vi "fly dominator.vi"() -> ()   [LabVIEW 2021]
uses:
  states.ctl
  <vilib>/Analysis/NI_AALBase.lvlib
  <vilib>/Analysis/baseanly.llb/Mean (DBL).vi
  <extravilib>/ChannelInstances/Tag-bool.lvlib
  <vilib>/DAQmx/write.llb/DAQmx Write (Digital Bool 1Line 1Point).vi
  <vilib>/DAQmx/create/channels.llb/DAQmx Create Channel (DO-Digital Output).vi
  <resource>/objmgr/daqmx.rc
  <vilib>/Waveform/WDTFileIO.llb/ Write Waveform to File.vi
  C:/FINDS_VIs/Thorlabs.MotionControl.Controls.dll
  FINDS_VIs/Thorlabs.MotionControl.Controls.dll
  C:/FINDS_VIs/Thorlabs.MotionControl.Benchtop.StepperMotorCLI.dll
  FINDS_VIs/Thorlabs.MotionControl.Benchtop.StepperMotorCLI.dll
  <vilib>/Analysis/NI_AALPro.lvlib
  0273469b-1630-426e-8888-91f9d245564e.vi
  8ea25fb4-7a89-4be8-837a-9bc05b844755.vi
  <vilib>/smtpClient/LabVIEWSMTPClient.lvlib
  a9b58a78-20d6-47fd-9184-b30837673e93.vi
  <vilib>/vision/NI_Vision_Development_Module.lvlib
  <vilib>/DAQmx/write.llb/DAQmx Write (Analog DBL 1Chan 1Samp).vi
  <vilib>/platform/TimedLoop/XDataNode/XDataNode.xnode
  <vilib>/Platform/TimedLoop/XDataNode/nitl_modes.ctl
  <vilib>/Platform/TimedLoop/XDataNode/XDNodeRunTimeDep.lvlib
  <vilib>/Platform/TimedLoop/XDataNode/wakeup.ctl
  <vilib>/Platform/TimedLoop/XDataNode/timing_clust.ctl
  <vilib>/DAQmx/read.llb/DAQmx Read (Digital Bool 1Line 1Point).vi
  <vilib>/DAQmx/create/channels.llb/DAQmx Create Channel (DI-Digital Input).vi
  <vilib>/DAQmx/create/channels.llb/DAQmx Create Channel (AO-Voltage-Basic).vi
  <vilib>/DAQmx/configure/timing.llb/DAQmx Timing (Sample Clock).vi
  <vilib>/DAQmx/create/channels.llb/DAQmx Create Channel (AI-Voltage-Basic).vi
  <vilib>/DAQmx/read.llb/DAQmx Read (Analog 1D DBL 1Chan NSamp).vi
  <vilib>/smtpClient/Set Message Text.vi
panel:
  out "Focal position":dbl
  in  "y 3":dbl
  in  "y 2":dbl
  in  "x":dbl
  in  "element 3":dbl=200.0
  in  "Focus changing \nperiod (ms)":dbl=3000.0
  out "relative seconds start":dbl format="%_19f"
  in  "4c":bool
  in  "Exposure time":dbl=0.0195
  in  "sample name":string="cance4r"
  out "Current state":string
  in  "Range 3":bool
  out "Last saved file 2":path
  out "Last saved # 2":i32
  in  "# to measure 2":i32=200
  out "Timed loop#":i32
  out "lateral position\n indexs":dbl[](array[numeric])
  out "647 2":bool
  out "647 i":bool
  in  "647?":bool
  in  "647 filter":dbl=0.2499999999999 format="%#_13g"
  in  "galvano":bool
  in  "647":bool
  in  "Slide":dbl(slide)=2.5059665871121717 scale=0.0..5.0
  out "405 2":bool
  out "488 2":bool
  out "594  2":bool
  out "532  2":bool
  in  "594 filter":dbl=0.3333333333333 format="%#_13g"
  in  "532 filter":dbl=0.4166667 format="%#_13g"
  in  "405 filter":dbl=0.16 format="%#_13g"
  in  "488 filter":dbl=0.08333333333333333 format="%#_13g"
  out "center":dbl format="%0.2f"
  in  "morphology\nthreshold":i32=40
  out "Numeric 8":i32
  in  "Setting 2":dbl=110.0
  in  "tube to stop":i32=6
  in  "maximum":i32=15
  out "larva size":bool
  out "r285":bool
  out "r216":bool
  out "Homing distance":u32
  in  "594?":bool
  in  "488?":bool
  in  "532?":bool
  in  "405?":bool
  in  "shower time":u32=20000
  in  "waiting time for\n robotic arm":u32=12000
  in  "washing time":u32=11000
  out "Boolean":bool
  out "Numeric 7":i32
  out "Numeric 6":i32
  out "Numeric 5":dbl
  out "waiting number":i32
  out "larvae in chamber?":bool
  in  "Range 2":bool
  out "4c label #":i32
  in  "batch#":string
  in  "High speed?":bool
  out "max value":i32
  out "real R2":i32
  in  "clearing date":string
  in  "laser channel":string
  in  "wait for\nclearing":bool
  in  "wait for clearing? 2":bool
  out "clear finished?":bool
  out "relative seconds 2":dbl format="%_19f"
  in  "real laser power":string
  in  "Operator":T1(ring)=enum."hanqing WANG"
  in  "max intensity threshold":i32=3500
  out "screening":bool
  in  "4000?":bool
  in  "calibration?":bool
  out "experiment time(mins)":dbl
  out "experiment stop time (relative)":dbl format="%_19f"
  in  "screening method":T2(ring)=enum."Pix count"
  in  "Count threshold":dbl
  in  "2000?":bool=TRUE
  out "Numeric 4":i32
  out "index":i32
  out "size(s)":i32
  out "Frame 2":i32
  out "mean 5":dbl format="%0.2f"
  out "mean 4":dbl format="%0.2f"
  out "Numeric 2":i32
  in  "manual loading":bool
  in  "shower time(ms)":u32=5000
  in  "BUBBLE SIZE":i32=3
  out "gp":dbl
  in  "um to move short":u32=6500
  in  "um to move long":u32=7000
  out "OK Done 4":bool
  out "homing speed":bool
  out "homing":bool
  in  "4c direction":bool=TRUE
  in  "manual 4c":bool
  out "tube changing #":i32
  in  "# BEFORE GO DOWN":i32=1
  in  "TIME THRESHOLD":dbl=40.0
  in  "force anticlogging":bool
  in  "Flow Rate (5.00)":dbl=100.0 format="%#.4f"
  in  "milliseconds to wait":u32=4000
  in  "position":dbl=0.083333
  out "#of edgehunting":u32
  in  "wavelength":string
  out "Auto-imaging time":dbl[](graph)
  in  "4c Base file name":string="brp_each"
  out "594 i":bool
  out "532 i":bool
  out "488 i":bool
  out "405 i":bool
  out "Last saved file 4c":path
  in  "BenchtopStepperControl":refnum<k24>(container)
  in  "SerialNumber":string="40227394"
  in  "Frames in memory 2":i32=800
  in  "High Speed 2":u32=10000
  out "Larva length (# frames)":i32
  in  "correction":i32=600
  out "backwards pulses":i32
  in  "scanning Speed":u32=20000 min=1 max=500000
  out "larvae size in scan":dbl[](graph)
  out "OK Done":bool
  in  "Edge-hunting Direction":bool
  in  "scanning distance (um)":u32=43000 min=1 max=500000
  in  "Main/Sub":bool
  in  "manual edgehunting":bool
  in  "Number of samples":i32=150
  out "Waveform Graph":dbl[](graph)
  out "loading tube#":i32
  in  "manual load":bool
  in  "Force move":bool
  in  "Larva # to move":i32=1000
  out "Larvae until move":i32
  in  "tb Pulses to move":u32=750 min=1 max=500000
  in  "tube Direction":bool
  in  "Save start #":i32
  out "Last saved file number 4":i32
  in  "Enable screening\n(during flow zoometry)":bool
  in  "Save base file name 2000":path=path "\\\\FINDSCTRL\\findsdata/finds2/20240321/2000test"
  in  "Acquire speed 3 (um/s)":u32=2000
  out "Last saved file 2000":path
  out "Last saved file number 2000":i32
  in  "Samples to measure 2000":i32=100
  in  "EH speed 3":bool
  out "Mean intensity\nof frame":dbl=212.9530098438263 format="%0.2f"
  in  "reverse":bool
  in  "wave trigger":dbl
  in  "Save base file name 4000":path=path "\\\\157.82.9.50\\d/20240220/gp mor/tm6b/4000/uasmcherry.tm6b.2.50w.4000"
  in  "Acquire speed 2 (um/s)":u32=4000
  out "Last saved file 4000":path
  in  "Samples to measure 4000":i32=100
  in  "EH speed 2":bool
  in  "reverse flow \nthreshold (sec)":dbl=40.0
  out "Elapsed (sec)":dbl
  in  "next loop":bool=TRUE
  out "False triggers":i32
  in  "manual imaging":bool
  in  "SampClk.Rate 2":dbl=100000.0
  in  "Physical Channel 2":tag="Dev1/ai0"
  in  "Stop Trigger stream":bool
  out "Mean":dbl format="%0.2f"
  out "Triggered":bool
  in  "Trigger":dbl=0.10000000000000009
  out "Trigger PD running mean":dbl(graph)
  out "#triggers":i32
  in  "um to move":u32=6000
  in  "488":bool
  in  "532":bool
  in  "594":bool
  in  "405":bool
  in  "START AUTO IMAGING":bool caption="Start\nauto imaging"
  in  "Continuous\nacquisition":bool
  in  "# to measure":i32=200
  out "Last saved #":i32
  out "Last saved file":path
  in  "Acquire speed (um/s)":u32=200
  in  "Movement direction":bool=TRUE
  out "Saving image":bool
  out "Moving":bool
  in  "Save directory":path=path "\\\\157.82.9.50\\d/HW/b11 cance4r"
  in  "Mean trigger":i32=170
  out "Sub img mean":dbl
  out "Sub image":u16[][](graph) caption="Image"
  in  "XS x length":i32=1000
  in  "XS x px start":i32=500
  out "READY":bool
  in  "Shut down":bool
  in  "START":bool
  out "Streaming":bool
  in  "XS y length":i32=1000
  in  "XS y px start":i32=1000
  out "Camera error out":errorcluster {"code" format="%.0x"}
  in  "Quit":bool
  out "Obtained image":u16[][](graph) caption="Image"
  out "Frame count":i32
  # "error trigger exclusion setting"
  # "NOTICE:\nplease check the state frequently\nyou have to go back to chilling state before you do any other operation"
  # "File & save settings"
  # "motion tracker"
  # "Status"
  # "Laser output\n(Chilling state updates)"
  # "Flow zoometry"
  # "Trigger"
  # "No-flow imaging"
  # "Camera streaming"
  # "Genetic screening"
  # "Acquisition settings"
  # "Auto\nfocus settings"
  # "Sucking tube settings"
  # "Manual image acquisition\n(initiate from chilling state)"
  # "down"
  # "up"
  # "Edgehunting settings"
  # "Anti-clogging settings"
  # "ROBOTIC ARM LOADING"
  # "B"
  # "F"
  # "channel selection"
types:
  T1 = enum16{"kobayashi", "Tsutsumi", "hanqing WANG", "chenglang"}
  T2 = enum16{"morphology", "Pix count", "MAX INTENSITY", "Average int"}
  T3 = enum32{"Invalid", "Standard", "Closed", "Hidden", "Minimized", "Maximized"}
  T4 = typedef "states.ctl" = enum16{"acquire without AF", "647", "Initialize", "Chilling", "4climbo", "light reverse", "wait for clearing", "manual loading", "4cini", "reverse", "2000", "4000", "screening", "tube position", "Edgehunting", "Edgehunting2", "homing", "Position_check", "antic\n", "Stream w/o flow2", "Stream w/o flow", "stopflow triggertest", "Find boundaries", "Acquire", "save", "auto imaging", "robotic arm", "Close", "594", "532", "488", "405", "4c acquirement", "Stop", "405_r"}
  T5 = enum32{"Map Pixel Pointer", "Unmap Pixel Pointer", "Get Pixels Infos"}
  T6 = typedef "XDNodeRunTimeDep.lvlib/timing_clust.ctl" = cluster{"Expected End [f-1]":u64, "Actual End [f-1]":u64, "Finished Late? [f-1]":bool, "Expected End [i-1]":u64, "Actual End [i-1]":u64, "Finished Late? [i-1]":bool, "Expected Start [i]":u64, "Actual Start [i]":u64, "Expected Start [f]":u64, "Actual Start [f]":u64, "Source Name":string, "Structure Name":string, "Period":i64, "Deadline":i64, "Offset":i64, "Start":i64, "Priority":i32, "Timeout":i32, "Mode":T7, "Wakeup Reason":T8, "Error":errorcluster, "Source Type":string, "Secondary Source Type":string, "Global End Time":u64, "Global Start Time":u64, "Frame Duration":u64, "Iteration Duration":u64, "Assigned CPU":i32, "I/O Scan Engine Mode":u32}
  T7 = typedef "XDNodeRunTimeDep.lvlib/nitl_modes.ctl" = enum32{"No Change", "Process missed periods, maintain original phase", "Discard missed periods, maintain original phase", "Process missed periods, ignore original phase", "Discard missed periods, ignore original phase"}
  T8 = typedef "XDNodeRunTimeDep.lvlib/wakeup.ctl" = enum32{"Normal", "Aborted", "Asynchronous wakeup", "Timing source error", "Timed loop error", "Timeout"}
  T9 = cluster{"Output Trigger Mode":u32, "Output Trigger Polarity":u32}
  T10 = cluster{"Output Trigger Period":dbl, "Delay":dbl, "Source":u32}
  T11 = typedef "Image Type" = u32
  T12 = typedef "IMAQ Image.ctl" = refnum<image>
  T13 = typedef "Tag-bool.lvlib/))Channel.ctl" = refnum<queue>
  T14 = typedef "LabVIEWSMTPClient.lvlib/SmtpClientHandle.ctl" = refnum<k1>
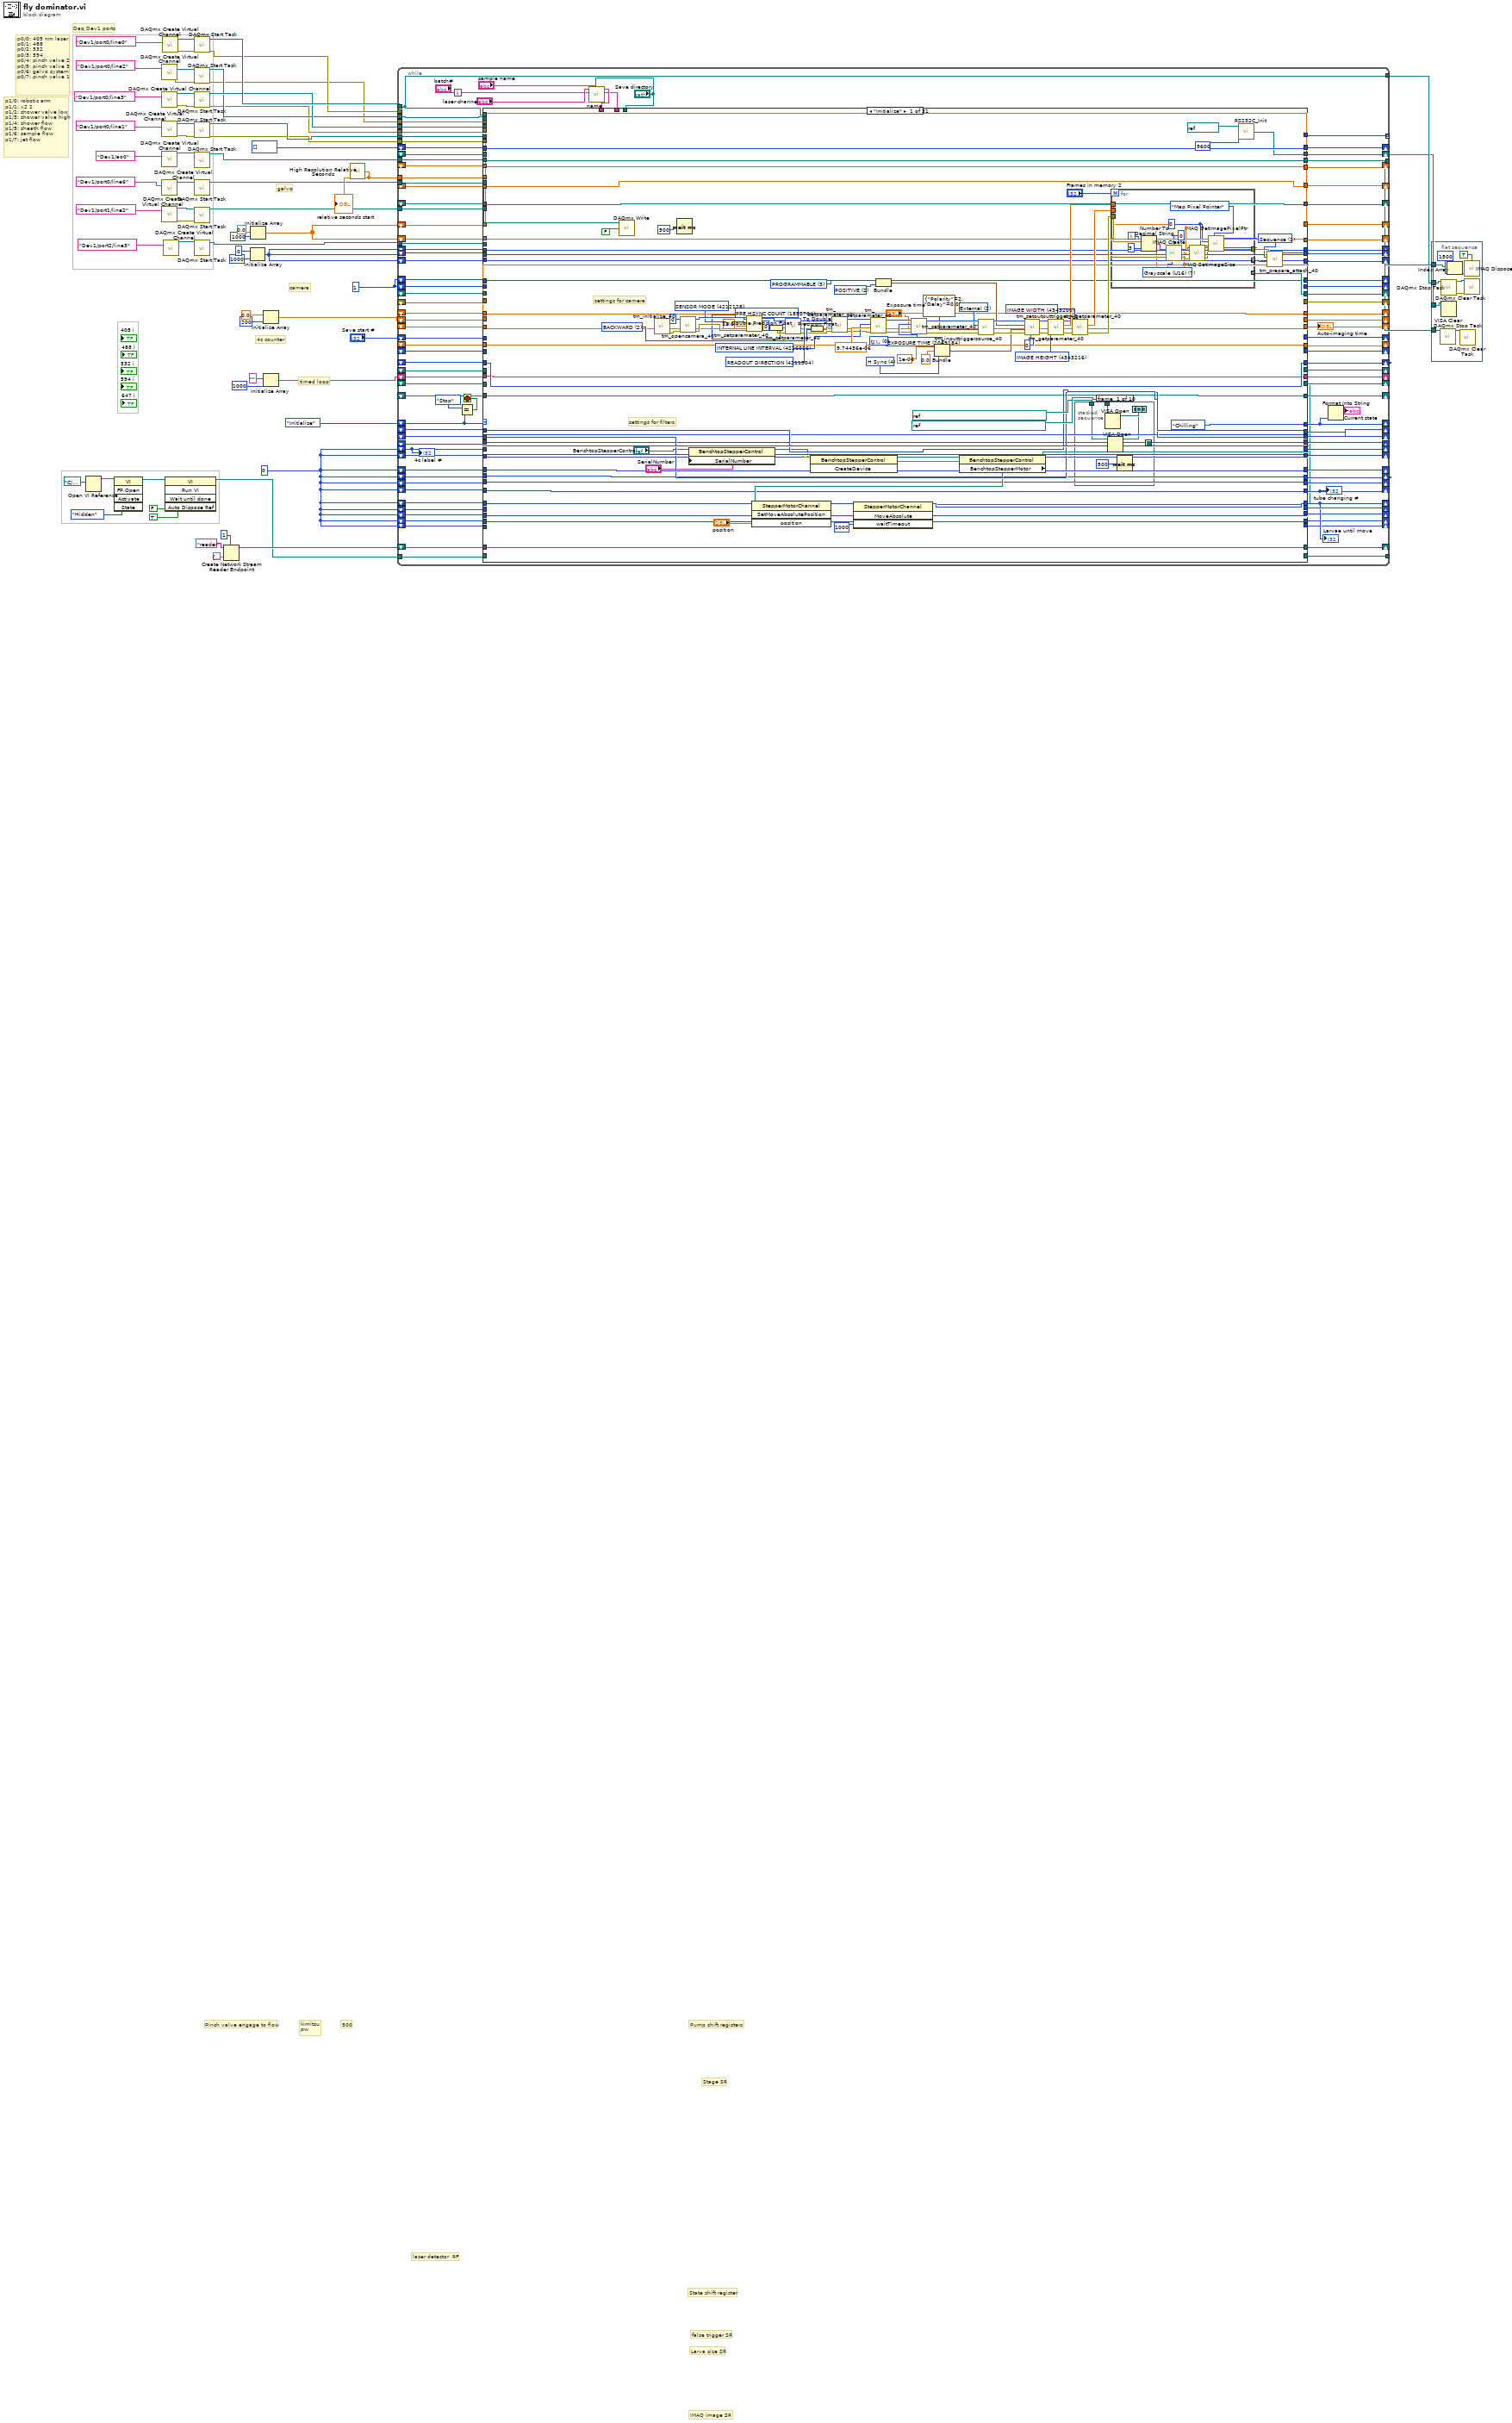
[diagram p0: block diagram]
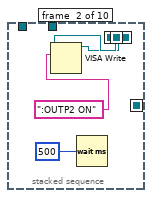
[diagram p2: hidden frame]
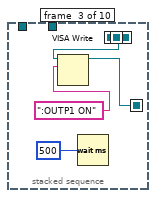
[diagram p3: hidden frame]
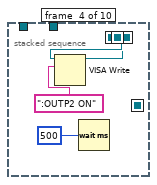
[diagram p4: hidden frame]
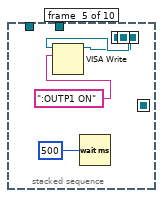
[diagram p5: hidden frame]
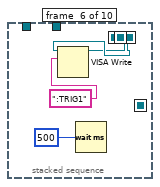
[diagram p6: hidden frame]
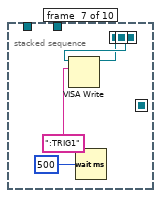
[diagram p7: hidden frame]
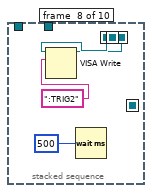
[diagram p8: hidden frame]
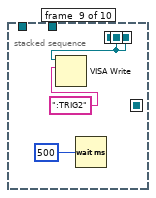
[diagram p9: hidden frame]
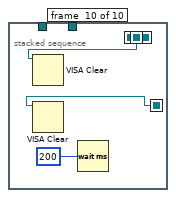
[diagram p10: hidden frame]
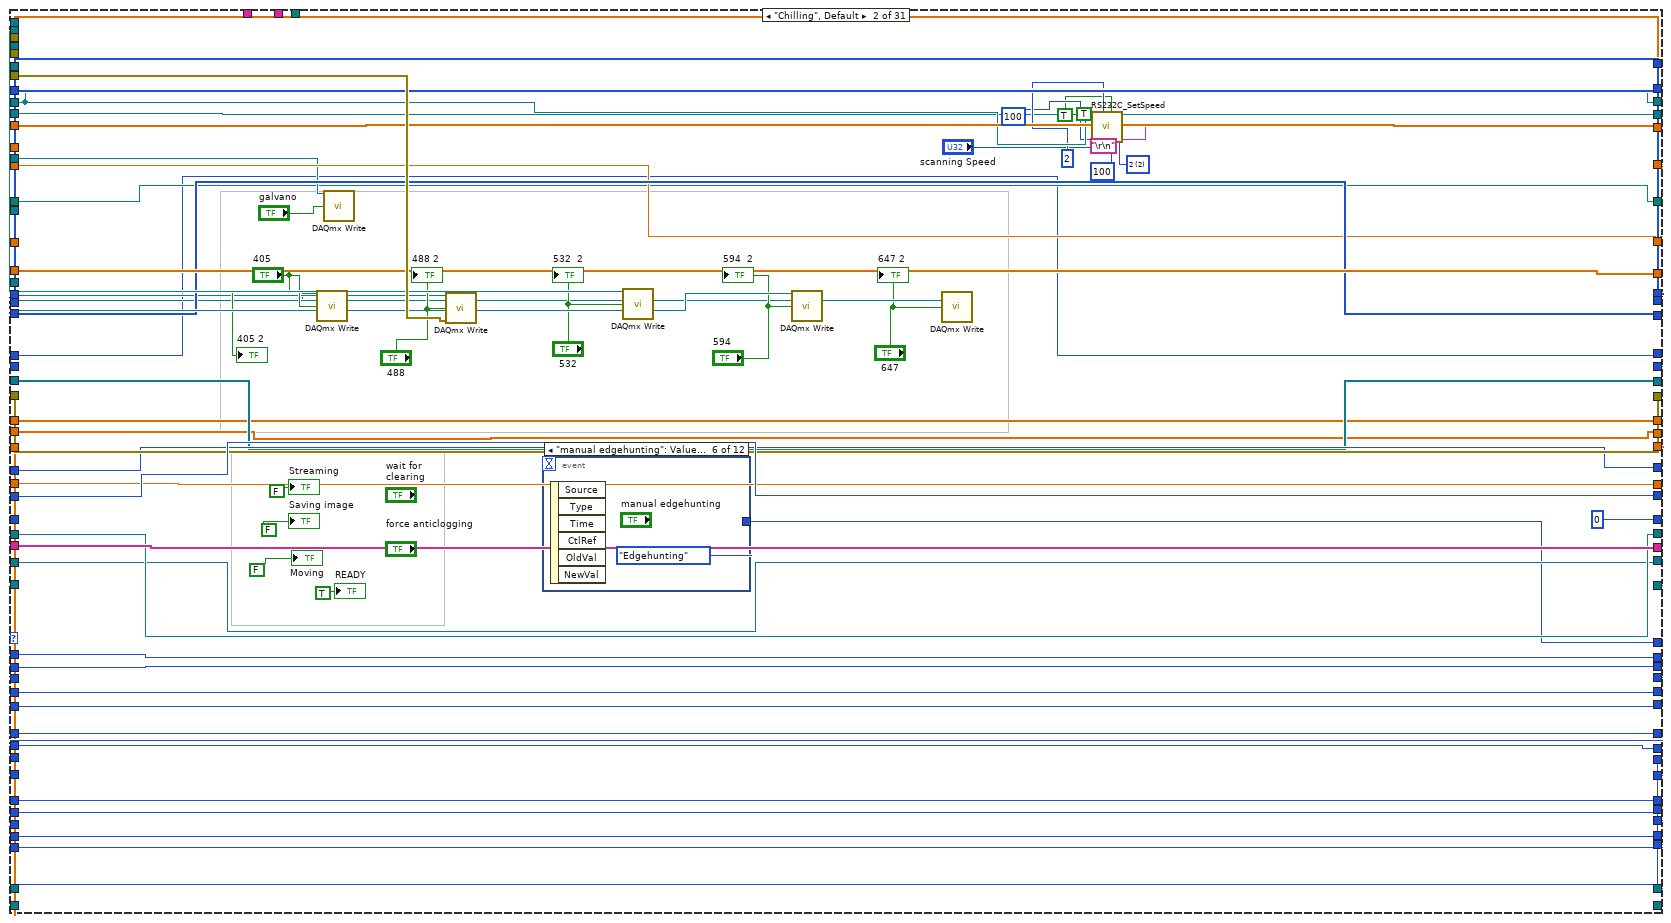
[diagram p11: hidden frame]
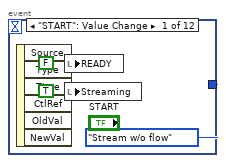
[diagram p12: hidden frame]
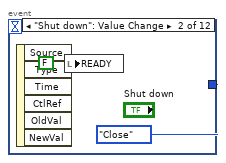
[diagram p13: hidden frame]
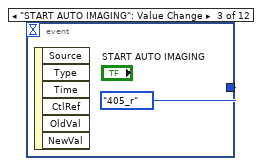
[diagram p14: hidden frame]
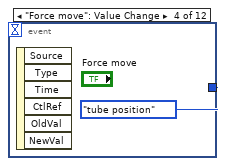
[diagram p15: hidden frame]
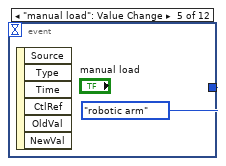
[diagram p16: hidden frame]
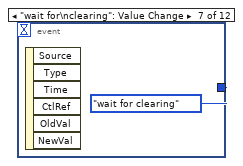
[diagram p17: hidden frame]
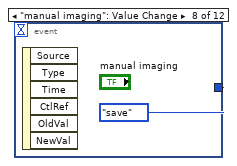
[diagram p18: hidden frame]
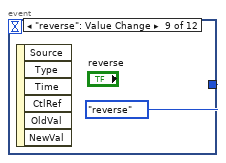
[diagram p19: hidden frame]
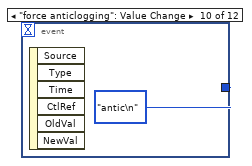
[diagram p20: hidden frame]
diagram:
  w4 = 1
  w5 = 0
  # "p0/0: 405 nm laser \np0/1: 488\np0/2: 532\np0/3: 594\np0/4: pinch valve 2\np0/5: pinch valve 3\np0/6: galvo system \np0/7: pinch valve 1"
  # "p1/0: robotic arm\np1/1: v2 2\np1/2: shower valve low\np1/3: shower valve high\np1/4: shower flow\np1/5: sheath flow\np1/6: sample flow\np1/7: jet flow"
  # "timed loop"
  # "Daq Dev1 ports"
  # "galvo"
  # "4c counter"
  # "500"
  # "false trigger SR"
  # "camera"
  # "kimitsu\npw"
  # "laser detector  RF"
  # "IMAQ image SR"
  # "Larva size SR"
  # "Stage SR"
  # "Pinch valve engage to flow"
  # "State shift register"
  # "Pump shift registers"
  n1 = Open VI Reference(vi path=path "C:/FINDS_VIs/Abyss-watcher_love-edition.vi") -> (vi reference=w27:refnum<vi>)  [unwired: 5 in, 1 out]
  n2 = invoke class="VI" method="FP.Open"(reference=w27, "State"=T3."Hidden") -> (reference out=w25:refnum<vi>)  [unwired: 3 in, 4 out]
  n3 = call-poly <vilib>:"DAQmx Create Virtual Channel.vi"("lines"=tag "Dev1/port0/line2") -> ("task out"=w49:refnum<k21>, "error out"=w58:errorcluster)  [unwired: 13 in]
  n4 = call-poly <vilib>:"DAQmx Create Virtual Channel.vi"("lines"=tag "Dev1/port0/line3") -> ("task out"=w52:refnum<k21>, "error out"=w56:errorcluster)  [unwired: 13 in]
  n5 = call-poly <vilib>:"DAQmx Create Virtual Channel.vi"("lines"=tag "Dev1/port0/line1") -> ("task out"=w61:refnum<k21>, "error out"=w54:errorcluster)  [unwired: 13 in]
  n6 = call-poly <vilib>:"DAQmx Create Virtual Channel.vi"("physical channels"=tag "Dev1/ao0") -> ("task out"=w12:refnum<k21>)  [unwired: 13 in, 1 out]
  n7 = call-poly <vilib>:"DAQmx Create Virtual Channel.vi"("lines"=tag "Dev1/port0/line6") -> ("task out"=w9:refnum<k21>)  [unwired: 13 in, 1 out]
  n8 = call-poly <vilib>:"DAQmx Create Virtual Channel.vi"("lines"=tag "Dev1/port1/line2") -> ("task out"=w33:refnum<k21>, "error out"=w31:errorcluster)  [unwired: 13 in]
  n9 = call-poly <vilib>:"DAQmx Create Virtual Channel.vi"("lines"=tag "Dev1/port0/line0") -> ("task out"=w65:refnum<k21>, "error out"=w64:errorcluster)  [unwired: 13 in]
  n10 = call-poly <vilib>:"DAQmx Create Virtual Channel.vi"("lines"=tag "Dev1/port2/line3") -> ("task out"=w17:refnum<k21>)  [unwired: 13 in, 1 out]
  n11 = invoke class="VI" method="Run VI"(reference=w25, "Wait until done"=FALSE ("Wait Until Done"), "Auto Dispose Ref"=TRUE ("Auto Dispose Reference")) -> (reference out=w3:refnum<vi>)  [unwired: 2 in, 4 out]
  n12 = call <vilib>:"DAQmx Start Task.vi"("task/channels in"=w49, "error in"=w58) -> ("task out"=w50:refnum<k21>, "error out"=w43:errorcluster)  [unwired: 12 in]
  n13 = call <vilib>:"DAQmx Start Task.vi"("task/channels in"=w52, "error in"=w56) -> ("task out"=w51:refnum<k21>, "error out"=w42:errorcluster)  [unwired: 12 in]
  n14 = call <vilib>:"DAQmx Start Task.vi"("task/channels in"=w61, "error in"=w54) -> ("task out"=w59:refnum<k21>, "error out"=w53:errorcluster)  [unwired: 12 in]
  n15 = call <vilib>:"DAQmx Start Task.vi"("task/channels in"=w12) -> ("task out"=w11:refnum<k21>)  [unwired: 13 in, 1 out]
  n16 = call <vilib>:"DAQmx Start Task.vi"("task/channels in"=w9) -> ("task out"=w8:refnum<k21>)  [unwired: 13 in, 1 out]
  n17 = call <vilib>:"DAQmx Start Task.vi"("task/channels in"=w65, "error in"=w64) -> ("task out"=w62:refnum<k21>, "error out"=w48:errorcluster)  [unwired: 12 in]
  n18 = call <vilib>:"DAQmx Start Task.vi"("task/channels in"=w33, "error in"=w31) -> ("task out"=w30:refnum<k21>)  [unwired: 12 in, 1 out]
  n19 = call <vilib>:"DAQmx Start Task.vi"("task/channels in"=w17) -> ("task out"=w16:refnum<k21>)  [unwired: 13 in, 1 out]
  n20 = Create Network Stream Reader Endpoint(7:1 ("reader buffer size"), 9:cluster{dbl, bool} {0.0, TRUE}, 11:"reader" ("reader name")) -> (3:w20:refnum<k21>)  [unwired: 4 in, 1 out]
  n21 = Initialize Array(i16 0 ("element"), 1000 ("dimension size")) -> (w1:i16[])
  n22 = Initialize Array(0.0 ("element"), 1000 ("dimension size")) -> (w7:dbl[])
  n23 = Initialize Array("", 1000 ("dimension size")) -> (w44:string[])
  n24 = Initialize Array(0.0 ("element"), 200 ("dimension size")) -> (w6:dbl[])
  n25 = call <vilib>:"High Resolution Relative Seconds.vi"() -> ("relative seconds"=w36:dbl)
  "relative seconds start" <- w36
  n26 = while {
    shift-right: [w73] -> _
    shift-left: states."Initialize" -> [w173]
    shift-right: [w170] -> _
    shift-left: _ -> [w168]
    shift-right: [w169] -> _
    shift-left: _ -> [w167]
    shift-right: [w165] -> _
    shift-left: "Save start #" -> [w166]
    shift-right: [w164] -> _
    shift-left: _ -> [w163]
    shift-right: [w98] -> w29
    shift-left: _ -> [w162]
    shift-right: [w161] -> _
    shift-left: _ -> [w160]
    shift-right: [w159] -> w47
    shift-left: _ -> [w158]
    tunnel: w62 -> [w107]
    tunnel: w59 -> [w157]
    tunnel: w53 -> [w156]
    tunnel: w51 -> [w154]
    tunnel: w50 -> [w155]
    tunnel: [w107] -> w37
    tunnel: w48 -> [_]
    shift-right: [w152] -> _
    shift-left: w5 -> [w153]
    shift-right: [w132] -> _
    shift-left: w7 -> [w151]
    shift-right: [w111] -> _
    shift-left: w6 -> [w150]
    shift-right: [w148] -> _
    shift-left: w44 -> [w149]
    shift-right: [w146] -> _
    shift-left: w5 -> [w147]
    shift-right: [w144] -> _
    shift-left: i32[] [] -> [w145]
    shift-right: [w142] -> _
    shift-left: w1 -> [w143]
    shift-right: [w131] -> _
    shift-left: _ -> [w141]
    shift-right: [w139] -> _
    shift-left: w4 -> [w140]
    shift-right: [w137] -> _
    shift-left: w1 -> [w138]
    tunnel: w43 -> [w136]
    tunnel: w42 -> [w135]
    shift-right: [w133] -> _
    shift-left: w1 -> [w134]
    shift-right: [w129] -> _
    shift-left: w4 -> [w130]
    shift-right: [w127] -> _
    shift-left: w5 -> [w128]
    shift-right: [w126] -> _
    shift-left: w5 -> [w125]
    tunnel: [w124] -> _ mode=indexing
    shift-right: [w122] -> _
    shift-left: w5 -> [w123]
    shift-right: [w87] -> _
    shift-left: _ -> [w119]
    shift-right: [w121] -> _
    shift-left: _ -> [w117]
    shift-right: [w120] -> _
    shift-left: _ -> [w118]
    shift-right: [w116] -> _
    shift-left: _ -> [w114]
    shift-right: [w115] -> _
    shift-left: _ -> [w75]
    tunnel: w36 -> [w113]
    shift-right: [w110] -> _
    shift-left: w6 -> [w112]
    shift-right: [w108] -> _
    shift-left: w5 -> [w109]
    tunnel: w30 -> [w106]
    tunnel: [w105] -> _
    shift-right: [w103] -> _
    shift-left: w5 -> [w104]
    shift-right: [w101] -> _
    shift-left: w5 -> [w102]
    shift-right: [w99] -> _
    shift-left: w6 -> [w100]
    shift-right: [w96] -> _
    shift-left: w5 -> [w97]
    shift-right: [w95] -> _
    shift-left: w20 -> [w94]
    tunnel: w3 -> [w93]
    shift-right: [w91] -> _
    shift-left: w5 -> [w92]
    shift-right: [w90] -> _
    shift-left: _ -> [w89]
    tunnel: w16 -> [w88]
    shift-right: [w85] -> _
    shift-left: w7 -> [w86]
    shift-right: [w83] -> _
    shift-left: w5 -> [w84]
    tunnel: w11 -> [w82]
    tunnel: [w81] -> w13
    tunnel: w8 -> [w80]
    shift-right: [w79] -> _
    shift-left: _ -> [w78]
    shift-right: [w77] -> _
    shift-left: _ -> [w76]
    stop <- w172 stop-if-true
    n27 = Equal?(x=w173, y=states."Stop") -> (x = y?=w172:bool)
    n28 = call "name.vi"("sample name"="sample name", "Save directory"="Save directory", "batch#"="batch#", "laser channel"="laser channel") -> ("time stamp"=w72:string, "file naming"=w71:string)  [unwired: 5 in, 1 out]
    n29 = case shown="\"Initialize\"" w173 {
      tunnel: [w232 w413 w482 w535 w630 w969 w1057 w1355 w1471 w1591 w1885 w1969 w2219 w2397 w2602 w2848 w3081 w3281 w3349 w3417 w3486 w3548 w3616 w3684 w3734 w3827 w4035 w4186 w4447 u32 0 ("Handle out") u32 0 ("Handle out")] -> w170
      tunnel: [w235 w412 w481 w536 w632 w968 w1056 w1354 w1470 w1590 w1884 w1967 w2218 w2396 w2600 w2846 w3079 w3280 w3348 w3416 w3485 w3547 w3615 w3683 w3733 w3826 w4034 w4185 w4446 errorcluster {"status"=FALSE, "code"=0, "source"=""} ("error out") errorcluster {"status"=FALSE, "code"=0, "source"=""} ("error out")] -> w169
      tunnel: [states."Chilling" w367 w451 states."Chilling" w633 w952 w1045 w1328 w1444 w1546 w1814 w2032 w2193 w2398 states."acquire without AF" w2880 w3110 w3247 w3315 w3383 w3453 w3514 w3582 w3650 w3701 w3859 w4042 w4151 w4454 states."Stop" states."Stop"] -> w73
      tunnel: w168 -> [_ w413 w482 w497 w630 w969 w1057 w1355 w1471 w1591 w1885 w1974 w2219 w2397 w2643 w2890 w3120 w3281 w3349 w3417 w3486 w3548 w3616 w3684 w3734 w3870 w4055 w4186 w4466 w4628 _]
      tunnel: w167 -> [_ w412 w481 w533 w632 w968 w1056 w1354 w1470 w1590 w1884 w1973 w2218 w2396 w2644 w2891 w3121 w3280 w3348 w3416 w3485 w3547 w3615 w3683 w3733 w3871 w4056 w4185 w4467 w4627 _]
      tunnel: w166 -> [w245 w411 w480 w540 w634 w967 w1055 w1353 w1469 w1589 w1883 w1938 w2217 w2395 w2556 w2788 w3032 w3279 w3347 w3415 w3484 w3546 w3614 w3682 w3732 w3815 w3995 w4184 w4405 w4623 w4729]
      tunnel: [w245 w411 w480 w540 w634 w967 w1055 w1353 w1469 w1589 w1883 w1938 w2217 w2395 w2612 w2788 w3031 w3279 w3347 w3415 w3484 w3546 w3614 w3682 w3732 w3814 w3995 w4184 w4405 w4623 w4729] -> w165
      tunnel: [w179 w410 w432 w539 w576 w925 w984 w1291 w1407 w1517 w1807 w1958 w2170 w2353 w2642 w2889 w3119 w3227 w3296 w3364 w3431 w3494 w3563 w3631 w3692 w3869 w4054 w4141 w4465 refnum<visa-resource-name> refnum ("VISA resource name out") refnum<visa-resource-name> refnum ("VISA resource name out")] -> w164
      tunnel: w163 -> [w179 w410 w432 w539 w576 w925 w984 w1291 w1407 w1517 w1807 w1958 w2170 w2353 w2642 w2889 w3119 w3227 w3296 w3364 w3431 w3494 w3563 w3631 w3692 w3869 w4054 w4141 w4465 _ _]
      tunnel: [w206 w388 w479 w538 w631 w966 w1044 w1352 w1468 w1588 w1882 w2017 w2199 w2371 w2631 w2876 w3107 w3278 w3346 w3414 w3483 w3545 w3613 w3681 w3731 w3856 w4037 w4183 w4449 w4621 w4727] -> w98
      tunnel: w162 -> [_ w388 w479 w538 w631 w966 w1044 w1352 w1468 w1588 w1882 w2031 w2201 w2371 w2641 w2888 w3118 w3278 w3346 w3414 w3483 w3545 w3613 w3681 w3731 w3868 w4053 w4183 w4464 w4621 w4727]
      tunnel: [w224 u32 0 w478 w528 w625 w965 w1036 w1351 w1467 w1587 w1881 w2044 w2216 w2400 w2618 w2863 w3095 w3277 w3345 w3413 w3482 w3544 w3612 w3680 w3730 w3845 w4021 w4182 w4386 w4616 w4723] -> w161
      tunnel: w160 -> [w224 _ w478 w528 w625 w965 w1036 w1351 w1467 w1587 w1881 w2044 w2216 w2400 w2618 w2863 w3095 w3277 w3345 w3413 w3482 w3544 w3612 w3680 w3730 w3845 w4021 w4182 w4386 w4616 w4723]
      tunnel: "Save directory" -> [_ _ _ _ _ _ _ _ _ _ _ w1935 _ _ w2529 w2882 w3111 _ _ _ _ _ _ _ _ w3861 _ _ _ _ _]
      tunnel: [w229 w408 w477 w532 w629 w964 w1054 w1350 w1466 w1586 w1880 w2021 w2215 w2344 w2629 w2874 w3105 w3276 w3344 w3412 w3481 w3543 w3611 w3679 w3729 w3853 w4032 w4181 w4444 w4620 w4664] -> w159
      tunnel: w158 -> [_ w408 w477 w534 w629 w964 w1054 w1350 w1466 w1586 w1880 w2026 w2215 w2344 w2629 w2874 w3105 w3276 w3344 w3412 w3481 w3543 w3611 w3679 w3729 w3853 w4032 w4181 w4444 w4620 w4664]
      tunnel: w157 -> [_ w349 _ _ _ _ _ _ _ _ _ _ _ _ _ _ _ w3253 w3321 w3389 w3459 w3520 w3588 w3656 w3697 _ _ _ _ w4606 w4715]
      tunnel: w156 -> [_ w407 _ _ _ _ _ _ _ _ _ _ _ _ _ _ _ _ _ _ _ _ _ _ _ _ _ _ _ _ w4714]
      tunnel: w155 -> [_ w406 _ _ _ _ _ _ _ _ _ _ _ _ _ _ _ w3252 w3320 w3388 w3458 w3519 w3587 w3655 w3696 _ _ _ _ w4607 w4713]
      tunnel: w154 -> [_ w405 _ _ _ _ _ _ _ _ _ _ _ _ _ _ _ w3251 w3319 w3387 w3457 w3518 w3586 w3654 w3695 _ _ _ _ w4605 w4712]
      tunnel: w153 -> [w227 w401 w476 w531 w628 w963 w1053 w1349 w1465 w1585 w1879 w2043 w2214 w2394 w2616 w2861 w3093 w3275 w3343 w3411 w3480 w3542 w3610 w3678 w3728 w3843 w4019 w4180 w4431 w4619 w4726]
      tunnel: [w227 w401 w476 w531 w628 w963 w1053 w1349 w1465 w1585 w1879 w2043 w2214 w2393 w2616 w2861 w3093 w3275 w3343 w3411 w3480 w3542 w3610 w3678 w3728 w3843 w4019 w4180 w4431 w4619 w4726] -> w152
      tunnel: [w226 w400 w475 w530 w627 w962 w1052 w1348 w1464 w1584 w1878 w2042 w2213 w2392 w2597 w2843 w3072 w3274 w3342 w3410 w3479 w3541 w3609 w3677 w3727 w3832 w3977 w4179 w4403 w4618 w4725] -> w132
      tunnel: w151 -> [w226 w400 w475 w530 w627 w962 w1052 w1348 w1464 w1584 w1878 w2042 w2213 w2392 w2597 w2843 w3072 w3274 w3342 w3410 w3479 w3541 w3609 w3677 w3727 w3832 w3979 w4179 w4403 w4618 w4725]
      tunnel: w150 -> [w225 w399 w474 w529 w626 w961 w1051 w1347 w1463 w1583 w1877 w2009 w2212 w2391 w2596 w2842 w3071 w3273 w3341 w3409 w3478 w3540 w3608 w3676 w3726 w3831 w3984 w4178 w4429 w4617 w4724]
      tunnel: [w225 w399 w474 w529 w626 w961 w1051 w1347 w1463 w1583 w1877 w2008 w2212 w2391 w2596 w2842 w3071 w3273 w3341 w3409 w3478 w3540 w3608 w3676 w3726 w3831 w3984 w4178 w4428 w4617 w4724] -> w111
      tunnel: w149 -> [w223 w398 w473 w527 w623 w960 w1038 w1346 w1462 w1582 w1876 w2041 w2211 w2390 w2615 w2860 w3092 w3272 w3340 w3408 w3477 w3539 w3607 w3675 w3725 w3842 w4013 w4177 w4420 w4615 w4722]
      tunnel: w72 -> [_ _ _ _ _ _ _ _ _ _ _ _ _ _ w2614 w2859 w3091 _ _ _ _ _ _ _ _ w3841 w4017 _ w4426 _ _]
      tunnel: [w223 w398 w473 w527 w623 w960 w1038 w1346 w1462 w1582 w1876 w2041 w2211 w2390 w2613 w2858 w3090 w3272 w3340 w3408 w3477 w3539 w3607 w3675 w3725 w3840 w4013 w4177 w4420 w4615 w4722] -> w148
      tunnel: w147 -> [w222 w397 w472 w526 w622 w959 w1037 w1345 w1461 w1581 w1875 w2040 w2210 w2389 _ _ _ w3271 w3339 w3407 w3476 w3538 w3606 w3674 w3724 w3820 _ w4176 _ w4614 w4721]
      tunnel: [w222 w397 w472 w526 w622 w959 w979 w1345 w1461 w1581 w1875 w2040 w2210 w2389 0 0 0 w3271 w3339 w3407 w3476 w3538 w3606 w3674 w3724 w3820 0 w4176 0 w4614 w4721] -> w146
      tunnel: w145 -> [w221 w396 w471 w525 w621 w958 w1033 w1344 w1460 w1580 w1874 w2039 w2209 w2388 w2611 w2857 w3089 w3270 w3338 w3406 w3475 w3537 w3605 w3673 w3723 w3839 w4016 w4175 w4425 w4613 w4720]
      tunnel: [w221 w396 w471 w525 w621 w958 w1033 w1344 w1460 w1580 w1874 w2039 w2209 w2388 w2611 w2857 w3089 w3270 w3338 w3406 w3475 w3537 w3605 w3673 w3723 w3839 w4016 w4175 w4425 w4613 w4720] -> w144
      tunnel: w143 -> [w220 w395 w470 w524 w620 w957 w1032 w1343 w1459 w1579 w1873 w1993 w2208 w2387 _ _ _ w3269 w3337 w3405 w3474 w3536 w3604 w3672 w3722 _ w4014 w4174 w4421 w4612 w4719]
      tunnel: [w220 w395 w470 w524 w620 w957 w1032 w1343 w1459 w1579 w1873 w1993 w2208 w2387 i16[] [] i16[] [] i16[] [] w3269 w3337 w3405 w3474 w3536 w3604 w3672 w3722 w3821 w4014 w4174 w4421 w4612 w4719] -> w142
      tunnel: [w219 w394 w469 w523 w619 w956 w1031 w1342 w1458 w1578 w1872 w2038 w2207 w2386 w2610 w2856 w3088 w3268 w3336 w3404 w3473 w3535 w3603 w3671 w3721 w3838 w3986 w4173 w4422 w4611 w4718] -> w131
      tunnel: w141 -> [w219 w394 w469 w523 w619 w956 w1031 w1342 w1458 w1578 w1872 w2038 w2207 w2386 w2610 w2856 w3088 w3268 w3336 w3404 w3473 w3535 w3603 w3671 w3721 w3838 w3986 w4173 _ w4611 w4718]
      tunnel: w140 -> [w218 w393 w468 w522 w618 w937 w1030 w1341 w1457 w1577 w1871 w2037 w2206 w2385 w2609 w2855 w3087 w3267 w3335 w3403 w3472 w3534 w3602 w3670 w3720 w3837 w3996 w4172 w4393 w4604 w4717]
      tunnel: [w218 w393 w468 w522 w618 w937 w1030 w1341 w1457 w1577 w1871 w2037 w2206 w2385 w2609 w2855 w3087 w3267 w3335 w3403 w3472 w3534 w3602 w3670 w3720 w3837 w3980 w4172 w4393 w4604 w4717] -> w139
      tunnel: w138 -> [w217 w392 w467 w521 w617 w955 w1029 w1340 w1456 w1576 w1870 w2036 w2198 w2384 w2608 w2854 w3086 w3266 w3334 w3402 w3471 w3533 w3601 w3669 w3719 w3821 w3994 w4171 w4399 w4603 w4716]
      tunnel: [w217 w392 w467 w521 w617 w955 w1029 w1340 w1456 w1576 w1870 w2036 w2198 w2384 w2608 w2854 w3086 w3266 w3334 w3402 w3471 w3533 w3601 w3669 w3719 w3821 w3993 w4171 w4399 w4603 w4716] -> w137
      tunnel: w136 -> [_ _ _ _ _ _ _ _ _ _ _ _ _ _ _ _ _ _ _ _ _ _ _ _ _ _ _ _ _ _ w4701]
      tunnel: w135 -> [_ _ _ _ _ _ _ _ _ _ _ _ _ _ _ _ _ _ _ _ _ _ _ _ _ _ _ _ _ _ w4698]
      tunnel: [w216 w391 w466 w520 w616 w954 w1028 w1339 w1455 w1575 w1869 w2035 w2205 w2383 w2607 w2853 w3085 w3265 w3333 w3401 w3470 w3532 w3600 w3668 w3718 w3836 w3987 w4170 w4401 w4602 w4696] -> w133
      tunnel: w134 -> [w216 w391 w466 w520 w616 w954 w1028 w1339 w1455 w1575 w1869 w2035 w2205 w2383 w2607 w2853 w3085 w3265 w3333 w3401 w3470 w3532 w3600 w3668 w3718 w3836 w3987 w4170 w4400 w4602 w4696]
      tunnel: w130 -> [w215 w348 w465 w519 w615 w953 w1027 w1338 w1454 w1574 w1868 w2034 w2204 w2362 w2606 w2852 w3084 w3264 w3332 w3400 w3469 w3531 w3599 w3667 w3717 w3835 w3985 w4169 w4369 w4601 w4695]
      tunnel: [w215 w348 w465 w519 w615 w953 w1027 w1338 w1454 w1574 w1868 w2034 w2204 w2362 w2606 w2852 w3084 w3264 w3332 w3400 w3469 w3531 w3599 w3667 w3717 w3835 w3985 w4169 w4370 w4601 w4695] -> w129
      tunnel: w71 -> [_ _ _ _ _ _ _ _ _ _ _ _ _ _ w2604 w2850 _ _ _ _ _ _ _ _ _ w3823 _ _ _ _ w4674]
      tunnel: w128 -> [w211 w390 w464 w518 w614 w933 w1003 w1337 w1453 _ w1867 w2033 w2203 w2382 w2594 w2789 w3068 w3263 w3331 w3399 w3468 w3530 w3598 w3666 w3716 w3817 w3976 w4168 w4388 w4586 w4694]
      tunnel: [w211 w390 w464 w518 w614 w933 w1003 w1337 w1453 0 ("Larva # to move") w1867 w2033 w2203 w2382 w2593 w2789 w3067 w3263 w3331 w3399 w3468 w3530 w3598 w3666 w3716 w3817 w3976 w4168 w4388 w4586 w4694] -> w127
      tunnel: [w210 w389 w463 w517 w613 w950 w1002 w1336 w1452 w1573 w1866 w2001 w2202 w2381 w2591 w2840 w3066 w3262 w3330 w3398 w3467 w3529 w3597 w3665 w3715 w3816 w3975 w4167 w4387 w4585 w4693] -> w126
      tunnel: w125 -> [w210 w389 w463 w517 w612 w950 w1002 w1336 w1452 w1573 w1866 w2001 w2202 w2381 w2591 w2840 w3066 w3262 w3330 w3398 w3467 w3529 w3597 w3665 w3715 w3816 w3975 w4167 w4387 w4585 w4693]
      tunnel: [_ _ _ _ w611 _ _ _ _ _ _ _ _ _ _ _ _ _ _ _ _ _ _ _ _ _ _ _ _ _ _] -> w124
      tunnel: w123 -> [w187 w369 w462 w507 w583 w934 w992 w1301 w1418 w1545 w1865 w1995 w2188 w2369 w2566 w2814 w3043 w3236 w3305 w3372 w3446 w3502 w3571 w3639 w3714 w3804 w3965 w4166 w4376 w4575 w4683]
      tunnel: [w187 w369 w462 w507 w583 w934 w992 w1301 w1418 w1524 w1865 w1995 w2188 w2369 w2566 w2814 w3043 w3236 w3305 w3372 w3446 w3502 w3571 w3639 w3714 w3804 w3965 w4166 w4376 w4575 w4683] -> w122
      tunnel: [w208 w380 w461 w515 w608 w948 w1000 w1335 w1451 w1543 w1864 w2019 w2200 w2361 w2585 w2834 w3038 w3261 w3329 w3397 w3466 w3528 w3596 w3664 w3713 w3812 w3973 w4165 w4384 w4583 w4691] -> w87
      tunnel: [w207 w379 w460 w514 w607 w947 w999 w1334 w1450 w1542 w1863 w2018 w2197 w2379 w2584 w2833 w3061 w3260 w3328 w3396 w3465 w3527 w3595 w3663 w3712 w3811 w3972 w4164 w4383 w4582 w4690] -> w121
      tunnel: [w209 w381 w459 w516 w609 w949 w1001 w1333 w1449 w1544 w1862 w2013 w2196 w2380 w2586 w2835 w3041 w3259 w3327 w3395 w3464 w3526 w3594 w3662 w3711 w3813 w3974 w4163 w4385 w4584 w4692] -> w120
      tunnel: w119 -> [w209 w381 w459 w516 w609 w949 w1001 w1333 w1449 w1544 w1862 _ w2196 w2380 w2586 w2835 w3041 w3259 w3327 w3395 w3464 w3526 w3594 w3662 w3711 w3813 w3974 w4163 w4385 w4584 w4692]
      tunnel: w118 -> [w208 w380 w461 w515 w608 w948 w1000 w1335 w1451 w1543 w1864 _ w2200 w2361 w2585 w2834 w3038 w3261 w3329 w3397 w3466 w3528 w3596 w3664 w3713 w3812 w3973 w4165 w4384 w4583 w4691]
      tunnel: w117 -> [w207 w379 w460 w514 w607 w947 w999 w1334 w1450 w1542 w1863 _ w2197 w2379 w2584 w2833 w3061 w3260 w3328 w3396 w3465 w3527 w3595 w3663 w3712 w3811 w3972 w4164 w4383 w4582 w4690]
      tunnel: [w197 w376 w458 w513 w606 w946 w998 w1332 w1448 w1541 w1861 w2011 w2195 w2378 w2582 w2831 w3056 w3258 w3326 w3394 w3463 w3525 w3593 w3661 w3710 w3810 w3971 w4162 w4382 w4581 w4689] -> w116
      tunnel: [w192 w375 w457 w512 w605 w945 w997 w1331 w1447 w1540 w1860 w2010 w2194 w2377 w2581 w2830 w3050 w3249 w3317 w3385 w3455 w3516 w3584 w3652 w3709 w3809 w3970 w4161 w4381 w4580 w4688] -> w115
      tunnel: w114 -> [_ w376 w458 w513 w606 w946 w998 w1332 w1448 w1541 w1861 w2011 w2195 w2378 w2582 w2831 w3056 w3258 w3326 w3394 w3463 w3525 w3593 w3661 w3710 w3810 w3971 w4162 w4382 w4581 w4689]
      tunnel: w75 -> [_ w375 w457 w512 w605 w945 w997 w1331 w1447 w1540 w1860 w2010 w2194 w2377 w2581 w2830 w3050 w3250 w3318 w3386 w3456 w3517 w3585 w3653 w3709 w3809 w3970 w4161 w4381 w4580 w4688]
      tunnel: w107 -> [_ w347 _ _ _ _ _ _ _ _ _ _ _ _ _ _ _ w3254 w3322 w3390 w3460 w3521 w3589 w3657 w3698 _ _ _ _ _ _]
      tunnel: w113 -> [_ _ _ _ _ _ _ _ _ _ _ _ _ _ _ _ _ _ _ _ _ _ _ _ _ _ _ _ _ _ _]
      tunnel: w112 -> [w196 w374 w456 w511 w604 w944 w996 w1330 w1446 w1539 w1859 w2005 w2192 w2376 w2580 w2829 w3049 w3242 w3310 w3378 w3451 w3508 w3577 w3645 w3708 w3808 w3969 w4160 w4380 w4579 w4687]
      tunnel: [w196 w374 w456 w511 w602 w944 w996 w1330 w1446 w1539 w1859 w2005 w2192 w2376 w2580 w2829 w3049 w3242 w3310 w3378 w3451 w3508 w3577 w3645 w3708 w3808 w3969 w4160 w4380 w4579 w4687] -> w110
      tunnel: w109 -> [w190 w373 w455 w510 w600 w943 w995 w1329 w1445 w1538 w1858 w2003 w2191 w2375 w2579 w2828 w3047 w3240 w3309 w3376 w3449 w3506 w3575 w3643 w3707 w3807 w3968 w4159 w4379 w4578 w4686]
      tunnel: [w190 w373 w455 w510 w600 w943 w995 w1329 w1445 w1538 w1858 w2002 w2191 w2375 w2579 w2828 w3047 w3240 w3309 w3376 w3449 w3506 w3575 w3643 w3707 w3807 w3968 w4159 w4379 w4578 w4686] -> w108
      tunnel: w106 -> [_ _ _ _ _ _ _ w1325 w1443 w1537 _ _ _ _ _ _ _ _ _ _ _ _ _ _ _ _ _ _ _ _ _]
      tunnel: [_ _ _ _ _ _ _ w1287 w1440 w1536 _ _ _ _ _ _ _ _ _ _ _ _ _ _ _ _ _ _ _ _ _] -> w105
      tunnel: w104 -> [w189 w371 w454 w509 w598 _ w994 w1313 w1430 w1535 w1857 w2000 w2190 w2374 w2575 w2824 w3046 w3239 w3308 w3375 w3448 w3505 w3574 w3642 w3706 w3806 w3967 w4158 w4378 w4577 w4685]
      tunnel: [w189 w371 w454 w509 w596 0 w994 w1313 w1430 w1535 w1857 w2000 w2190 w2374 w2575 w2824 w3046 w3239 w3308 w3375 w3448 w3505 w3574 w3642 w3706 w3806 w3967 w4158 w4378 w4577 w4685] -> w103
      tunnel: w102 -> [w188 w370 w453 w508 w594 w936 w993 w1312 w1429 w1534 w1856 w1999 w2189 w2373 w2574 w2823 w3045 w3238 w3307 w3374 w3447 w3504 w3573 w3641 w3705 w3805 w3966 w4157 w4377 w4576 w4684]
      tunnel: [w188 w370 w453 w508 w594 w935 w993 w1312 w1429 w1534 w1856 w1999 w2189 w2373 w2574 w2823 w3045 w3238 w3307 w3374 w3447 w3504 w3573 w3641 w3705 w3805 w3966 w4157 w4377 w4576 w4684] -> w101
      tunnel: w100 -> [w186 w368 w452 w506 w588 w932 w991 w1300 w1417 w1528 w1855 w1994 w2187 w2368 w2565 w2813 w3042 w3235 w3304 w3371 w3445 w3501 w3570 w3638 w3704 w3803 w3964 w4156 w4375 w4574 w4682]
      tunnel: [w186 w368 w452 w506 w588 w932 w991 w1300 w1417 w1528 w1855 w1994 w2182 w2368 w2565 w2813 w3042 w3235 w3304 w3371 w3445 w3501 w3570 w3638 w3704 w3803 w3964 w4156 w4375 w4574 w4682] -> w99
      tunnel: w97 -> [w185 w366 w438 w505 w587 w931 w990 w1297 w1413 w1527 w1813 w1984 w2179 w2363 w2561 w2809 w3037 w3234 w3303 w3370 w3444 w3500 w3569 w3637 w3703 w3802 w3961 w4148 w4374 w4572 w4673]
      tunnel: [w185 w366 w438 w505 w587 w931 w990 w1297 w1413 w1527 w1813 w1984 w2179 w2363 w2561 w2809 w3037 w3234 w3303 w3370 w3443 w3500 w3569 w3637 w3703 w3802 w3961 w4148 w4374 w4572 w4673] -> w96
      tunnel: w94 -> [w184 w365 w437 w504 w586 w930 w989 w1296 w1412 w1526 w1812 w1983 w2178 w2360 w2560 w2808 w3036 w3233 w3302 w3369 w3442 w3499 w3568 w3636 w3702 w3801 w3960 w4147 w4373 w4571 w4672]
      tunnel: [w184 w365 w437 w504 w585 w930 w989 w1296 w1412 w1526 w1812 w1983 w2178 w2360 w2560 w2808 w3036 w3233 w3302 w3369 w3442 w3499 w3568 w3636 w3702 w3801 w3960 w4147 w4373 w4571 w4672] -> w95
      tunnel: w93 -> [_ _ _ _ _ _ _ _ _ _ _ _ _ _ _ _ _ _ _ _ _ _ _ _ _ _ _ _ _ _ w4671]
      tunnel: w92 -> [w183 w364 w436 w503 w580 w929 w988 w1295 w1411 w1521 w1811 w1976 w2177 w2357 w2559 w2807 w3034 w3232 w3301 w3368 w3436 w3498 w3567 w3635 w3700 w3800 w3959 w4146 w4372 w4570 w4663]
      tunnel: [w183 w364 w436 w503 w580 w929 w988 w1295 w1411 w1521 w1811 w1976 w2177 w2357 w2559 w2807 w3034 w3232 w3301 w3368 w3436 w3498 w3567 w3635 w3700 w3800 w3959 w4146 w4372 w4570 w4663] -> w91
      tunnel: [w182 w363 w435 w502 w579 w928 w987 w1294 w1410 w1520 w1810 w1975 w2176 w2356 w2558 w2806 w3033 w3231 w3300 w3367 w3435 w3497 w3566 w3634 w3699 w3799 w3958 w4145 w4371 w4569 w4670] -> w90
      tunnel: w89 -> [w182 w363 w435 w502 w579 w928 w987 w1294 w1410 w1520 w1810 w1975 w2176 w2356 w2558 w2806 w3033 w3231 w3300 w3367 w3435 w3497 w3566 w3634 w3699 w3799 _ w4145 _ w4569 w4670]
      tunnel: w88 -> [_ w359 _ _ _ _ _ _ _ _ _ _ _ _ _ _ _ w3230 w3299 w3362 w3434 w3492 w3561 w3629 _ _ _ _ _ _ _]
      tunnel: [w181 w362 w434 w498 w578 w927 w986 w1293 w1409 w1519 w1809 w1961 w2175 w2355 w2557 w2804 w3030 w3229 w3298 w3366 w3433 w3496 w3565 w3633 w3694 w3798 w3957 w4143 w4367 w4568 w4669] -> w85
      tunnel: w86 -> [w181 w362 w434 w498 w578 w927 w986 w1293 w1409 w1519 w1809 w1960 w2175 w2355 w2557 w2804 w3030 w3229 w3298 w3366 w3433 w3496 w3565 w3633 w3694 w3798 w3957 w4143 w4367 w4568 w4669]
      tunnel: w84 -> [w180 w361 w433 w501 w577 w926 w985 w1292 w1408 w1518 w1808 w1959 w2174 w2354 w2551 w2799 w3029 w3228 w3297 w3365 w3432 w3495 w3564 w3632 w3693 w3797 w3956 w4142 w4366 w4567 w4668]
      tunnel: [w180 w361 w433 w501 w577 w926 w985 w1292 w1408 w1518 w1808 w1959 w2174 w2354 w2555 w2803 w3029 w3228 w3297 w3365 w3432 w3495 w3564 w3632 w3693 w3797 w3956 w4142 w4366 w4567 w4668] -> w83
      tunnel: w82 -> [w178 w360 w431 w500 w575 w924 w983 w1290 w1406 w1516 w1806 w1957 w2171 w2352 w2546 _ w3028 w3226 w3295 w3363 w3430 w3493 w3562 w3630 w3691 w3796 w3955 w4140 w4365 w4566 w4667]
      tunnel: [w178 w360 w431 w499 w575 w924 w983 w1290 w1406 w1516 w1806 w1957 w2172 w2352 w2545 _ w3028 w3226 w3295 w3363 w3430 w3493 w3562 w3630 w3691 w3796 w3955 w4140 w4365 w4566 w4667] -> w81
      tunnel: w80 -> [w177 w357 _ _ _ _ _ _ _ _ _ w1948 _ _ w2538 w2793 _ _ _ _ _ _ _ _ _ _ _ _ _ w4564 _]
      tunnel: [w176 w355 w430 w496 w574 w923 w982 w1289 w1405 w1515 w1805 w1936 w2166 w2348 w2547 w2796 w3027 w3224 w3293 w3360 w3428 w3490 w3559 w3627 w3690 w3795 w3954 w4139 w4364 w4565 w4666] -> w79
      tunnel: w78 -> [w176 w355 w430 w496 w574 w923 w982 w1289 w1405 w1515 w1805 _ w2166 w2348 w2547 w2796 w3027 w3224 w3293 w3360 w3428 w3490 w3559 w3627 w3690 w3795 w3954 w4139 w4364 w4565 w4666]
      tunnel: [w175 w354 w429 w495 w573 w922 w981 w1288 w1404 w1514 w1804 w1949 w2165 w2347 w2539 w2794 w3026 w3223 w3292 w3359 w3427 w3489 w3558 w3626 w3689 w3794 w3953 w4138 w4363 w4562 w4665] -> w77
      tunnel: w76 -> [w175 w354 w429 w495 w573 w922 w981 w1288 w1404 w1514 w1804 w1949 _ w2347 w2539 w2794 w3026 w3223 w3292 w3359 w3427 w3489 w3558 w3626 w3689 w3794 w3953 w4138 w4363 w4562 w4665]
      frame "Initialize" {
        w233 = 1 items=["Snap", "Sequence"] ("Capture mode")
        w240 = u32 4343216 items=["SENSOR MODE"=4212128, "SENSOR MODE LINE BUNDLE HEIGHT"=4212192, "READOUT DIRECTION"=4211904, "BIT PER CHANNEL"=4342976, "EXPOSURE TIME"=2049184, "CONTRAST GAIN"=3163312, "BINNING"=4215968, "TIMING READOUT TIME"=4223904, "INTERNAL FRAME RATE"=4225952, "INTERNAL FRAME INTERVAL"=4225968, "INTERNAL LINE SPEED"=4226000, "IMAGE WIDTH"=4343200, "IMAGE HEIGHT"=4343216, "IMAGE ROWBYTES"=4343232, "IMAGE FRAMEBYTES"=4343248, "IMAGE PIXEL TYPE"=4343296] ("Parameter")
        w241 = u32 4343200 items=["SENSOR MODE"=4212128, "SENSOR MODE LINE BUNDLE HEIGHT"=4212192, "READOUT DIRECTION"=4211904, "BIT PER CHANNEL"=4342976, "EXPOSURE TIME"=2049184, "CONTRAST GAIN"=3163312, "BINNING"=4215968, "TIMING READOUT TIME"=4223904, "INTERNAL FRAME RATE"=4225952, "INTERNAL FRAME INTERVAL"=4225968, "INTERNAL LINE SPEED"=4226000, "IMAGE WIDTH"=4343200, "IMAGE HEIGHT"=4343216, "IMAGE ROWBYTES"=4343232, "IMAGE FRAMEBYTES"=4343248, "IMAGE PIXEL TYPE"=4343296] ("Parameter")
        (unwired) u16 0 items=["なし", "XON/XOFF", "RTS/CTS", "XON/XOFF & RTS/CTS", "DTR/DSR", "XON/XOFF & DTR/DSR"] ("flow control (0:none)")
        w254 = u32 2 items=["FORWARD"=1, "BACKWARD"=2] ("Readout Direction")
        w281 = u32 2049184 items=["SENSOR MODE"=4212128, "SENSOR MODE LINE BUNDLE HEIGHT"=4212192, "READOUT DIRECTION"=4211904, "BIT PER CHANNEL"=4342976, "EXPOSURE TIME"=2049184, "CONTRAST GAIN"=3163312, "BINNING"=4215968, "TIMING READOUT TIME"=4223904, "INTERNAL FRAME RATE"=4225952, "INTERNAL FRAME INTERVAL"=4225968, "INTERNAL LINE SPEED"=4226000, "IMAGE WIDTH"=4343200, "IMAGE HEIGHT"=4343216, "IMAGE ROWBYTES"=4343232, "IMAGE FRAMEBYTES"=4343248, "IMAGE PIXEL TYPE"=4343296] ("Parameter")
        w275 = 2 items=["Internal"=1, "External"=2, "Software"=3, "Master Pulse"=4] ("Source")
        w262 = u32 2 items=["NEGATIVE"=1, "POSITIVE"=2] ("Output Trigger Polarity")
        w270 = u32 3 items=["LOW"=1, "GLOBAL EXPOSURE"=2, "PROGRAMMABLE"=3, "TRIGGER READY"=4, "HIGH"=5] ("Output Trigger Mode")
        w267 = u32 4 items=["Exposure"=1, "Readout End"=2, "V Sync"=3, "H Sync"=4, "Trigger"=6] ("Source")
        w261 = u32 4226016 items=["SENSOR MODE"=4212128, "CCD MODE"=4212384, "READOUT MODE"=4211872, "ACTIVE VIEW INDEX"=4343136, "BITS PER CHANNEL"=4342976, "IMAGE PIXEL TYPE"=4343296, "BINNING"=4215968, "EXPOSURE TIME"=2049184, "CONTRAST GAIN"=3163312, "CONTRAST OFFSET"=3163328, "LIGHT MODE"=2114720, "SENSITIVITY"=2114992, "PHOTON IMAGING MODE"=2115200, "HIGH DYNAMIC RANGE MODE"=3163360, "WHITE BALANCE"=3163568, "TEMPERATURE"=2115232, "TEMPERATURE TARGET"=2115264, "SENSOR COOLER FAN"=2115296, "LINEBUNDLE HEIGHT"=4212192, "MECHANICAL SHUTTER"=2115488, "BACK FOCUS POSITION"=8422304, "TRIGGER CONNECTOR"=1066432, "TRIGGER SOURCE"=1066144, "OUTPUT TRIGGER SOURCE"=1852576, "TRIGGER GLOBAL EXPOSURE"=2049680, "FIRST TRIGGER BEHAVIOR"=2049696, "CHANNEL SYNC"=1852352, "READOUT DIRECTION"=4211904, "PRE HSYNC COUNT"=1852704, "INTERNAL LINE SPEED"=4226000, "INTERNAL LINE INTERVAL"=4226016] ("Parameter")
        w258 = u32 4212128 items=["SENSOR MODE"=4212128, "CCD MODE"=4212384, "READOUT MODE"=4211872, "ACTIVE VIEW INDEX"=4343136, "BITS PER CHANNEL"=4342976, "IMAGE PIXEL TYPE"=4343296, "BINNING"=4215968, "EXPOSURE TIME"=2049184, "CONTRAST GAIN"=3163312, "CONTRAST OFFSET"=3163328, "LIGHT MODE"=2114720, "SENSITIVITY"=2114992, "PHOTON IMAGING MODE"=2115200, "HIGH DYNAMIC RANGE MODE"=3163360, "WHITE BALANCE"=3163568, "TEMPERATURE"=2115232, "TEMPERATURE TARGET"=2115264, "SENSOR COOLER FAN"=2115296, "LINEBUNDLE HEIGHT"=4212192, "MECHANICAL SHUTTER"=2115488, "BACK FOCUS POSITION"=8422304, "TRIGGER CONNECTOR"=1066432, "TRIGGER SOURCE"=1066144, "OUTPUT TRIGGER SOURCE"=1852576, "TRIGGER GLOBAL EXPOSURE"=2049680, "FIRST TRIGGER BEHAVIOR"=2049696, "CHANNEL SYNC"=1852352, "READOUT DIRECTION"=4211904, "PRE HSYNC COUNT"=1852704, "INTERNAL LINE SPEED"=4191408, "INTERNAL LINE INTERVAL"=4191424] ("Parameter")
        w257 = u32 1852704 items=["SENSOR MODE"=4212128, "CCD MODE"=4212384, "READOUT MODE"=4211872, "ACTIVE VIEW INDEX"=4343136, "BITS PER CHANNEL"=4342976, "IMAGE PIXEL TYPE"=4343296, "BINNING"=4215968, "EXPOSURE TIME"=2049184, "CONTRAST GAIN"=3163312, "CONTRAST OFFSET"=3163328, "LIGHT MODE"=2114720, "SENSITIVITY"=2114992, "PHOTON IMAGING MODE"=2115200, "HIGH DYNAMIC RANGE MODE"=3163360, "WHITE BALANCE"=3163568, "TEMPERATURE"=2115232, "TEMPERATURE TARGET"=2115264, "SENSOR COOLER FAN"=2115296, "LINEBUNDLE HEIGHT"=4212192, "MECHANICAL SHUTTER"=2115488, "BACK FOCUS POSITION"=8422304, "TRIGGER CONNECTOR"=1066432, "TRIGGER SOURCE"=1066144, "OUTPUT TRIGGER SOURCE"=1852576, "TRIGGER GLOBAL EXPOSURE"=2049680, "FIRST TRIGGER BEHAVIOR"=2049696, "CHANNEL SYNC"=1852352, "READOUT DIRECTION"=4211904, "PRE HSYNC COUNT"=1852704, "INTERNAL LINE SPEED"=4191408, "INTERNAL LINE INTERVAL"=4191424] ("Parameter")
        w256 = u32 4211904 items=["SENSOR MODE"=4212128, "CCD MODE"=4212384, "READOUT MODE"=4211872, "ACTIVE VIEW INDEX"=4343136, "BITS PER CHANNEL"=4342976, "IMAGE PIXEL TYPE"=4343296, "BINNING"=4215968, "EXPOSURE TIME"=2049184, "CONTRAST GAIN"=3163312, "CONTRAST OFFSET"=3163328, "LIGHT MODE"=2114720, "SENSITIVITY"=2114992, "PHOTON IMAGING MODE"=2115200, "HIGH DYNAMIC RANGE MODE"=3163360, "WHITE BALANCE"=3163568, "TEMPERATURE"=2115232, "TEMPERATURE TARGET"=2115264, "SENSOR COOLER FAN"=2115296, "LINEBUNDLE HEIGHT"=4212192, "MECHANICAL SHUTTER"=2115488, "BACK FOCUS POSITION"=8422304, "TRIGGER CONNECTOR"=1066432, "TRIGGER SOURCE"=1066144, "OUTPUT TRIGGER SOURCE"=1852576, "TRIGGER GLOBAL EXPOSURE"=2049680, "FIRST TRIGGER BEHAVIOR"=2049696, "CHANNEL SYNC"=1852352, "READOUT DIRECTION"=4211904, "PRE HSYNC COUNT"=1852704, "INTERNAL LINE SPEED"=4191408, "INTERNAL LINE INTERVAL"=4191424] ("Parameter")
        # "settings for camera"
        # "settings for filters"
        n30 = call-poly <vilib>:"DAQmx Write.vi"("task/channels in"=w177, "data"=FALSE) -> ()  [unwired: 11 in, 3 out]
        n31 = call <userlib>:"tm_initialize_40.vi"() -> ("error out"=w247:errorcluster)  [unwired: 8 in, 3 out]
        n32 = Wait (ms)(milliseconds to wait=u32 500) -> ()  [unwired: 1 out]
        n33 = call <userlib>:"tm_opencamera_40.vi"("error in (no error)"=w247, "Camera Index"=u32 0) -> ("error out"=w271:errorcluster, "Handle out"=w272:u32)  [unwired: 7 in, 1 out]
        n34 = property class="BenchtopStepperControl"(reference="BenchtopStepperControl", "SerialNumber"="SerialNumber") -> (reference out=w203:refnum<k24>, error out=w202:errorcluster)  [unwired: 1 in]
        n35 = call <userlib>:"tm_setparameter_40.vi"("error in (no error)"=w271, "Value in"=12.0, "Parameter"=w258, "Handle in"=w272) -> ("error out"=w269:errorcluster, "Handle out"=w268:u32)  [unwired: 6 in]
        n36 = To Double Precision Float(number=u32 0) -> (double precision float=w250:dbl)
        n37 = call <userlib>:"tm_setparameter_40.vi"("error in (no error)"=w269, "Value in"=w250, "Parameter"=w257, "Handle in"=w268) -> ("error out"=w251:errorcluster, "Handle out"=w252:u32)  [unwired: 6 in]
        n38 = To Double Precision Float(number=w254) -> (double precision float=w253:dbl)
        n39 = invoke class="BenchtopStepperControl" method="CreateDevice"(reference=w203, error in=w202) -> (reference out=w199:refnum<k24>, error out=w198:errorcluster)  [unwired: 1 in, 1 out]
        n40 = call <userlib>:"tm_setparameter_40.vi"("error in (no error)"=w251, "Value in"=w253, "Parameter"=w256, "Handle in"=w252) -> ("error out"=w260:errorcluster, "Handle out"=w259:u32)  [unwired: 6 in]
        n41 = call <userlib>:"tm_setparameter_40.vi"("error in (no error)"=w260, "Value in"=9.74436e-06, "Parameter"=w261, "Handle in"=w259) -> ("error out"=w280:errorcluster, "Handle out"=w279:u32)  [unwired: 6 in]
        n42 = Bundle("Output Trigger Mode"=w270, "Output Trigger Polarity"=w262) -> (w263:T9)  [unwired: 1 in]
        n43 = call <userlib>:"tm_setparameter_40.vi"("error in (no error)"=w280, "Value in"="Exposure time", "Parameter"=w281, "Handle in"=w279) -> ("error out"=w278:errorcluster, "Handle out"=w277:u32)  [unwired: 6 in]
        n44 = Bundle("Output Trigger Period"=1e-06, "Delay"=0.0, "Source"=w267) -> (w264:T10)  [unwired: 1 in]
        n45 = property class="BenchtopStepperControl"(reference=w199, error in=w198) -> (reference out=w197:refnum<k24>, "BenchtopStepperMotor"=w193:refnum<k24>)  [unwired: 1 out]
        n46 = invoke class="StepperMotorChannel" method="SetMoveAbsolutePosition"(reference=w193, "position"="position") -> (reference out=w194:refnum<k24>)  [unwired: 2 in, 3 out]
        n47 = invoke class="StepperMotorChannel" method="MoveAbsolute"(reference=w194, "waitTimeout"=1000) -> (reference out=w192:refnum<k24>)  [unwired: 2 in, 3 out]
        n48 = call <userlib>:"tm_inputtriggersource_40.vi"("error in (no error)"=w278, "External Options"=cluster{"Polarity":i32, "Delay":dbl} {"Polarity"=2, "Delay"=0.0}, "Source"=w275, "Handle in"=w277) -> ("error out"=w274:errorcluster, "Handle out"=w273:u32)  [unwired: 6 in]
        n49 = call <userlib>:"tm_setoutputtrigger_40.vi"("Port"=0 ("Index"), "error in (no error)"=w274, "Programmable Options"=w264, "Type"=w263, "Handle in"=w273) -> ("error out"=w237:errorcluster, "Handle out"=w231:u32)  [unwired: 5 in]
        n50 = call <userlib>:"tm_getparameter_40.vi"("error in (no error)"=w237, "Parameter"=w240, "Handle in"=w231) -> ("error out"=w239:errorcluster, "Value out"=w242:dbl, "Handle out"=w230:u32)  [unwired: 6 in]
        n51 = call <userlib>:"tm_getparameter_40.vi"("error in (no error)"=w239, "Parameter"=w241, "Handle in"=w230) -> ("error out"=w238:errorcluster, "Value out"=w243:dbl)  [unwired: 6 in, 1 out]
        n52 = stacked-sequence "sg triggers" {
          seq-local: [w286 _ _ _ _ _ _ _ _ _] -> [_ w293 _ _ _ _ _ _ _ _]
          seq-local: [w284 _ _ _ _ _ _ _ _ _] -> [_ w290 _ _ _ _ _ _ _ _]
          seq-local: [_ w293 _ _ _ _ _ _ _ _] -> [_ _ w298 _ _ _ _ _ _ _]
          seq-local: [_ w289 _ _ _ _ _ _ _ _] -> [_ _ w296 _ _ _ _ _ _ _]
          seq-local: [_ _ w298 _ _ _ _ _ _ _] -> [_ _ _ w303 _ _ _ _ _ _]
          seq-local: [_ _ w294 _ _ _ _ _ _ _] -> [_ _ _ w299 _ _ _ _ _ _]
          seq-local: [_ _ _ w300 _ _ _ _ _ _] -> [_ _ _ _ w308 _ _ _ _ _]
          seq-local: [_ _ _ w299 _ _ _ _ _ _] -> [_ _ _ _ w304 _ _ _ _ _]
          seq-local: [_ _ _ _ w305 _ _ _ _ _] -> [_ _ _ _ _ w313 _ _ _ _]
          seq-local: [_ _ _ _ w304 _ _ _ _ _] -> [_ _ _ _ _ w309 _ _ _ _]
          seq-local: [_ _ _ _ _ w310 _ _ _ _] -> [_ _ _ _ _ _ w317 _ _ _]
          seq-local: [_ _ _ _ _ w309 _ _ _ _] -> [_ _ _ _ _ _ w318 _ _ _]
          seq-local: [_ _ _ _ _ _ w316 _ _ _] -> [_ _ _ _ _ _ _ w320 _ _]
          seq-local: [_ _ _ _ _ _ w318 _ _ _] -> [_ _ _ _ _ _ _ w323 _ _]
          seq-local: [_ _ _ _ _ _ _ w319 _ _] -> [_ _ _ _ _ _ _ _ w325 _]
          seq-local: [_ _ _ _ _ _ _ w323 _ _] -> [_ _ _ _ _ _ _ _ w327 _]
          seq-local: [_ _ _ _ _ _ _ _ w325 _] -> [_ _ _ _ _ _ _ _ _ w330]
          seq-local: [_ _ _ _ _ _ _ _ w327 _] -> [_ _ _ _ _ _ _ _ _ w328]
          tunnel: refnum<visa-resource-name> "USB0::0x1AB1::0x0643::DG9A242400208::INSTR" ("sg triggers") -> [w288 _ _ _ _ _ _ _ _ _]
          tunnel: refnum<visa-resource-name> "USB0::0x1AB1::0x0643::DG9A242400205::INSTR" ("sg triggers") -> [w285 _ _ _ _ _ _ _ _ _]
          frame #0 {
            n53 = VISA Open(VISA resource name=w288) -> (VISA resource name=w286:refnum<visa-resource-name>)  [unwired: 4 in, 1 out]
            n54 = VISA Open(VISA resource name=w285) -> (VISA resource name=w284:refnum<visa-resource-name>)  [unwired: 4 in, 1 out]
            n55 = Wait (ms)(milliseconds to wait=u32 500) -> ()  [unwired: 1 out]
          }
          frame #1 {
            n56 = VISA Write(VISA resource name=w290, write buffer=":OUTP2 ON") -> (VISA resource name out=w289:refnum<visa-resource-name>)  [unwired: 1 in, 2 out]
            n57 = Wait (ms)(milliseconds to wait=u32 500) -> ()  [unwired: 1 out]
          }
          frame #2 {
            n58 = VISA Write(VISA resource name=w296, write buffer=":OUTP1 ON") -> (VISA resource name out=w294:refnum<visa-resource-name>)  [unwired: 1 in, 2 out]
            n59 = Wait (ms)(milliseconds to wait=u32 500) -> ()  [unwired: 1 out]
          }
          frame #3 {
            n60 = VISA Write(VISA resource name=w303, write buffer=":OUTP2 ON") -> (VISA resource name out=w300:refnum<visa-resource-name>)  [unwired: 1 in, 2 out]
            n61 = Wait (ms)(milliseconds to wait=u32 500) -> ()  [unwired: 1 out]
          }
          frame #4 {
            n62 = VISA Write(VISA resource name=w308, write buffer=":OUTP1 ON") -> (VISA resource name out=w305:refnum<visa-resource-name>)  [unwired: 1 in, 2 out]
            n63 = Wait (ms)(milliseconds to wait=u32 500) -> ()  [unwired: 1 out]
          }
          frame #5 {
            n64 = VISA Write(VISA resource name=w313, write buffer=":TRIG1") -> (VISA resource name out=w310:refnum<visa-resource-name>)  [unwired: 1 in, 2 out]
            n65 = Wait (ms)(milliseconds to wait=u32 500) -> ()  [unwired: 1 out]
          }
          frame #6 {
            n66 = VISA Write(VISA resource name=w317, write buffer=":TRIG1") -> (VISA resource name out=w316:refnum<visa-resource-name>)  [unwired: 1 in, 2 out]
            n67 = Wait (ms)(milliseconds to wait=u32 500) -> ()  [unwired: 1 out]
          }
          frame #7 {
            n68 = VISA Write(VISA resource name=w320, write buffer=":TRIG2") -> (VISA resource name out=w319:refnum<visa-resource-name>)  [unwired: 1 in, 2 out]
            n69 = Wait (ms)(milliseconds to wait=u32 500) -> ()  [unwired: 1 out]
          }
          frame #8 {
            n70 = VISA Write(VISA resource name=w325, write buffer=":TRIG2") -> ()  [unwired: 1 in, 3 out]
            n71 = Wait (ms)(milliseconds to wait=u32 500) -> ()  [unwired: 1 out]
          }
          frame #9 {
            n72 = VISA Clear(VISA resource name=w330) -> ()  [unwired: 1 in, 2 out]
            n73 = VISA Clear(VISA resource name=w328) -> ()  [unwired: 1 in, 2 out]
            n74 = Wait (ms)(milliseconds to wait=u32 200) -> ()  [unwired: 1 out]
          }
        }
        n75 = for {
          N: "Frames in memory 2" -> [_]
          tunnel: [w338] -> w234 mode=indexing
          tunnel: [w337] -> w236
          tunnel: w238 -> [w335]
          tunnel: w243 -> [w334]
          tunnel: w242 -> [w333]
          tunnel: [w332] -> w229 mode=indexing
          i -> [w342]
          w339 = T11 7 items=["Grayscale (U8)", "Grayscale (I16)", "Grayscale (SGL)", "Complex (CSG)", "RGB (U32)", "HSL (U32)", "RGB (U64)", "Grayscale (U16)"] ("Image Type")
          w344 = 0
          n76 = Number To Decimal String(number=w342, width (-)=i16 3) -> (decimal integer string=w343:string)
          n77 = call "IMAQ Create"("Border Size"=0, "Image Name"=w343, "Image Type"=w339, "error in (no error)"=w335) -> ("New Image"=w331:T12, "error out"=w346:errorcluster)  [unwired: 1 in]
          n78 = call "IMAQ SetImageSize"("error in (no error)"=w346, "Y Resolution"=w333, "X Resolution"=w334, "Image"=w331) -> ("error out"=w345:errorcluster, "Image Out"=w332:T12)  [unwired: 1 in]
          n79 = call "IMAQ GetImagePixelPtr"("Function"=T5."Map Pixel Pointer", "error in (no error)"=w345, "Y Coordinate"=w344, "X Coordinate"=w344, "Image"=w332) -> ("error out"=w337:errorcluster, "Pixel Pointer out"=w338:u64)  [unwired: 1 in, 4 out]
        }
        n80 = call "RS232C_Init.vi"("baud rate"=u16 9600 ("baud rate 2"), "COM Port"=refnum<visa-resource-name> "COM4" ("VISA resource name")) -> ("VISA resource name out"=w206:refnum<visa-resource-name>)  [unwired: 1 in, 2 out]
        n81 = call <userlib>:"tm_prepare_attach_40.vi"("error in (no error)"=w236, "buffers"=w234, "Capture mode"=w233) -> ("error out"=w235:errorcluster, "Handle out"=w232:u32)  [unwired: 7 in]
      }
      frame "Chilling", Default {
        w384 = u8 2 items=["0", "1", "2", "3", "4"] ("Axis Number")
        n82 = call-poly <vilib>:"DAQmx Write.vi"("task/channels in"=w347, "data"="405") -> ()  [unwired: 11 in, 3 out]
        n83 = call-poly <vilib>:"DAQmx Write.vi"("task/channels in"=w357, "data"="galvano") -> ()  [unwired: 11 in, 3 out]
        n84 = call-poly <vilib>:"DAQmx Write.vi"("task/channels in"=w349, "data"="488", "error in"=w407) -> ()  [unwired: 10 in, 3 out]
        n85 = event shown="[5] \"manual edgehunting\": Value Change" {
          selector: _ -> [_ _ _ _ _ _ _ _ _ _ _ _]
          dyn-events: _ -> [_ _ _ _ _ _ _ _ _ _ _ _]
          timeout: _ -> [_ _ _ _ _ _ _ _ _ _ _ _]
          tunnel: [states."Stream w/o flow" states."Close" states."405_r" states."tube position" states."robotic arm" states."Edgehunting" states."wait for clearing" states."save" states."reverse" states."antic\n" states."405" states."manual loading"] -> w367
          event "START": Value Change {
            n86 = event-data() -> ()  [unwired: 1 in, 6 out]
            n87 = local write "READY"(FALSE ("Ready")) -> ()
            n88 = local write "Streaming"(TRUE ("Streaming")) -> ()
          }
          event "Shut down": Value Change {
            n89 = event-data() -> ()  [unwired: 1 in, 6 out]
            n90 = local write "READY"(FALSE ("Ready")) -> ()
          }
          event "START AUTO IMAGING": Value Change {
            n91 = event-data() -> ()  [unwired: 1 in, 6 out]
          }
          event "Force move": Value Change {
            n92 = event-data() -> ()  [unwired: 1 in, 6 out]
          }
          event "manual load": Value Change {
            n93 = event-data() -> ()  [unwired: 1 in, 6 out]
          }
          event "manual edgehunting": Value Change {
            n94 = event-data() -> ()  [unwired: 1 in, 6 out]
          }
          event "wait for\nclearing": Value Change {
            n95 = event-data() -> ()  [unwired: 1 in, 6 out]
          }
          event "manual imaging": Value Change {
            n96 = event-data() -> ()  [unwired: 1 in, 6 out]
          }
          event "reverse": Value Change {
            n97 = event-data() -> ()  [unwired: 1 in, 6 out]
          }
          event "force anticlogging": Value Change {
            n98 = event-data() -> ()  [unwired: 1 in, 6 out]
          }
          event "manual 4c": Value Change {
            n99 = event-data() -> ()  [unwired: 1 in, 6 out]
          }
          event "manual loading": Value Change {
            n100 = event-data() -> ()  [unwired: 1 in, 6 out]
          }
        }
        n101 = call-poly <vilib>:"DAQmx Write.vi"("task/channels in"=w406, "data"="532") -> ()  [unwired: 11 in, 3 out]
        n102 = call-poly <vilib>:"DAQmx Write.vi"("task/channels in"=w405, "data"="594") -> ()  [unwired: 11 in, 3 out]
        n103 = call-poly <vilib>:"DAQmx Write.vi"("task/channels in"=w359, "data"="647") -> ()  [unwired: 11 in, 3 out]
        n104 = call "RS232C_SetSpeed.vi"("Low Speed"=u32 100, "High Speed"="scanning Speed", "Acceleration Time"=u16 100, "Axis Number"=w384, "Delimiter"="\r\n", "VISAリソース名"=w388, "Axis Count"=u8 2, "Range"=TRUE, "Main/Sub"=TRUE) -> ()  [unwired: 2 out]
        "Streaming" <- FALSE ("Streaming")
        "READY" <- TRUE ("Ready")
        "Moving" <- FALSE ("Moving")
        "Saving image" <- FALSE ("Saving image")
        "532  2" <- "532"
        "594  2" <- "594"
        "488 2" <- "488"
        "405 2" <- "405"
        "647 2" <- "647"
      }
      frame "wait for clearing" {
        # "wait for the signal from robot arm"
        n105 = call-poly <vilib>:"DAQmx Create Virtual Channel.vi"("lines"=tag "Dev1/port2/line6") -> ("task out"=w450:refnum<k21>, "error out"=w448:errorcluster)  [unwired: 13 in]
        n106 = call <vilib>:"DAQmx Start Task.vi"("task/channels in"=w450, "error in"=w448) -> ("task out"=w447:refnum<k21>, "error out"=w443:errorcluster)  [unwired: 12 in]
        n107 = while {
          tunnel: w447 -> [w492]
          tunnel: [w491] -> w444
          tunnel: w443 -> [w490]
          tunnel: [w489] -> w442
          shift-right: [w485] -> w440
          shift-left: FALSE -> [_]
          stop <- w488 stop-if-true
          n108 = call-poly <vilib>:"DAQmx Read.vi"("task/channels in"=w492, "error in"=w490) -> ("task out"=w491:refnum<k21>, "data"=w485:bool, "error out"=w489:errorcluster)  [unwired: 11 in]
          "clear finished?" <- w485
          n109 = Or(x=w485, y="wait for clearing? 2") -> (x .or. y?=w488:bool)
          n110 = call <vilib>:"High Resolution Relative Seconds.vi"() -> ("relative seconds"=→"relative seconds 2":dbl)
        }
        n111 = call <vilib>:"DAQmx Stop Task.vi"("task/channels in"=w444, "error in"=w442) -> ("task out"=w446:refnum<k21>, "error out"=w445:errorcluster)  [unwired: 12 in]
        n112 = flat-sequence {
          tunnel: w440 -> [w484]
          tunnel: [w484] -> w439
          frame #0 {
            n113 = Wait (ms)(milliseconds to wait=u32 50) -> ()  [unwired: 1 out]
          }
        }
        n114 = call <vilib>:"DAQmx Clear Task.vi"("task in"=w446, "error in"=w445) -> ()  [unwired: 13 in, 1 out]
        n115 = case shown="False" w439 {
          tunnel: [states."Chilling" states."robotic arm"] -> w451
          frame False {
          }
          frame True {
          }
        }
      }
      frame "Stream w/o flow" {
        # "Imaging for preview"
        n116 = call <userlib>:"tm_startcapture_40.vi"("error in (no error)"=w533, "Handle in"=w497) -> ("error out"=w541:errorcluster, "Handle out"=w542:u32)  [unwired: 8 in]
        n117 = while {
          tunnel: [w554] -> w543
          tunnel: [w555] -> w544
          tunnel: w542 -> [w545]
          tunnel: w541 -> [w571]
          tunnel: w534 -> [w553]
          tunnel: [w553] -> w532
          tunnel: w500 -> [w548]
          tunnel: [w547] -> w499
          stop <- w566 stop-if-true
          # "sub- ROI"
          n118 = call-poly <vilib>:"DAQmx Write.vi"("task/channels in"=w548, "data"="Slide") -> ("task out"=w547:refnum<k21>)  [unwired: 11 in, 2 out]
          n119 = call <userlib>:"tm_waitnextframe_40.vi"("error in (no error)"=w571, "Handle in"=w545) -> ("error out"=w555:errorcluster, "Frame Count"=→"Frame count":i32, "Frame Index"=w557:i32, "Handle out"=w554:u32)  [unwired: 6 in]
          n120 = Index Array(array=w553, index=w557) -> (element=w556:T12)
          n121 = call "IMAQ ImageToArray"("Image"=w556) -> ("Image Pixels (U16)"=w551:u16[][])  [unwired: 3 in, 4 out]
          "Obtained image" <- w551
          n122 = Unbundle By Name(w555) -> ("status"=w568:bool)
          n123 = Array Subset(array=w551, index (row)="XS y px start", length (row)="XS y length", index (col)="XS x px start", length (col)="XS x length") -> (w563:u16[][])
          "Sub image" <- w563
          n124 = Multiply(x="XS y length", y="XS x length") -> (x*y=w560:i32)
          n125 = Build Array("Quit", w568) -> (w567:bool[])
          n126 = Reshape Array(w563, w560) -> (w562:u16[])
          n127 = Or Array Elements(Boolean array=w567) -> (logical OR=w566:bool)
          n128 = call-poly <vilib>:"Mean.vi"("X"=w562) -> ("mean"=→"Sub img mean":dbl)  [unwired: 1 out]
          n129 = Reshape Array(w551, 4194304 ("dimension size")) -> (w552:u16[])
          n130 = call-poly <vilib>:"Mean.vi"("X"=w552) -> ("mean"=→"Mean intensity\nof frame":dbl)  [unwired: 1 out]
        }
        n131 = call <userlib>:"tm_stopcapture_40.vi"("error in (no error)"=w544, "Handle in"=w543) -> ("error out"=w536:errorcluster, "Handle out"=w535:u32)  [unwired: 8 in]
      }
      frame "auto imaging" {
        w572 = 0.0
        n132 = call <vilib>:"High Resolution Relative Seconds.vi"() -> ("relative seconds"=w603:dbl)
        n133 = local read "#of edgehunting"() -> (w601:u32)
        n134 = while {
          shift-right: [w788] -> _
          shift-left: w572 -> [w787]
          tunnel: [w693] -> w624
          shift-right: [w743] -> _
          shift-left: w572 -> [w743]
          tunnel: [w692] -> w613
          tunnel: w612 -> [w691]
          tunnel: [w690] -> w611
          tunnel: "Number of samples" -> [w689]
          tunnel: w604 -> [w688]
          tunnel: w603 -> [w687]
          tunnel: [w685] -> w602
          tunnel: w601 -> [w684]
          tunnel: [w681] -> w597
          shift-right: [w670] -> w585
          shift-left: w586 -> [w671]
          tunnel: [w669] -> w584
          i -> [w666]
          stop <- w745 stop-if-true
          w765 = 10123 items=["Finite Samples"=10178, "Continuous Samples"=10123, "Hardware Timed Single Point"=12522] ("sample mode")
          w767 = 10106 items=["Default"=-1, "RSE"=10083, "NRSE"=10078, "Differential"=10106, "Pseudodifferential"=12529] ("input terminal configuration")
          n135 = Increment(x=w787) -> (x+1=w788:dbl)
          n136 = call-poly <vilib>:"DAQmx Create Virtual Channel.vi"("maximum value"=5.0, "minimum value"=-5.0, "input terminal configuration"=w767, "physical channels"="Physical Channel 2") -> ("task out"=w762:refnum<k21>, "error out"=w761:errorcluster)  [unwired: 10 in]
          n137 = call <vilib>:"High Resolution Relative Seconds.vi"() -> ("relative seconds"=w744:dbl)
          n138 = call-poly <vilib>:"DAQmx Create Virtual Channel.vi"("lines"=tag "Dev1/port0/line5") -> ("task out"=w680:refnum<k21>)  [unwired: 13 in, 1 out]
          n139 = call-poly <vilib>:"DAQmx Create Virtual Channel.vi"("lines"=tag "Dev1/port0/line4") -> ("task out"=w780:refnum<k21>, "error out"=w779:errorcluster)  [unwired: 13 in]
          n140 = call-poly <vilib>:"DAQmx Create Virtual Channel.vi"("lines"=tag "Dev1/port1/line7") -> ("task out"=w785:refnum<k21>, "error out"=w784:errorcluster)  [unwired: 13 in]
          n141 = call-poly <vilib>:"DAQmx Create Virtual Channel.vi"("lines"=tag "Dev1/port0/line7") -> ("task out"=w725:refnum<k21>, "error out"=w730:errorcluster)  [unwired: 13 in]
          n142 = call-poly <vilib>:"DAQmx Create Virtual Channel.vi"("lines"=tag "Dev1/port1/line5") -> ("task out"=w727:refnum<k21>, "error out"=w728:errorcluster)  [unwired: 13 in]
          n143 = call-poly <vilib>:"DAQmx Create Virtual Channel.vi"("lines"=tag "Dev1/port1/line6") -> ("task out"=w726:refnum<k21>, "error out"=w729:errorcluster)  [unwired: 13 in]
          n144 = call-poly <vilib>:"DAQmx Timing.vi"("task/channels in"=w762, "sample mode"=w765, "rate"=10000.0, "source"=tag "OnboardClock", "error in"=w761) -> ("task out"=w760:refnum<k21>, "error out"=w759:errorcluster)  [unwired: 9 in]
          n145 = property class="DAQmx Timing"(reference=w760, error in=w759, "SampClk.Rate"="SampClk.Rate 2") -> (reference out=w757:refnum<k21>, error out=w756:errorcluster)
          n146 = call <vilib>:"DAQmx Start Task.vi"("task/channels in"=w757, "error in"=w756) -> ("task out"=w755:refnum<k21>, "error out"=w754:errorcluster)  [unwired: 12 in]
          n147 = call <vilib>:"DAQmx Start Task.vi"("task/channels in"=w780, "error in"=w779) -> ("task out"=w742:refnum<k21>, "error out"=w740:errorcluster)  [unwired: 12 in]
          n148 = call <vilib>:"DAQmx Start Task.vi"("task/channels in"=w785, "error in"=w784) -> ("task out"=w782:refnum<k21>, "error out"=w781:errorcluster)  [unwired: 12 in]
          n149 = call <vilib>:"DAQmx Start Task.vi"("task/channels in"=w725, "error in"=w730) -> ("task out"=w724:refnum<k21>, "error out"=w723:errorcluster)  [unwired: 12 in]
          n150 = call <vilib>:"DAQmx Start Task.vi"("task/channels in"=w726, "error in"=w729) -> ("task out"=w722:refnum<k21>)  [unwired: 12 in, 1 out]
          n151 = call <vilib>:"DAQmx Start Task.vi"("task/channels in"=w727, "error in"=w728) -> ("task out"=w720:refnum<k21>)  [unwired: 12 in, 1 out]
          n152 = call <vilib>:"DAQmx Start Task.vi"("task/channels in"=w680) -> ("task out"=w678:refnum<k21>)  [unwired: 13 in, 1 out]
          n153 = while {
            tunnel: w755 -> [w921]
            tunnel: w754 -> [w920]
            tunnel: [w919] -> w751
            tunnel: [w918] -> w750
            shift-right: [w917] -> _
            shift-left: w744 -> [w916]
            shift-right: [w913] -> _
            shift-left: 100.0 ("relative seconds") -> [w914]
            tunnel: w791 -> [w912]
            tunnel: w789 -> [w911]
            tunnel: [w893] -> w786
            tunnel: [w912] -> w736
            tunnel: [w911] -> w735
            tunnel: [w896] -> w694
            shift-right: [w908] -> _
            shift-left: w743 -> [w910]
            tunnel: w734 -> [w906]
            tunnel: [w906] -> w732
            tunnel: w733 -> [w905]
            tunnel: [w905] -> w731
            tunnel: w713 -> [w904]
            tunnel: [w904] -> w698
            tunnel: w712 -> [w903]
            tunnel: [w903] -> w697
            tunnel: w710 -> [w902]
            tunnel: [w902] -> w709
            tunnel: w689 -> [w900]
            tunnel: w675 -> [w899]
            tunnel: [w899] -> w674
            tunnel: [w894] -> w668
            stop <- w895 stop-if-true
            n154 = call <vilib>:"High Resolution Relative Seconds.vi"() -> ("relative seconds"=w917:dbl)
            n155 = call-poly <vilib>:"DAQmx Read.vi"("task/channels in"=w921, "number of samples per channel"=w900, "error in"=w920) -> ("task out"=w919:refnum<k21>, "data"=w901:dbl[], "error out"=w918:errorcluster)  [unwired: 10 in]
            "Waveform Graph" <- w901
            n156 = Subtract(x=w917, y=w916) -> (x-y=w909:dbl)
            n157 = Unbundle By Name(w918) -> ()  [unwired: 1 out]
            n158 = Less?(x=w914, y="Trigger") -> (x < y?=w893:bool)
            "Triggered" <- w893
            n159 = Add(x=w910, y=w909) -> (x+y=w908:dbl)
            "Elapsed (sec)" <- w908
            n160 = call-poly <vilib>:"Mean.vi"("X"=w901) -> ("mean"=w913:dbl)  [unwired: 1 out]
            "Mean" <- w913
            "Trigger PD running mean" <- w913
            n161 = Greater?(x=w908, y="reverse flow \nthreshold (sec)") -> (0:w896:bool)
            n162 = Or(x=w893, y="Stop Trigger stream") -> (x .or. y?=w897:bool)
            n163 = Or(x=w897, y=w896) -> (x .or. y?=w895:bool)
            n164 = call <extravilib>:"Write.vi"("element"=w895) -> ("channel"=w894:T13)  [unwired: 1 out]
          }
          n165 = while {
            tunnel: [w802] -> w669
            shift-right: [w808] -> w670
            shift-left: w671 -> [w809]
            shift-right: [w804] -> _
            shift-left: 0 -> [w797]
            tunnel: w668 -> [w799]
            i -> [w800]
            stop <- w801 stop-if-true
            n166 = shared-variable-read(w809) -> (w808:refnum<k21>, w807:cluster{dbl, bool})  [unwired: 2 in, 2 out]
            n167 = Unbundle(w807) -> (→"Numeric 5":dbl, w796:bool)
            "larvae in chamber?" <- w796
            n168 = Not(x=w796) -> (.not. x?=w805:bool)
            n169 = case shown="True" w805 {
              tunnel: w797 -> [w810 w812]
              tunnel: [w810 w811] -> w804
              frame False {
              }
              frame True {
                n170 = Increment(x=w812) -> (x+1=w811:i32)
              }
            }
            n171 = call <extravilib>:"Read.vi"("channel"=w799) -> ("element"=w798:bool)  [unwired: 1 in, 1 out]
            n172 = Greater Or Equal?(x=w804, y=120) -> (x >= y?=w802:bool)
            n173 = Or(x=w798, y=w802) -> (x .or. y?=w801:bool)
            "waiting number" <- w797
            "Numeric 6" <- w800
          }
          "Boolean" <- w669
          n174 = flat-sequence {
            tunnel: [w843] -> w794
            tunnel: w782 -> [w843]
            tunnel: w781 -> [w842]
            tunnel: [w842] -> w793
            tunnel: w742 -> [w829]
            tunnel: [w828] -> w741
            tunnel: w740 -> [w827]
            tunnel: [w826] -> w739
            tunnel: w724 -> [w825]
            tunnel: w723 -> [w823]
            tunnel: w722 -> [w822]
            tunnel: [w822] -> w721
            tunnel: w720 -> [w821]
            tunnel: [w821] -> w719
            tunnel: [w820] -> w714
            tunnel: w678 -> [w819]
            tunnel: [w817] -> w677
            tunnel: w794 -> [w859]
            tunnel: w793 -> [w858]
            tunnel: [w857] -> w792
            tunnel: [w856] -> w790
            tunnel: w741 -> [w855]
            tunnel: w739 -> [w854]
            tunnel: [w855] -> w738
            tunnel: [w854] -> w737
            tunnel: w721 -> [w853]
            tunnel: w719 -> [w849]
            tunnel: [w848] -> w717
            tunnel: [w847] -> w716
            tunnel: [w846] -> w715
            tunnel: w714 -> [w846]
            tunnel: w677 -> [w845]
            tunnel: [w845] -> w676
            tunnel: w792 -> [w867]
            tunnel: [w867] -> w791
            tunnel: w790 -> [w866]
            tunnel: [w866] -> w789
            tunnel: [w865] -> w734
            tunnel: w738 -> [w865]
            tunnel: [w864] -> _
            tunnel: w737 -> [w864]
            tunnel: [w864] -> w733
            tunnel: [w863] -> w713
            tunnel: w717 -> [w863]
            tunnel: w716 -> [w862]
            tunnel: [w861] -> w710
            tunnel: w715 -> [w861]
            tunnel: [w862] -> w712
            tunnel: w676 -> [w860]
            tunnel: [w860] -> w675
            frame #0 {
              # "7 jet pump\n6 push pump\n5 HD pump"
              n175 = call-poly <vilib>:"DAQmx Write.vi"("task/channels in"=w829, "data"=TRUE ("new element/subarray"), "error in"=w827) -> ("task out"=w828:refnum<k21>, "error out"=w826:errorcluster)  [unwired: 10 in, 1 out]
              n176 = Initialize Array(FALSE, 8 ("dimension size")) -> (w840:bool[])
              n177 = Replace Array Subset(array=w840, new element #1=TRUE ("new element/subarray"), index #1=7 ("index"), new element #2=TRUE ("new element/subarray"), index #2=6 ("index"), new element #3=TRUE ("new element/subarray"), index #3=5 ("index"), new element #4=TRUE ("new element/subarray"), index #4=1 ("index")) -> ()  [unwired: 1 out]
              n178 = call-poly <vilib>:"DAQmx Write.vi"("task/channels in"=w825, "data"=TRUE, "error in"=w823) -> ("task out"=w820:refnum<k21>)  [unwired: 10 in, 2 out]
              n179 = call-poly <vilib>:"DAQmx Write.vi"("task/channels in"=w819, "data"=FALSE) -> ("task out"=w817:refnum<k21>)  [unwired: 11 in, 2 out]
              n180 = Wait (ms)(milliseconds to wait=u32 50) -> ()  [unwired: 1 out]
            }
            frame #1 {
              # "start"
              n181 = call-poly <vilib>:"DAQmx Write.vi"("task/channels in"=w859, "data"=TRUE, "error in"=w858) -> ("task out"=w857:refnum<k21>, "error out"=w856:errorcluster)  [unwired: 10 in, 1 out]
              n182 = call-poly <vilib>:"DAQmx Write.vi"("task/channels in"=w853, "data"=TRUE) -> ("task out"=w848:refnum<k21>)  [unwired: 11 in, 2 out]
              n183 = call-poly <vilib>:"DAQmx Write.vi"("task/channels in"=w849, "data"=TRUE) -> ("task out"=w847:refnum<k21>)  [unwired: 11 in, 2 out]
            }
            frame #2 {
              n184 = Wait (ms)(milliseconds to wait=u32 50) -> ()  [unwired: 1 out]
            }
          }
          n185 = flat-sequence {
            tunnel: w694 -> [w816]
            tunnel: [w816] -> w693
            tunnel: [w815] -> w692
            tunnel: w691 -> [w814]
            tunnel: [w813] -> w690
            frame #0 {
              n186 = Tick Count (ms)() -> (millisecond timer value=w815:u32)
              n187 = Subtract(x=w815, y=w814) -> (x-y=w813:u32)
            }
          }
          n188 = call-poly <vilib>:"DAQmx Write.vi"("task/channels in"=w732, "data"=FALSE, "error in"=w731) -> ("task out"=w749:refnum<k21>, "error out"=w748:errorcluster)  [unwired: 10 in, 1 out]
          n189 = call-poly <vilib>:"DAQmx Write.vi"("task/channels in"=w709, "data"=FALSE) -> ("task out"=w705:refnum<k21>)  [unwired: 11 in, 2 out]
          n190 = while {
            tunnel: w749 -> [w892]
            tunnel: [w892] -> w775
            tunnel: w748 -> [w891]
            tunnel: [w891] -> w774
            tunnel: [w882] -> w771
            tunnel: [w881] -> w770
            tunnel: w786 -> [w888]
            tunnel: [w889] -> w746
            tunnel: w693 -> [w885]
            tunnel: w736 -> [w884]
            tunnel: w735 -> [w883]
            tunnel: w705 -> [w879]
            tunnel: [w879] -> w704
            tunnel: [w878] -> w700
            tunnel: [w877] -> w699
            tunnel: w698 -> [w874]
            tunnel: w697 -> [w873]
            tunnel: [w872] -> w686
            tunnel: w674 -> [w871]
            tunnel: [w869] -> w673
            stop <- w889 stop-if-true
            n191 = call-poly <vilib>:"DAQmx Write.vi"("task/channels in"=w884, "data"=FALSE, "error in"=w883) -> ("task out"=w882:refnum<k21>, "error out"=w881:errorcluster)  [unwired: 10 in, 1 out]
            n192 = call-poly <vilib>:"DAQmx Write.vi"("task/channels in"=w874, "data"=FALSE) -> ("task out"=w877:refnum<k21>)  [unwired: 11 in, 2 out]
            n193 = Wait (ms)(milliseconds to wait=u32 1000) -> ()  [unwired: 1 out]
            n194 = And(x=w888, y="next loop") -> (x .and. y?=w886:bool)
            n195 = call-poly <vilib>:"DAQmx Write.vi"("task/channels in"=w871, "data"=FALSE) -> ("task out"=w869:refnum<k21>)  [unwired: 11 in, 2 out]
            n196 = call-poly <vilib>:"DAQmx Write.vi"("task/channels in"=w873, "data"=FALSE) -> ("task out"=w878:refnum<k21>)  [unwired: 11 in, 2 out]
            n197 = Or(x=w886, y=w885) -> (x .or. y?=w889:bool)
            n198 = call <vilib>:"High Resolution Relative Seconds.vi"() -> ("relative seconds"=w872:dbl)
          }
          n199 = Subtract(x=w686, y=w687) -> (x-y=w683:dbl)
          n200 = Insert Into Array(array=w688, index=w684, new element=w683) -> (w685:dbl[])
          n201 = Greater?(x=w683, y="TIME THRESHOLD") -> (0:w681:bool)
          n202 = Or(x=w746, y=w693) -> (x .or. y?=w745:bool)
          n203 = call <vilib>:"DAQmx Stop Task.vi"("task/channels in"=w700) -> ("task out"=w701:refnum<k21>, "error out"=w707:errorcluster)  [unwired: 13 in]
          n204 = call <vilib>:"DAQmx Stop Task.vi"("task/channels in"=w699) -> ("task out"=w702:refnum<k21>, "error out"=w708:errorcluster)  [unwired: 13 in]
          n205 = call <vilib>:"DAQmx Stop Task.vi"("task/channels in"=w704) -> ("task out"=w703:refnum<k21>, "error out"=w706:errorcluster)  [unwired: 13 in]
          n206 = call <vilib>:"DAQmx Stop Task.vi"("task/channels in"=w771, "error in"=w770) -> ("task out"=w773:refnum<k21>, "error out"=w772:errorcluster)  [unwired: 12 in]
          n207 = call <vilib>:"DAQmx Stop Task.vi"("task/channels in"=w775, "error in"=w774) -> ("task out"=w777:refnum<k21>, "error out"=w776:errorcluster)  [unwired: 12 in]
          n208 = call <vilib>:"DAQmx Stop Task.vi"("task/channels in"=w673) -> ("task out"=w672:refnum<k21>)  [unwired: 13 in, 1 out]
          n209 = call <vilib>:"DAQmx Clear Task.vi"("task in"=w773, "error in"=w772) -> ()  [unwired: 13 in, 1 out]
          n210 = call <vilib>:"DAQmx Clear Task.vi"("task in"=w701, "error in"=w707) -> ()  [unwired: 13 in, 1 out]
          n211 = call <vilib>:"DAQmx Clear Task.vi"("task in"=w703, "error in"=w706) -> ()  [unwired: 13 in, 1 out]
          n212 = call <vilib>:"DAQmx Clear Task.vi"("task in"=w702, "error in"=w708) -> ()  [unwired: 13 in, 1 out]
          n213 = call <vilib>:"DAQmx Clear Task.vi"("task in"=w777, "error in"=w776) -> ()  [unwired: 13 in, 1 out]
          n214 = call <vilib>:"DAQmx Clear Task.vi"("task in"=w672) -> ()  [unwired: 14 in, 1 out]
          n215 = call <vilib>:"DAQmx Stop Task.vi"("task/channels in"=w751, "error in"=w750) -> ("task out"=w753:refnum<k21>, "error out"=w752:errorcluster)  [unwired: 12 in]
          n216 = call <vilib>:"DAQmx Clear Task.vi"("task in"=w753, "error in"=w752) -> ()  [unwired: 13 in, 1 out]
          "#triggers" <- w787
          "Numeric 7" <- w666
        }
        n217 = case shown="True" w597 {
          tunnel: w598 -> [w635 w637]
          tunnel: [w635 w636] -> w596
          frame False {
          }
          frame True {
            n218 = Increment(x=w637) -> (x+1=w636:i32)
          }
        }
        n219 = local read "tube changing #"() -> (w593:i32)
        n220 = local read "tube to stop"() -> (w581:i32)
        n221 = local read "Continuous\nacquisition"() -> (w599:bool)
        n222 = Greater?(x=w583, y=w581) -> (0:w582:bool)
        n223 = Less?(x=w593, y=10) -> (x < y?=w590:bool)
        n224 = Greater?(x=w596, y="# BEFORE GO DOWN") -> (0:w591:bool)
        n225 = And(x=w591, y=w590) -> (x .and. y?=w589:bool)
        n226 = case shown="True" w599 {
          tunnel: [states."Edgehunting" w643] -> w633
          tunnel: w624 -> [_ w642]
          tunnel: w589 -> [_ w641]
          tunnel: w584 -> [_ w640]
          tunnel: w582 -> [_ w639]
          frame False {
          }
          frame True {
            n227 = case shown="False" w641 {
              tunnel: [w647 states."Edgehunting"] -> w643
              tunnel: w642 -> [w646 _]
              tunnel: w640 -> [w645 _]
              tunnel: w639 -> [w644 _]
              frame False {
                n228 = case shown="False" w646 {
                  tunnel: [w650 w659] -> w647
                  tunnel: w645 -> [w649 w656]
                  tunnel: w644 -> [w648 w658]
                  frame False {
                    n229 = case shown="True" w649 {
                      tunnel: [states."Edgehunting" w653] -> w650
                      tunnel: w648 -> [_ w652]
                      frame False {
                      }
                      frame True {
                        n230 = case shown="True" w652 {
                          tunnel: [states."robotic arm" states."Chilling"] -> w653
                          frame False {
                          }
                          frame True {
                          }
                        }
                      }
                    }
                  }
                  frame True {
                    n231 = Not(x=w658) -> (.not. x?=w657:bool)
                    n232 = case shown="True" w656 {
                      tunnel: [states."reverse" w662] -> w659
                      tunnel: w657 -> [_ w661]
                      frame False {
                      }
                      frame True {
                        n233 = case shown="True" w661 {
                          tunnel: [states."Close" states."robotic arm"] -> w662
                          frame False {
                          }
                          frame True {
                          }
                        }
                      }
                    }
                  }
                }
              }
              frame True {
              }
            }
          }
        }
      }
      frame "tube position" {
        n234 = Increment(x=w936) -> (x+1=w935:i32)
        n235 = stacked-sequence {
          tunnel: FALSE ("Main/Sub") -> [_ w976]
          tunnel: "tb Pulses to move" -> [_ w973]
          tunnel: "tube Direction" -> [_ w972]
          tunnel: "\r\n" -> [_ w970]
          tunnel: [_ w971] -> _
          tunnel: [_ w970] -> _
          frame #0 {
            (unwired) u32 2000 ("High Speed")
            (unwired) TRUE ("Range")
            (unwired) u8 2 ("Axis Count")
            (unwired) u8 2 items=["0", "1", "2", "3", "4"] ("Axis Number")
            (unwired) u16 100 ("Acceleration Time")
            (unwired) u32 100 ("Low Speed")
          }
          frame #1 {
            w974 = u8 1 items=["0", "1", "2", "3", "4"] ("Axis Number")
            n236 = call "RS232C_Move.vi"("Axis Count"=u8 2, "Axis Number"=w974, "Pulse Number"=w973, "Direction"=w972, "Delimiter"=w970, "Main/Sub"=w976) -> ("OK Done"=w971:bool)  [unwired: 1 in, 1 out]
          }
        }
        n237 = local read "Continuous\nacquisition"() -> (w951:bool)
        n238 = case shown="False" w951 {
          tunnel: [states."Chilling" states."auto imaging"] -> w952
          frame False {
          }
          frame True {
          }
        }
      }
      frame "antic\n" {
        n239 = Increment(x=w1037) -> (x+1=w979:i32)
        n240 = call-poly <vilib>:"DAQmx Create Virtual Channel.vi"("lines"=tag "Dev1/port1/line5") -> ("task out"=w1043:refnum<k21>, "error out"=w1042:errorcluster)  [unwired: 13 in]
        n241 = call-poly <vilib>:"DAQmx Create Virtual Channel.vi"("lines"=tag "Dev1/port0/line7") -> ("task out"=w1026:refnum<k21>, "error out"=w1025:errorcluster)  [unwired: 13 in]
        n242 = call-poly <vilib>:"DAQmx Create Virtual Channel.vi"("lines"=tag "Dev1/port0/line4") -> ("task out"=w1050:refnum<k21>, "error out"=w1049:errorcluster)  [unwired: 13 in]
        n243 = call <vilib>:"DAQmx Start Task.vi"("task/channels in"=w1043, "error in"=w1042) -> ("task out"=w1040:refnum<k21>, "error out"=w1039:errorcluster)  [unwired: 12 in]
        n244 = call <vilib>:"DAQmx Start Task.vi"("task/channels in"=w1050, "error in"=w1049) -> ("task out"=w1048:refnum<k21>, "error out"=w1047:errorcluster)  [unwired: 12 in]
        n245 = call <vilib>:"DAQmx Start Task.vi"("task/channels in"=w1026, "error in"=w1025) -> ("task out"=w1023:refnum<k21>, "error out"=w1022:errorcluster)  [unwired: 12 in]
        n246 = stacked-sequence {
          seq-local: [w1070 _ _ _ _ _ _ _ _ _] -> [_ w1083 _ _ _ _ _ _ _ _]
          seq-local: [w1069 _ _ _ _ _ _ _ _ _] -> [_ w1082 _ _ _ _ _ _ _ _]
          seq-local: [w1064 _ _ _ _ _ _ _ _ _] -> [_ w1077 _ _ _ _ _ _ _ _]
          seq-local: [w1063 _ _ _ _ _ _ _ _ _] -> [_ w1076 _ _ _ _ _ _ _ _]
          seq-local: [w1061 _ _ _ _ _ _ _ _ _] -> [_ w1075 _ _ _ _ _ _ _ _]
          seq-local: [w1060 _ _ _ _ _ _ _ _ _] -> [_ w1074 _ _ _ _ _ _ _ _]
          seq-local: [_ w1081 _ _ _ _ _ _ _ _] -> [_ _ w1093 _ _ _ _ _ _ _]
          seq-local: [_ w1080 _ _ _ _ _ _ _ _] -> [_ _ w1092 _ _ _ _ _ _ _]
          seq-local: [_ w1077 _ _ _ _ _ _ _ _] -> [_ _ w1087 _ _ _ _ _ _ _]
          seq-local: [_ w1076 _ _ _ _ _ _ _ _] -> [_ _ w1086 _ _ _ _ _ _ _]
          seq-local: [_ w1075 _ _ _ _ _ _ _ _] -> [_ _ w1085 _ _ _ _ _ _ _]
          seq-local: [_ w1074 _ _ _ _ _ _ _ _] -> [_ _ w1084 _ _ _ _ _ _ _]
          seq-local: [_ _ w1091 _ _ _ _ _ _ _] -> [_ _ _ w1103 _ _ _ _ _ _]
          seq-local: [_ _ w1090 _ _ _ _ _ _ _] -> [_ _ _ w1102 _ _ _ _ _ _]
          seq-local: [_ _ w1087 _ _ _ _ _ _ _] -> [_ _ _ w1097 _ _ _ _ _ _]
          seq-local: [_ _ w1086 _ _ _ _ _ _ _] -> [_ _ _ w1096 _ _ _ _ _ _]
          seq-local: [_ _ w1085 _ _ _ _ _ _ _] -> [_ _ _ w1095 _ _ _ _ _ _]
          seq-local: [_ _ w1084 _ _ _ _ _ _ _] -> [_ _ _ w1094 _ _ _ _ _ _]
          seq-local: [_ _ _ w1101 _ _ _ _ _ _] -> [_ _ _ _ w1113 _ _ _ _ _]
          seq-local: [_ _ _ w1100 _ _ _ _ _ _] -> [_ _ _ _ w1112 _ _ _ _ _]
          seq-local: [_ _ _ w1097 _ _ _ _ _ _] -> [_ _ _ _ w1107 _ _ _ _ _]
          seq-local: [_ _ _ w1096 _ _ _ _ _ _] -> [_ _ _ _ w1106 _ _ _ _ _]
          seq-local: [_ _ _ w1095 _ _ _ _ _ _] -> [_ _ _ _ w1105 _ _ _ _ _]
          seq-local: [_ _ _ w1094 _ _ _ _ _ _] -> [_ _ _ _ w1104 _ _ _ _ _]
          seq-local: [_ _ _ _ w1110 _ _ _ _ _] -> [_ _ _ _ _ w1120 _ _ _ _]
          seq-local: [_ _ _ _ w1109 _ _ _ _ _] -> [_ _ _ _ _ w1118 _ _ _ _]
          seq-local: [_ _ _ _ w1107 _ _ _ _ _] -> [_ _ _ _ _ w1123 _ _ _ _]
          seq-local: [_ _ _ _ w1106 _ _ _ _ _] -> [_ _ _ _ _ w1122 _ _ _ _]
          seq-local: [_ _ _ _ w1105 _ _ _ _ _] -> [_ _ _ _ _ w1115 _ _ _ _]
          seq-local: [_ _ _ _ w1104 _ _ _ _ _] -> [_ _ _ _ _ w1114 _ _ _ _]
          seq-local: [_ _ _ _ _ w1119 _ _ _ _] -> [_ _ _ _ _ _ w1128 _ _ _]
          seq-local: [_ _ _ _ _ w1117 _ _ _ _] -> [_ _ _ _ _ _ w1130 _ _ _]
          seq-local: [_ _ _ _ _ w1123 _ _ _ _] -> [_ _ _ _ _ _ w1133 _ _ _]
          seq-local: [_ _ _ _ _ w1122 _ _ _ _] -> [_ _ _ _ _ _ w1132 _ _ _]
          seq-local: [_ _ _ _ _ w1115 _ _ _ _] -> [_ _ _ _ _ _ w1125 _ _ _]
          seq-local: [_ _ _ _ _ w1114 _ _ _ _] -> [_ _ _ _ _ _ w1124 _ _ _]
          seq-local: [_ _ _ _ _ _ w1127 _ _ _] -> [_ _ _ _ _ _ _ w1138 _ _]
          seq-local: [_ _ _ _ _ _ w1129 _ _ _] -> [_ _ _ _ _ _ _ w1140 _ _]
          seq-local: [_ _ _ _ _ _ w1133 _ _ _] -> [_ _ _ _ _ _ _ w1143 _ _]
          seq-local: [_ _ _ _ _ _ w1132 _ _ _] -> [_ _ _ _ _ _ _ w1142 _ _]
          seq-local: [_ _ _ _ _ _ w1125 _ _ _] -> [_ _ _ _ _ _ _ w1135 _ _]
          seq-local: [_ _ _ _ _ _ w1124 _ _ _] -> [_ _ _ _ _ _ _ w1134 _ _]
          seq-local: [_ _ _ _ _ _ _ w1137 _ _] -> [_ _ _ _ _ _ _ _ w1150 _]
          seq-local: [_ _ _ _ _ _ _ w1139 _ _] -> [_ _ _ _ _ _ _ _ w1149 _]
          seq-local: [_ _ _ _ _ _ _ w1143 _ _] -> [_ _ _ _ _ _ _ _ w1153 _]
          seq-local: [_ _ _ _ _ _ _ w1142 _ _] -> [_ _ _ _ _ _ _ _ w1152 _]
          seq-local: [_ _ _ _ _ _ _ w1135 _ _] -> [_ _ _ _ _ _ _ _ w1145 _]
          seq-local: [_ _ _ _ _ _ _ w1134 _ _] -> [_ _ _ _ _ _ _ _ w1144 _]
          seq-local: [_ _ _ _ _ _ _ _ w1147 _] -> [_ _ _ _ _ _ _ _ _ w1169]
          seq-local: [_ _ _ _ _ _ _ _ w1148 _] -> [_ _ _ _ _ _ _ _ _ w1159]
          seq-local: [_ _ _ _ _ _ _ _ w1153 _] -> [_ _ _ _ _ _ _ _ _ w1164]
          seq-local: [_ _ _ _ _ _ _ _ w1152 _] -> [_ _ _ _ _ _ _ _ _ w1163]
          seq-local: [_ _ _ _ _ _ _ _ w1145 _] -> [_ _ _ _ _ _ _ _ _ w1157]
          seq-local: [_ _ _ _ _ _ _ _ w1144 _] -> [_ _ _ _ _ _ _ _ _ w1156]
          tunnel: w1048 -> [w1073 _ _ _ _ _ _ _ _ _]
          tunnel: w1047 -> [w1072 _ _ _ _ _ _ _ _ _]
          tunnel: w1040 -> [w1067 _ _ _ _ _ _ _ _ _]
          tunnel: w1039 -> [w1066 _ _ _ _ _ _ _ _ _]
          tunnel: w1023 -> [w1059 _ _ _ _ _ _ _ _ _]
          tunnel: w1022 -> [w1058 _ _ _ _ _ _ _ _ _]
          tunnel: [_ _ _ _ _ _ _ _ _ w1167] -> w1021
          tunnel: [_ _ _ _ _ _ _ _ _ w1166] -> w1020
          tunnel: [_ _ _ _ _ _ _ _ _ w1162] -> w1019
          tunnel: [_ _ _ _ _ _ _ _ _ w1161] -> w1018
          tunnel: [_ _ _ _ _ _ _ _ _ w1155] -> w1017
          tunnel: [_ _ _ _ _ _ _ _ _ w1154] -> w1016
          frame #0 {
            n247 = call-poly <vilib>:"DAQmx Write.vi"("task/channels in"=w1067, "data"=TRUE, "error in"=w1066) -> ("task out"=w1064:refnum<k21>, "error out"=w1063:errorcluster)  [unwired: 10 in, 1 out]
            n248 = call-poly <vilib>:"DAQmx Write.vi"("task/channels in"=w1059, "data"=TRUE, "error in"=w1058) -> ("task out"=w1061:refnum<k21>, "error out"=w1060:errorcluster)  [unwired: 10 in, 1 out]
            n249 = call-poly <vilib>:"DAQmx Write.vi"("task/channels in"=w1073, "data"=TRUE, "error in"=w1072) -> ("task out"=w1070:refnum<k21>, "error out"=w1069:errorcluster)  [unwired: 10 in, 1 out]
            n250 = Wait (ms)(milliseconds to wait=u32 300) -> ()  [unwired: 1 out]
          }
          frame #1 {
            n251 = call-poly <vilib>:"DAQmx Write.vi"("task/channels in"=w1083, "data"=FALSE, "error in"=w1082) -> ("task out"=w1081:refnum<k21>, "error out"=w1080:errorcluster)  [unwired: 10 in, 1 out]
            n252 = Wait (ms)(milliseconds to wait=u32 300) -> ()  [unwired: 1 out]
          }
          frame #2 {
            n253 = call-poly <vilib>:"DAQmx Write.vi"("task/channels in"=w1093, "data"=TRUE, "error in"=w1092) -> ("task out"=w1091:refnum<k21>, "error out"=w1090:errorcluster)  [unwired: 10 in, 1 out]
            n254 = Wait (ms)(milliseconds to wait=u32 300) -> ()  [unwired: 1 out]
          }
          frame #3 {
            n255 = call-poly <vilib>:"DAQmx Write.vi"("task/channels in"=w1103, "data"=FALSE, "error in"=w1102) -> ("task out"=w1101:refnum<k21>, "error out"=w1100:errorcluster)  [unwired: 10 in, 1 out]
            n256 = Wait (ms)(milliseconds to wait=u32 300) -> ()  [unwired: 1 out]
          }
          frame #4 {
            n257 = call-poly <vilib>:"DAQmx Write.vi"("task/channels in"=w1113, "data"=TRUE, "error in"=w1112) -> ("task out"=w1110:refnum<k21>, "error out"=w1109:errorcluster)  [unwired: 10 in, 1 out]
            n258 = Wait (ms)(milliseconds to wait=u32 300) -> ()  [unwired: 1 out]
          }
          frame #5 {
            n259 = Wait (ms)(milliseconds to wait=u32 300) -> ()  [unwired: 1 out]
            n260 = call-poly <vilib>:"DAQmx Write.vi"("task/channels in"=w1120, "data"=FALSE, "error in"=w1118) -> ("task out"=w1119:refnum<k21>, "error out"=w1117:errorcluster)  [unwired: 10 in, 1 out]
          }
          frame #6 {
            n261 = Wait (ms)(milliseconds to wait=u32 300) -> ()  [unwired: 1 out]
            n262 = call-poly <vilib>:"DAQmx Write.vi"("task/channels in"=w1128, "data"=TRUE, "error in"=w1130) -> ("task out"=w1127:refnum<k21>, "error out"=w1129:errorcluster)  [unwired: 10 in, 1 out]
          }
          frame #7 {
            n263 = call-poly <vilib>:"DAQmx Write.vi"("task/channels in"=w1138, "data"=FALSE, "error in"=w1140) -> ("task out"=w1137:refnum<k21>, "error out"=w1139:errorcluster)  [unwired: 10 in, 1 out]
            n264 = Wait (ms)(milliseconds to wait=u32 300) -> ()  [unwired: 1 out]
          }
          frame #8 {
            n265 = call-poly <vilib>:"DAQmx Write.vi"("task/channels in"=w1150, "data"=TRUE, "error in"=w1149) -> ("task out"=w1147:refnum<k21>, "error out"=w1148:errorcluster)  [unwired: 10 in, 1 out]
            n266 = Wait (ms)(milliseconds to wait=u32 300) -> ()  [unwired: 1 out]
          }
          frame #9 {
            n267 = call-poly <vilib>:"DAQmx Write.vi"("task/channels in"=w1169, "data"=TRUE, "error in"=w1159) -> ("task out"=w1167:refnum<k21>, "error out"=w1166:errorcluster)  [unwired: 10 in, 1 out]
            n268 = call-poly <vilib>:"DAQmx Write.vi"("task/channels in"=w1164, "data"=FALSE, "error in"=w1163) -> ("task out"=w1162:refnum<k21>, "error out"=w1161:errorcluster)  [unwired: 10 in, 1 out]
            n269 = call-poly <vilib>:"DAQmx Write.vi"("task/channels in"=w1157, "data"=TRUE, "error in"=w1156) -> ("task out"=w1155:refnum<k21>, "error out"=w1154:errorcluster)  [unwired: 10 in, 1 out]
            n270 = Wait (ms)(milliseconds to wait=u32 300) -> ()  [unwired: 1 out]
          }
        }
        n271 = stacked-sequence {
          seq-local: [w1182 _ _ _ _ _ _ _ _ _] -> [_ w1195 _ _ _ _ _ _ _ _]
          seq-local: [w1181 _ _ _ _ _ _ _ _ _] -> [_ w1194 _ _ _ _ _ _ _ _]
          seq-local: [w1176 _ _ _ _ _ _ _ _ _] -> [_ w1189 _ _ _ _ _ _ _ _]
          seq-local: [w1175 _ _ _ _ _ _ _ _ _] -> [_ w1188 _ _ _ _ _ _ _ _]
          seq-local: [w1173 _ _ _ _ _ _ _ _ _] -> [_ w1187 _ _ _ _ _ _ _ _]
          seq-local: [w1172 _ _ _ _ _ _ _ _ _] -> [_ w1186 _ _ _ _ _ _ _ _]
          seq-local: [_ w1193 _ _ _ _ _ _ _ _] -> [_ _ w1205 _ _ _ _ _ _ _]
          seq-local: [_ w1192 _ _ _ _ _ _ _ _] -> [_ _ w1204 _ _ _ _ _ _ _]
          seq-local: [_ w1189 _ _ _ _ _ _ _ _] -> [_ _ w1200 _ _ _ _ _ _ _]
          seq-local: [_ w1188 _ _ _ _ _ _ _ _] -> [_ _ w1199 _ _ _ _ _ _ _]
          seq-local: [_ w1187 _ _ _ _ _ _ _ _] -> [_ _ w1198 _ _ _ _ _ _ _]
          seq-local: [_ w1186 _ _ _ _ _ _ _ _] -> [_ _ w1197 _ _ _ _ _ _ _]
          seq-local: [_ _ w1203 _ _ _ _ _ _ _] -> [_ _ _ w1215 _ _ _ _ _ _]
          seq-local: [_ _ w1202 _ _ _ _ _ _ _] -> [_ _ _ w1214 _ _ _ _ _ _]
          seq-local: [_ _ w1200 _ _ _ _ _ _ _] -> [_ _ _ w1209 _ _ _ _ _ _]
          seq-local: [_ _ w1199 _ _ _ _ _ _ _] -> [_ _ _ w1208 _ _ _ _ _ _]
          seq-local: [_ _ w1198 _ _ _ _ _ _ _] -> [_ _ _ w1207 _ _ _ _ _ _]
          seq-local: [_ _ w1197 _ _ _ _ _ _ _] -> [_ _ _ w1206 _ _ _ _ _ _]
          seq-local: [_ _ _ w1213 _ _ _ _ _ _] -> [_ _ _ _ w1225 _ _ _ _ _]
          seq-local: [_ _ _ w1212 _ _ _ _ _ _] -> [_ _ _ _ w1224 _ _ _ _ _]
          seq-local: [_ _ _ w1209 _ _ _ _ _ _] -> [_ _ _ _ w1219 _ _ _ _ _]
          seq-local: [_ _ _ w1208 _ _ _ _ _ _] -> [_ _ _ _ w1218 _ _ _ _ _]
          seq-local: [_ _ _ w1207 _ _ _ _ _ _] -> [_ _ _ _ w1217 _ _ _ _ _]
          seq-local: [_ _ _ w1206 _ _ _ _ _ _] -> [_ _ _ _ w1216 _ _ _ _ _]
          seq-local: [_ _ _ _ w1222 _ _ _ _ _] -> [_ _ _ _ _ w1232 _ _ _ _]
          seq-local: [_ _ _ _ w1221 _ _ _ _ _] -> [_ _ _ _ _ w1230 _ _ _ _]
          seq-local: [_ _ _ _ w1219 _ _ _ _ _] -> [_ _ _ _ _ w1235 _ _ _ _]
          seq-local: [_ _ _ _ w1218 _ _ _ _ _] -> [_ _ _ _ _ w1234 _ _ _ _]
          seq-local: [_ _ _ _ w1217 _ _ _ _ _] -> [_ _ _ _ _ w1227 _ _ _ _]
          seq-local: [_ _ _ _ w1216 _ _ _ _ _] -> [_ _ _ _ _ w1226 _ _ _ _]
          seq-local: [_ _ _ _ _ w1231 _ _ _ _] -> [_ _ _ _ _ _ w1240 _ _ _]
          seq-local: [_ _ _ _ _ w1229 _ _ _ _] -> [_ _ _ _ _ _ w1242 _ _ _]
          seq-local: [_ _ _ _ _ w1235 _ _ _ _] -> [_ _ _ _ _ _ w1245 _ _ _]
          seq-local: [_ _ _ _ _ w1234 _ _ _ _] -> [_ _ _ _ _ _ w1244 _ _ _]
          seq-local: [_ _ _ _ _ w1227 _ _ _ _] -> [_ _ _ _ _ _ w1237 _ _ _]
          seq-local: [_ _ _ _ _ w1226 _ _ _ _] -> [_ _ _ _ _ _ w1236 _ _ _]
          seq-local: [_ _ _ _ _ _ w1239 _ _ _] -> [_ _ _ _ _ _ _ w1250 _ _]
          seq-local: [_ _ _ _ _ _ w1241 _ _ _] -> [_ _ _ _ _ _ _ w1252 _ _]
          seq-local: [_ _ _ _ _ _ w1245 _ _ _] -> [_ _ _ _ _ _ _ w1255 _ _]
          seq-local: [_ _ _ _ _ _ w1244 _ _ _] -> [_ _ _ _ _ _ _ w1254 _ _]
          seq-local: [_ _ _ _ _ _ w1237 _ _ _] -> [_ _ _ _ _ _ _ w1247 _ _]
          seq-local: [_ _ _ _ _ _ w1236 _ _ _] -> [_ _ _ _ _ _ _ w1246 _ _]
          seq-local: [_ _ _ _ _ _ _ w1249 _ _] -> [_ _ _ _ _ _ _ _ w1262 _]
          seq-local: [_ _ _ _ _ _ _ w1251 _ _] -> [_ _ _ _ _ _ _ _ w1261 _]
          seq-local: [_ _ _ _ _ _ _ w1255 _ _] -> [_ _ _ _ _ _ _ _ w1265 _]
          seq-local: [_ _ _ _ _ _ _ w1254 _ _] -> [_ _ _ _ _ _ _ _ w1264 _]
          seq-local: [_ _ _ _ _ _ _ w1247 _ _] -> [_ _ _ _ _ _ _ _ w1257 _]
          seq-local: [_ _ _ _ _ _ _ w1246 _ _] -> [_ _ _ _ _ _ _ _ w1256 _]
          seq-local: [_ _ _ _ _ _ _ _ w1259 _] -> [_ _ _ _ _ _ _ _ _ w1281]
          seq-local: [_ _ _ _ _ _ _ _ w1260 _] -> [_ _ _ _ _ _ _ _ _ w1271]
          seq-local: [_ _ _ _ _ _ _ _ w1265 _] -> [_ _ _ _ _ _ _ _ _ w1276]
          seq-local: [_ _ _ _ _ _ _ _ w1264 _] -> [_ _ _ _ _ _ _ _ _ w1275]
          seq-local: [_ _ _ _ _ _ _ _ w1257 _] -> [_ _ _ _ _ _ _ _ _ w1269]
          seq-local: [_ _ _ _ _ _ _ _ w1256 _] -> [_ _ _ _ _ _ _ _ _ w1268]
          tunnel: w1021 -> [w1185 _ _ _ _ _ _ _ _ _]
          tunnel: w1020 -> [w1184 _ _ _ _ _ _ _ _ _]
          tunnel: w1019 -> [w1179 _ _ _ _ _ _ _ _ _]
          tunnel: w1018 -> [w1178 _ _ _ _ _ _ _ _ _]
          tunnel: w1017 -> [w1171 _ _ _ _ _ _ _ _ _]
          tunnel: w1016 -> [w1170 _ _ _ _ _ _ _ _ _]
          tunnel: [_ _ _ _ _ _ _ _ _ w1279] -> w1005
          tunnel: [_ _ _ _ _ _ _ _ _ w1278] -> w1004
          tunnel: [_ _ _ _ _ _ _ _ _ w1274] -> w1007
          tunnel: [_ _ _ _ _ _ _ _ _ w1273] -> w1006
          tunnel: [_ _ _ _ _ _ _ _ _ w1267] -> w1009
          tunnel: [_ _ _ _ _ _ _ _ _ w1266] -> w1008
          frame #0 {
            n272 = Wait (ms)(milliseconds to wait=u32 300) -> ()  [unwired: 1 out]
            n273 = call-poly <vilib>:"DAQmx Write.vi"("task/channels in"=w1185, "data"=TRUE, "error in"=w1184) -> ("task out"=w1182:refnum<k21>, "error out"=w1181:errorcluster)  [unwired: 10 in, 1 out]
            n274 = call-poly <vilib>:"DAQmx Write.vi"("task/channels in"=w1179, "data"=TRUE, "error in"=w1178) -> ("task out"=w1176:refnum<k21>, "error out"=w1175:errorcluster)  [unwired: 10 in, 1 out]
            n275 = call-poly <vilib>:"DAQmx Write.vi"("task/channels in"=w1171, "data"=TRUE, "error in"=w1170) -> ("task out"=w1173:refnum<k21>, "error out"=w1172:errorcluster)  [unwired: 10 in, 1 out]
          }
          frame #1 {
            n276 = call-poly <vilib>:"DAQmx Write.vi"("task/channels in"=w1195, "data"=FALSE, "error in"=w1194) -> ("task out"=w1193:refnum<k21>, "error out"=w1192:errorcluster)  [unwired: 10 in, 1 out]
            n277 = Wait (ms)(milliseconds to wait=u32 300) -> ()  [unwired: 1 out]
          }
          frame #2 {
            n278 = call-poly <vilib>:"DAQmx Write.vi"("task/channels in"=w1205, "data"=TRUE, "error in"=w1204) -> ("task out"=w1203:refnum<k21>, "error out"=w1202:errorcluster)  [unwired: 10 in, 1 out]
            n279 = Wait (ms)(milliseconds to wait=u32 300) -> ()  [unwired: 1 out]
          }
          frame #3 {
            n280 = call-poly <vilib>:"DAQmx Write.vi"("task/channels in"=w1215, "data"=FALSE, "error in"=w1214) -> ("task out"=w1213:refnum<k21>, "error out"=w1212:errorcluster)  [unwired: 10 in, 1 out]
            n281 = Wait (ms)(milliseconds to wait=u32 300) -> ()  [unwired: 1 out]
          }
          frame #4 {
            n282 = call-poly <vilib>:"DAQmx Write.vi"("task/channels in"=w1225, "data"=TRUE, "error in"=w1224) -> ("task out"=w1222:refnum<k21>, "error out"=w1221:errorcluster)  [unwired: 10 in, 1 out]
            n283 = Wait (ms)(milliseconds to wait=u32 300) -> ()  [unwired: 1 out]
          }
          frame #5 {
            n284 = call-poly <vilib>:"DAQmx Write.vi"("task/channels in"=w1232, "data"=FALSE, "error in"=w1230) -> ("task out"=w1231:refnum<k21>, "error out"=w1229:errorcluster)  [unwired: 10 in, 1 out]
            n285 = Wait (ms)(milliseconds to wait=u32 300) -> ()  [unwired: 1 out]
          }
          frame #6 {
            n286 = call-poly <vilib>:"DAQmx Write.vi"("task/channels in"=w1240, "data"=TRUE, "error in"=w1242) -> ("task out"=w1239:refnum<k21>, "error out"=w1241:errorcluster)  [unwired: 10 in, 1 out]
            n287 = Wait (ms)(milliseconds to wait=u32 300) -> ()  [unwired: 1 out]
          }
          frame #7 {
            n288 = call-poly <vilib>:"DAQmx Write.vi"("task/channels in"=w1250, "data"=FALSE, "error in"=w1252) -> ("task out"=w1249:refnum<k21>, "error out"=w1251:errorcluster)  [unwired: 10 in, 1 out]
            n289 = Wait (ms)(milliseconds to wait=u32 300) -> ()  [unwired: 1 out]
          }
          frame #8 {
            n290 = call-poly <vilib>:"DAQmx Write.vi"("task/channels in"=w1262, "data"=TRUE, "error in"=w1261) -> ("task out"=w1259:refnum<k21>, "error out"=w1260:errorcluster)  [unwired: 10 in, 1 out]
            n291 = Wait (ms)(milliseconds to wait=u32 300) -> ()  [unwired: 1 out]
          }
          frame #9 {
            n292 = call-poly <vilib>:"DAQmx Write.vi"("task/channels in"=w1281, "data"=FALSE, "error in"=w1271) -> ("task out"=w1279:refnum<k21>, "error out"=w1278:errorcluster)  [unwired: 10 in, 1 out]
            n293 = call-poly <vilib>:"DAQmx Write.vi"("task/channels in"=w1276, "data"=FALSE, "error in"=w1275) -> ("task out"=w1274:refnum<k21>, "error out"=w1273:errorcluster)  [unwired: 10 in, 1 out]
            n294 = call-poly <vilib>:"DAQmx Write.vi"("task/channels in"=w1269, "data"=TRUE, "error in"=w1268) -> ("task out"=w1267:refnum<k21>, "error out"=w1266:errorcluster)  [unwired: 10 in, 1 out]
            n295 = Wait (ms)(milliseconds to wait=u32 300) -> ()  [unwired: 1 out]
          }
        }
        n296 = call <vilib>:"DAQmx Stop Task.vi"("task/channels in"=w1005, "error in"=w1004) -> ("task out"=w1015:refnum<k21>, "error out"=w1014:errorcluster)  [unwired: 12 in]
        n297 = call <vilib>:"DAQmx Stop Task.vi"("task/channels in"=w1007, "error in"=w1006) -> ("task out"=w1013:refnum<k21>, "error out"=w1012:errorcluster)  [unwired: 12 in]
        n298 = call <vilib>:"DAQmx Stop Task.vi"("task/channels in"=w1009, "error in"=w1008) -> ("task out"=w1011:refnum<k21>, "error out"=w1010:errorcluster)  [unwired: 12 in]
        n299 = call <vilib>:"DAQmx Clear Task.vi"("task in"=w1015, "error in"=w1014) -> ()  [unwired: 13 in, 1 out]
        n300 = call <vilib>:"DAQmx Clear Task.vi"("task in"=w1013, "error in"=w1012) -> ()  [unwired: 13 in, 1 out]
        n301 = call <vilib>:"DAQmx Clear Task.vi"("task in"=w1011, "error in"=w1010) -> ()  [unwired: 13 in, 1 out]
        n302 = Greater?(x=u32 5 ("y"), y=w979) -> (0:w1034:bool)
        n303 = local read "Continuous\nacquisition"() -> (w1035:bool)
        n304 = case shown="False" w1035 {
          tunnel: [states."Chilling" w1284] -> w1045
          tunnel: w1034 -> [_ w1283]
          frame False {
          }
          frame True {
            n305 = case shown="False" w1283 {
              tunnel: [states."auto imaging" states."Close"] -> w1284
              frame False {
              }
              frame True {
              }
            }
          }
        }
      }
      frame "reverse" {
        # "shower valve3"
        n306 = call-poly <vilib>:"DAQmx Create Virtual Channel.vi"("lines"=tag "Dev1/port0/line7") -> ("task out"=w1320:refnum<k21>, "error out"=w1321:errorcluster)  [unwired: 13 in]
        n307 = call-poly <vilib>:"DAQmx Create Virtual Channel.vi"("lines"=tag "Dev1/port0/line5") -> ("task out"=w1311:refnum<k21>)  [unwired: 13 in, 1 out]
        n308 = call-poly <vilib>:"DAQmx Write.vi"("task/channels in"=w1325, "data"=TRUE) -> ("task out"=w1323:refnum<k21>)  [unwired: 11 in, 2 out]
        n309 = call <vilib>:"DAQmx Start Task.vi"("task/channels in"=w1320, "error in"=w1321) -> ("task out"=w1317:refnum<k21>)  [unwired: 12 in, 1 out]
        n310 = call <vilib>:"DAQmx Start Task.vi"("task/channels in"=w1311) -> ("task out"=w1299:refnum<k21>)  [unwired: 13 in, 1 out]
        n311 = call-poly <vilib>:"DAQmx Create Virtual Channel.vi"("lines"=tag "Dev1/port0/line4") -> ("task out"=w1308:refnum<k21>)  [unwired: 13 in, 1 out]
        n312 = call-poly <vilib>:"DAQmx Write.vi"("task/channels in"=w1317, "data"=TRUE) -> ("task out"=w1316:refnum<k21>)  [unwired: 11 in, 2 out]
        n313 = call <vilib>:"DAQmx Start Task.vi"("task/channels in"=w1308) -> ("task out"=w1305:refnum<k21>)  [unwired: 13 in, 1 out]
        n314 = call-poly <vilib>:"DAQmx Write.vi"("task/channels in"=w1305, "data"=TRUE) -> ("task out"=w1302:refnum<k21>)  [unwired: 11 in, 2 out]
        n315 = stacked-sequence {
          seq-local: [w1359 _ _ _ _ _ _ _] -> [_ w1364 _ _ _ _ _ _]
          seq-local: [w1358 _ _ _ _ _ _ _] -> [_ w1363 _ _ _ _ _ _]
          seq-local: [w1357 _ _ _ _ _ _ _] -> [_ w1361 _ _ _ _ _ _]
          seq-local: [_ w1364 _ _ _ _ _ _] -> [_ _ w1370 _ _ _ _ _]
          seq-local: [_ w1363 _ _ _ _ _ _] -> [_ _ w1369 _ _ _ _ _]
          seq-local: [_ w1360 _ _ _ _ _ _] -> [_ _ w1368 _ _ _ _ _]
          seq-local: [_ _ w1370 _ _ _ _ _] -> [_ _ _ w1376 _ _ _ _]
          seq-local: [_ _ w1370 _ _ _ _ _] -> [_ _ _ w1375 _ _ _ _]
          seq-local: [_ _ w1369 _ _ _ _ _] -> [_ _ _ w1374 _ _ _ _]
          seq-local: [_ _ w1366 _ _ _ _ _] -> [_ _ _ w1373 _ _ _ _]
          seq-local: [_ _ _ w1376 _ _ _ _] -> [_ _ _ _ _ _ _ _]
          seq-local: [_ _ _ w1375 _ _ _ _] -> [_ _ _ _ w1382 _ _ _]
          seq-local: [_ _ _ w1374 _ _ _ _] -> [_ _ _ _ w1381 _ _ _]
          seq-local: [_ _ _ w1371 _ _ _ _] -> [_ _ _ _ w1380 _ _ _]
          seq-local: [_ _ _ _ w1382 _ _ _] -> [_ _ _ _ _ w1387 _ _]
          seq-local: [_ _ _ _ w1381 _ _ _] -> [_ _ _ _ _ w1386 _ _]
          seq-local: [_ _ _ _ w1378 _ _ _] -> [_ _ _ _ _ w1385 _ _]
          seq-local: [_ _ _ _ _ w1387 _ _] -> [_ _ _ _ _ _ _ _]
          seq-local: [_ _ _ _ _ w1386 _ _] -> [_ _ _ _ _ _ _ _]
          seq-local: [_ _ _ _ _ w1383 _ _] -> [_ _ _ _ _ _ w1391 _]
          seq-local: [_ _ _ _ _ _ w1389 _] -> [_ _ _ _ _ _ _ w1392]
          tunnel: "milliseconds to wait" -> [w1358 _ _ _ _ _ _ _]
          tunnel: "Flow Rate (5.00)" -> [w1359 _ _ _ _ _ _ _]
          tunnel: w1299 -> [w1357 _ _ _ _ _ _ _]
          tunnel: w1323 -> [_ _ _ _ _ _ _ w1401]
          tunnel: [_ _ _ _ _ _ _ w1399] -> w1287
          tunnel: w1316 -> [_ _ _ _ _ _ _ w1397]
          tunnel: [_ _ _ _ _ _ _ w1396] -> w1314
          tunnel: [_ _ _ _ _ _ _ w1395] -> w1303
          tunnel: w1302 -> [_ _ _ _ _ _ _ w1393]
          tunnel: [_ _ _ _ _ _ _ w1392] -> w1298
          frame #0 {
            (unwired) FALSE ("Boolean")
            n316 = Wait (ms)(milliseconds to wait=u32 1000) -> ()  [unwired: 1 out]
          }
          frame #1 {
            n317 = Wait (ms)(milliseconds to wait=w1363) -> ()  [unwired: 1 out]
            n318 = call-poly <vilib>:"DAQmx Write.vi"("task/channels in"=w1361, "data"=TRUE) -> ("task out"=w1360:refnum<k21>)  [unwired: 11 in, 2 out]
          }
          frame #2 {
            n319 = call-poly <vilib>:"DAQmx Write.vi"("task/channels in"=w1368, "data"=FALSE) -> ("task out"=w1366:refnum<k21>)  [unwired: 11 in, 2 out]
            n320 = Wait (ms)(milliseconds to wait=u32 500) -> ()  [unwired: 1 out]
          }
          frame #3 {
            (unwired) FALSE ("Boolean")
            n321 = call-poly <vilib>:"DAQmx Write.vi"("task/channels in"=w1373, "data"=TRUE) -> ("task out"=w1371:refnum<k21>)  [unwired: 11 in, 2 out]
          }
          frame #4 {
            n322 = call-poly <vilib>:"DAQmx Write.vi"("task/channels in"=w1380, "data"=FALSE) -> ("task out"=w1378:refnum<k21>)  [unwired: 11 in, 2 out]
            n323 = Wait (ms)(milliseconds to wait=u32 500) -> ()  [unwired: 1 out]
          }
          frame #5 {
            n324 = Wait (ms)(milliseconds to wait=w1386) -> ()  [unwired: 1 out]
            n325 = call-poly <vilib>:"DAQmx Write.vi"("task/channels in"=w1385, "data"=TRUE ("Boolean")) -> ("task out"=w1383:refnum<k21>)  [unwired: 11 in, 2 out]
          }
          frame #6 {
            n326 = call-poly <vilib>:"DAQmx Write.vi"("task/channels in"=w1391, "data"=FALSE) -> ("task out"=w1389:refnum<k21>)  [unwired: 11 in, 2 out]
            n327 = Wait (ms)(milliseconds to wait=u32 500) -> ()  [unwired: 1 out]
          }
          frame #7 {
            n328 = call-poly <vilib>:"DAQmx Write.vi"("task/channels in"=w1397, "data"=FALSE) -> ("task out"=w1396:refnum<k21>)  [unwired: 11 in, 2 out]
            n329 = call-poly <vilib>:"DAQmx Write.vi"("task/channels in"=w1401, "data"=FALSE) -> ("task out"=w1399:refnum<k21>)  [unwired: 11 in, 2 out]
            n330 = call-poly <vilib>:"DAQmx Write.vi"("task/channels in"=w1393, "data"=FALSE) -> ("task out"=w1395:refnum<k21>)  [unwired: 11 in, 2 out]
          }
        }
        n331 = call <vilib>:"DAQmx Stop Task.vi"("task/channels in"=w1314) -> ("task out"=w1315:refnum<k21>)  [unwired: 13 in, 1 out]
        n332 = call <vilib>:"DAQmx Stop Task.vi"("task/channels in"=w1303) -> ("task out"=w1306:refnum<k21>)  [unwired: 13 in, 1 out]
        n333 = call <vilib>:"DAQmx Stop Task.vi"("task/channels in"=w1298) -> ("task out"=w1309:refnum<k21>)  [unwired: 13 in, 1 out]
        n334 = call <vilib>:"DAQmx Clear Task.vi"("task in"=w1315) -> ()  [unwired: 14 in, 1 out]
        n335 = call <vilib>:"DAQmx Clear Task.vi"("task in"=w1306) -> ()  [unwired: 14 in, 1 out]
        n336 = call <vilib>:"DAQmx Clear Task.vi"("task in"=w1309) -> ()  [unwired: 14 in, 1 out]
        n337 = local read "Continuous\nacquisition"() -> (w1322:bool)
        n338 = case shown="True" w1322 {
          tunnel: [states."Chilling" states."antic\n"] -> w1328
          frame False {
          }
          frame True {
          }
        }
      }
      frame "light reverse" {
        # "valve 3"
        # "pinch valve v2"
        n339 = call-poly <vilib>:"DAQmx Create Virtual Channel.vi"("lines"=tag "Dev1/port0/line5") -> ("task out"=w1428:refnum<k21>)  [unwired: 13 in, 1 out]
        n340 = call-poly <vilib>:"DAQmx Create Virtual Channel.vi"("lines"=tag "Dev1/port0/line4") -> ("task out"=w1425:refnum<k21>)  [unwired: 13 in, 1 out]
        n341 = call <vilib>:"DAQmx Start Task.vi"("task/channels in"=w1428) -> ("task out"=w1416:refnum<k21>)  [unwired: 13 in, 1 out]
        n342 = call <vilib>:"DAQmx Start Task.vi"("task/channels in"=w1425) -> ("task out"=w1422:refnum<k21>)  [unwired: 13 in, 1 out]
        n343 = call-poly <vilib>:"DAQmx Create Virtual Channel.vi"("lines"=tag "Dev1/port0/line7") -> ("task out"=w1437:refnum<k21>, "error out"=w1438:errorcluster)  [unwired: 13 in]
        n344 = call-poly <vilib>:"DAQmx Write.vi"("task/channels in"=w1422, "data"=TRUE) -> ("task out"=w1419:refnum<k21>)  [unwired: 11 in, 2 out]
        n345 = call <vilib>:"DAQmx Start Task.vi"("task/channels in"=w1437, "error in"=w1438) -> ("task out"=w1434:refnum<k21>)  [unwired: 12 in, 1 out]
        n346 = call-poly <vilib>:"DAQmx Write.vi"("task/channels in"=w1434, "data"=TRUE) -> ("task out"=w1433:refnum<k21>)  [unwired: 11 in, 2 out]
        n347 = local read "Continuous\nacquisition"() -> (w1439:bool)
        n348 = call-poly <vilib>:"DAQmx Write.vi"("task/channels in"=w1443, "data"=TRUE) -> ("task out"=w1441:refnum<k21>)  [unwired: 11 in, 2 out]
        n349 = stacked-sequence {
          seq-local: [w1474 _ _ _ _ _ _ _] -> [_ w1478 _ _ _ _ _ _]
          seq-local: [w1473 _ _ _ _ _ _ _] -> [_ w1476 _ _ _ _ _ _]
          seq-local: [_ w1478 _ _ _ _ _ _] -> [_ _ w1483 _ _ _ _ _]
          seq-local: [_ w1475 _ _ _ _ _ _] -> [_ _ w1482 _ _ _ _ _]
          seq-local: [_ _ w1483 _ _ _ _ _] -> [_ _ _ w1487 _ _ _ _]
          seq-local: [_ _ w1480 _ _ _ _ _] -> [_ _ _ w1486 _ _ _ _]
          seq-local: [_ _ _ w1487 _ _ _ _] -> [_ _ _ _ w1492 _ _ _]
          seq-local: [_ _ _ w1484 _ _ _ _] -> [_ _ _ _ w1491 _ _ _]
          seq-local: [_ _ _ _ w1492 _ _ _] -> [_ _ _ _ _ w1496 _ _]
          seq-local: [_ _ _ _ w1489 _ _ _] -> [_ _ _ _ _ w1495 _ _]
          seq-local: [_ _ _ _ _ w1496 _ _] -> [_ _ _ _ _ _ _ _]
          seq-local: [_ _ _ _ _ w1493 _ _] -> [_ _ _ _ _ _ w1500 _]
          seq-local: [_ _ _ _ _ _ w1498 _] -> [_ _ _ _ _ _ _ w1501]
          tunnel: u32 1000 ("milliseconds to wait 2") -> [w1474 _ _ _ _ _ _ _]
          tunnel: w1416 -> [w1473 _ _ _ _ _ _ _]
          tunnel: w1441 -> [_ _ _ _ _ _ _ w1510]
          tunnel: [_ _ _ _ _ _ _ w1508] -> w1440
          tunnel: w1433 -> [_ _ _ _ _ _ _ w1506]
          tunnel: [_ _ _ _ _ _ _ w1505] -> w1431
          tunnel: [_ _ _ _ _ _ _ w1504] -> w1420
          tunnel: w1419 -> [_ _ _ _ _ _ _ w1502]
          tunnel: [_ _ _ _ _ _ _ w1501] -> w1415
          frame #0 {
            n350 = Wait (ms)(milliseconds to wait=u32 1000) -> ()  [unwired: 1 out]
          }
          frame #1 {
            n351 = Wait (ms)(milliseconds to wait=w1478) -> ()  [unwired: 1 out]
            n352 = call-poly <vilib>:"DAQmx Write.vi"("task/channels in"=w1476, "data"=TRUE) -> ("task out"=w1475:refnum<k21>)  [unwired: 11 in, 2 out]
          }
          frame #2 {
            n353 = call-poly <vilib>:"DAQmx Write.vi"("task/channels in"=w1482, "data"=FALSE) -> ("task out"=w1480:refnum<k21>)  [unwired: 11 in, 2 out]
            n354 = Wait (ms)(milliseconds to wait=u32 500) -> ()  [unwired: 1 out]
          }
          frame #3 {
            (unwired) FALSE ("Boolean")
            n355 = call-poly <vilib>:"DAQmx Write.vi"("task/channels in"=w1486, "data"=TRUE) -> ("task out"=w1484:refnum<k21>)  [unwired: 11 in, 2 out]
          }
          frame #4 {
            n356 = call-poly <vilib>:"DAQmx Write.vi"("task/channels in"=w1491, "data"=FALSE) -> ("task out"=w1489:refnum<k21>)  [unwired: 11 in, 2 out]
            n357 = Wait (ms)(milliseconds to wait=u32 500) -> ()  [unwired: 1 out]
          }
          frame #5 {
            n358 = Wait (ms)(milliseconds to wait=w1496) -> ()  [unwired: 1 out]
            n359 = call-poly <vilib>:"DAQmx Write.vi"("task/channels in"=w1495, "data"=TRUE ("Boolean")) -> ("task out"=w1493:refnum<k21>)  [unwired: 11 in, 2 out]
          }
          frame #6 {
            n360 = call-poly <vilib>:"DAQmx Write.vi"("task/channels in"=w1500, "data"=FALSE) -> ("task out"=w1498:refnum<k21>)  [unwired: 11 in, 2 out]
            n361 = Wait (ms)(milliseconds to wait=u32 500) -> ()  [unwired: 1 out]
          }
          frame #7 {
            n362 = call-poly <vilib>:"DAQmx Write.vi"("task/channels in"=w1506, "data"=FALSE) -> ("task out"=w1505:refnum<k21>)  [unwired: 11 in, 2 out]
            n363 = call-poly <vilib>:"DAQmx Write.vi"("task/channels in"=w1510, "data"=FALSE) -> ("task out"=w1508:refnum<k21>)  [unwired: 11 in, 2 out]
            n364 = call-poly <vilib>:"DAQmx Write.vi"("task/channels in"=w1502, "data"=FALSE) -> ("task out"=w1504:refnum<k21>)  [unwired: 11 in, 2 out]
          }
        }
        n365 = call <vilib>:"DAQmx Stop Task.vi"("task/channels in"=w1415) -> ("task out"=w1426:refnum<k21>)  [unwired: 13 in, 1 out]
        n366 = call <vilib>:"DAQmx Stop Task.vi"("task/channels in"=w1431) -> ("task out"=w1432:refnum<k21>)  [unwired: 13 in, 1 out]
        n367 = call <vilib>:"DAQmx Stop Task.vi"("task/channels in"=w1420) -> ("task out"=w1423:refnum<k21>)  [unwired: 13 in, 1 out]
        n368 = call <vilib>:"DAQmx Clear Task.vi"("task in"=w1426) -> ()  [unwired: 14 in, 1 out]
        n369 = call <vilib>:"DAQmx Clear Task.vi"("task in"=w1423) -> ()  [unwired: 14 in, 1 out]
        n370 = call <vilib>:"DAQmx Clear Task.vi"("task in"=w1432) -> ()  [unwired: 14 in, 1 out]
        n371 = case shown="False" w1439 {
          tunnel: [states."Chilling" states."auto imaging"] -> w1444
          frame False {
          }
          frame True {
          }
        }
      }
      frame "robotic arm" {
        # "reinitialize the parameter;\nwait for the next tube."
        n372 = Increment(x=w1545) -> (x+1=w1524:i32)
        "loading tube#" <- w1524
        n373 = local read "tb Pulses to move"() -> (w1531:u32)
        n374 = local read "tube changing #"() -> (w1530:i32)
        n375 = Multiply(x=w1531, y=w1530) -> (x*y=w1529:u32)
        n376 = stacked-sequence {
          tunnel: w1529 -> [_ w1801]
          tunnel: "\r\n" -> [w1791 w1799]
          tunnel: [_ w1800] -> _
          tunnel: [_ w1799] -> _
          frame #0 {
            w1794 = u8 2 items=["0", "1", "2", "3", "4"] ("Axis Number")
            n377 = call "RS232C_SetSpeed.vi"("Low Speed"=u32 100, "High Speed"=u32 2000, "Acceleration Time"=u16 100, "Axis Number"=w1794, "Delimiter"=w1791, "Axis Count"=u8 2, "Range"=TRUE, "Main/Sub"=FALSE) -> ()  [unwired: 1 in, 2 out]
          }
          frame #1 {
            w1802 = u8 1 items=["0", "1", "2", "3", "4"] ("Axis Number")
            n378 = local read "tube Direction"() -> (w1798:bool)
            n379 = Not(x=w1798) -> (.not. x?=w1797:bool)
            n380 = call "RS232C_Move.vi"("Axis Count"=u8 2, "Axis Number"=w1802, "Pulse Number"=w1801, "Direction"=w1797, "Delimiter"=w1799) -> ("OK Done"=w1800:bool)  [unwired: 2 in, 1 out]
          }
        }
        n381 = call-poly <vilib>:"DAQmx Create Virtual Channel.vi"("lines"=tag "Dev1/port1/line3") -> ("task out"=w1562:refnum<k21>, "error out"=w1561:errorcluster)  [unwired: 13 in]
        n382 = call <vilib>:"DAQmx Start Task.vi"("task/channels in"=w1562, "error in"=w1561) -> ("task out"=w1559:refnum<k21>, "error out"=w1557:errorcluster)  [unwired: 12 in]
        n383 = Greater?(x=w1524, y="tube to stop") -> (0:w1522:bool)
        n384 = call-poly <vilib>:"DAQmx Create Virtual Channel.vi"("lines"=tag "Dev1/port1/line0") -> ("task out"=w1572:refnum<k21>, "error out"=w1571:errorcluster)  [unwired: 13 in]
        n385 = local write "Larvae until move"(0 ("Larva # to move")) -> ()
        n386 = call <vilib>:"DAQmx Start Task.vi"("task/channels in"=w1572, "error in"=w1571) -> ("task out"=w1570:refnum<k21>, "error out"=w1569:errorcluster)  [unwired: 12 in]
        n387 = call-poly <vilib>:"DAQmx Create Virtual Channel.vi"("lines"=tag "Dev1/port1/line4") -> ("task out"=w1564:refnum<k21>, "error out"=w1563:errorcluster)  [unwired: 13 in]
        n388 = case shown="True" w1522 {
          tunnel: [w1785 states."Close"] -> w1546
          frame False {
            n389 = local read "Continuous\nacquisition"() -> (w1784:bool)
            n390 = case shown="True" w1784 {
              tunnel: [states."Chilling" states."auto imaging"] -> w1785
              frame False {
              }
              frame True {
              }
            }
          }
          frame True {
          }
        }
        n391 = call <vilib>:"DAQmx Start Task.vi"("task/channels in"=w1564, "error in"=w1563) -> ("task out"=w1560:refnum<k21>, "error out"=w1558:errorcluster)  [unwired: 12 in]
        n392 = stacked-sequence {
          seq-local: [w1599 _ _ _ _ _ _ _ _ _ _ _ _ _ _ _ _ _] -> [_ w1612 _ _ _ _ _ _ _ _ _ _ _ _ _ _ _ _]
          seq-local: [w1598 _ _ _ _ _ _ _ _ _ _ _ _ _ _ _ _ _] -> [_ w1611 _ _ _ _ _ _ _ _ _ _ _ _ _ _ _ _]
          seq-local: [w1597 _ _ _ _ _ _ _ _ _ _ _ _ _ _ _ _ _] -> [_ w1607 _ _ _ _ _ _ _ _ _ _ _ _ _ _ _ _]
          seq-local: [w1596 _ _ _ _ _ _ _ _ _ _ _ _ _ _ _ _ _] -> [_ w1606 _ _ _ _ _ _ _ _ _ _ _ _ _ _ _ _]
          seq-local: [w1595 _ _ _ _ _ _ _ _ _ _ _ _ _ _ _ _ _] -> [_ w1605 _ _ _ _ _ _ _ _ _ _ _ _ _ _ _ _]
          seq-local: [w1594 _ _ _ _ _ _ _ _ _ _ _ _ _ _ _ _ _] -> [_ w1604 _ _ _ _ _ _ _ _ _ _ _ _ _ _ _ _]
          seq-local: [w1592 _ _ _ _ _ _ _ _ _ _ _ _ _ _ _ _ _] -> [_ w1603 _ _ _ _ _ _ _ _ _ _ _ _ _ _ _ _]
          seq-local: [_ w1609 _ _ _ _ _ _ _ _ _ _ _ _ _ _ _ _] -> [_ _ w1620 _ _ _ _ _ _ _ _ _ _ _ _ _ _ _]
          seq-local: [_ w1608 _ _ _ _ _ _ _ _ _ _ _ _ _ _ _ _] -> [_ _ w1619 _ _ _ _ _ _ _ _ _ _ _ _ _ _ _]
          seq-local: [_ w1607 _ _ _ _ _ _ _ _ _ _ _ _ _ _ _ _] -> [_ _ w1618 _ _ _ _ _ _ _ _ _ _ _ _ _ _ _]
          seq-local: [_ w1606 _ _ _ _ _ _ _ _ _ _ _ _ _ _ _ _] -> [_ _ w1617 _ _ _ _ _ _ _ _ _ _ _ _ _ _ _]
          seq-local: [_ w1605 _ _ _ _ _ _ _ _ _ _ _ _ _ _ _ _] -> [_ _ w1616 _ _ _ _ _ _ _ _ _ _ _ _ _ _ _]
          seq-local: [_ w1604 _ _ _ _ _ _ _ _ _ _ _ _ _ _ _ _] -> [_ _ w1615 _ _ _ _ _ _ _ _ _ _ _ _ _ _ _]
          seq-local: [_ w1603 _ _ _ _ _ _ _ _ _ _ _ _ _ _ _ _] -> [_ _ w1614 _ _ _ _ _ _ _ _ _ _ _ _ _ _ _]
          seq-local: [_ _ w1620 _ _ _ _ _ _ _ _ _ _ _ _ _ _ _] -> [_ _ _ w1634 _ _ _ _ _ _ _ _ _ _ _ _ _ _]
          seq-local: [_ _ w1619 _ _ _ _ _ _ _ _ _ _ _ _ _ _ _] -> [_ _ _ w1633 _ _ _ _ _ _ _ _ _ _ _ _ _ _]
          seq-local: [_ _ w1618 _ _ _ _ _ _ _ _ _ _ _ _ _ _ _] -> [_ _ _ w1632 _ _ _ _ _ _ _ _ _ _ _ _ _ _]
          seq-local: [_ _ w1617 _ _ _ _ _ _ _ _ _ _ _ _ _ _ _] -> [_ _ _ w1630 _ _ _ _ _ _ _ _ _ _ _ _ _ _]
          seq-local: [_ _ w1616 _ _ _ _ _ _ _ _ _ _ _ _ _ _ _] -> [_ _ _ w1631 _ _ _ _ _ _ _ _ _ _ _ _ _ _]
          seq-local: [_ _ w1615 _ _ _ _ _ _ _ _ _ _ _ _ _ _ _] -> [_ _ _ w1629 _ _ _ _ _ _ _ _ _ _ _ _ _ _]
          seq-local: [_ _ w1614 _ _ _ _ _ _ _ _ _ _ _ _ _ _ _] -> [_ _ _ w1625 _ _ _ _ _ _ _ _ _ _ _ _ _ _]
          seq-local: [_ _ _ w1630 _ _ _ _ _ _ _ _ _ _ _ _ _ _] -> [_ _ _ _ w1645 _ _ _ _ _ _ _ _ _ _ _ _ _]
          seq-local: [_ _ _ w1629 _ _ _ _ _ _ _ _ _ _ _ _ _ _] -> [_ _ _ _ w1644 _ _ _ _ _ _ _ _ _ _ _ _ _]
          seq-local: [_ _ _ w1627 _ _ _ _ _ _ _ _ _ _ _ _ _ _] -> [_ _ _ _ w1643 _ _ _ _ _ _ _ _ _ _ _ _ _]
          seq-local: [_ _ _ w1626 _ _ _ _ _ _ _ _ _ _ _ _ _ _] -> [_ _ _ _ w1642 _ _ _ _ _ _ _ _ _ _ _ _ _]
          seq-local: [_ _ _ w1625 _ _ _ _ _ _ _ _ _ _ _ _ _ _] -> [_ _ _ _ w1641 _ _ _ _ _ _ _ _ _ _ _ _ _]
          seq-local: [_ _ _ w1624 _ _ _ _ _ _ _ _ _ _ _ _ _ _] -> [_ _ _ _ w1640 _ _ _ _ _ _ _ _ _ _ _ _ _]
          seq-local: [_ _ _ w1623 _ _ _ _ _ _ _ _ _ _ _ _ _ _] -> [_ _ _ _ w1638 _ _ _ _ _ _ _ _ _ _ _ _ _]
          seq-local: [_ _ _ _ w1645 _ _ _ _ _ _ _ _ _ _ _ _ _] -> [_ _ _ _ _ w1658 _ _ _ _ _ _ _ _ _ _ _ _]
          seq-local: [_ _ _ _ w1644 _ _ _ _ _ _ _ _ _ _ _ _ _] -> [_ _ _ _ _ w1657 _ _ _ _ _ _ _ _ _ _ _ _]
          seq-local: [_ _ _ _ w1643 _ _ _ _ _ _ _ _ _ _ _ _ _] -> [_ _ _ _ _ w1647 _ _ _ _ _ _ _ _ _ _ _ _]
          seq-local: [_ _ _ _ w1642 _ _ _ _ _ _ _ _ _ _ _ _ _] -> [_ _ _ _ _ w1653 _ _ _ _ _ _ _ _ _ _ _ _]
          seq-local: [_ _ _ _ w1641 _ _ _ _ _ _ _ _ _ _ _ _ _] -> [_ _ _ _ _ w1652 _ _ _ _ _ _ _ _ _ _ _ _]
          seq-local: [_ _ _ _ w1639 _ _ _ _ _ _ _ _ _ _ _ _ _] -> [_ _ _ _ _ w1649 _ _ _ _ _ _ _ _ _ _ _ _]
          seq-local: [_ _ _ _ w1637 _ _ _ _ _ _ _ _ _ _ _ _ _] -> [_ _ _ _ _ w1648 _ _ _ _ _ _ _ _ _ _ _ _]
          seq-local: [_ _ _ _ _ w1649 _ _ _ _ _ _ _ _ _ _ _ _] -> [_ _ _ _ _ _ w1667 _ _ _ _ _ _ _ _ _ _ _]
          seq-local: [_ _ _ _ _ w1648 _ _ _ _ _ _ _ _ _ _ _ _] -> [_ _ _ _ _ _ w1666 _ _ _ _ _ _ _ _ _ _ _]
          seq-local: [_ _ _ _ _ w1647 _ _ _ _ _ _ _ _ _ _ _ _] -> [_ _ _ _ _ _ w1661 _ _ _ _ _ _ _ _ _ _ _]
          seq-local: [_ _ _ _ _ w1656 _ _ _ _ _ _ _ _ _ _ _ _] -> [_ _ _ _ _ _ w1665 _ _ _ _ _ _ _ _ _ _ _]
          seq-local: [_ _ _ _ _ w1653 _ _ _ _ _ _ _ _ _ _ _ _] -> [_ _ _ _ _ _ w1664 _ _ _ _ _ _ _ _ _ _ _]
          seq-local: [_ _ _ _ _ w1655 _ _ _ _ _ _ _ _ _ _ _ _] -> [_ _ _ _ _ _ w1663 _ _ _ _ _ _ _ _ _ _ _]
          seq-local: [_ _ _ _ _ w1651 _ _ _ _ _ _ _ _ _ _ _ _] -> [_ _ _ _ _ _ w1662 _ _ _ _ _ _ _ _ _ _ _]
          seq-local: [_ _ _ _ _ _ w1667 _ _ _ _ _ _ _ _ _ _ _] -> [_ _ _ _ _ _ _ w1673 _ _ _ _ _ _ _ _ _ _]
          seq-local: [_ _ _ _ _ _ w1666 _ _ _ _ _ _ _ _ _ _ _] -> [_ _ _ _ _ _ _ w1672 _ _ _ _ _ _ _ _ _ _]
          seq-local: [_ _ _ _ _ _ w1660 _ _ _ _ _ _ _ _ _ _ _] -> [_ _ _ _ _ _ _ w1677 _ _ _ _ _ _ _ _ _ _]
          seq-local: [_ _ _ _ _ _ w1665 _ _ _ _ _ _ _ _ _ _ _] -> [_ _ _ _ _ _ _ w1676 _ _ _ _ _ _ _ _ _ _]
          seq-local: [_ _ _ _ _ _ w1664 _ _ _ _ _ _ _ _ _ _ _] -> [_ _ _ _ _ _ _ w1675 _ _ _ _ _ _ _ _ _ _]
          seq-local: [_ _ _ _ _ _ w1663 _ _ _ _ _ _ _ _ _ _ _] -> [_ _ _ _ _ _ _ w1674 _ _ _ _ _ _ _ _ _ _]
          seq-local: [_ _ _ _ _ _ w1662 _ _ _ _ _ _ _ _ _ _ _] -> [_ _ _ _ _ _ _ w1668 _ _ _ _ _ _ _ _ _ _]
          seq-local: [_ _ _ _ _ _ _ w1677 _ _ _ _ _ _ _ _ _ _] -> [_ _ _ _ _ _ _ _ w1688 _ _ _ _ _ _ _ _ _]
          seq-local: [_ _ _ _ _ _ _ w1676 _ _ _ _ _ _ _ _ _ _] -> [_ _ _ _ _ _ _ _ w1686 _ _ _ _ _ _ _ _ _]
          seq-local: [_ _ _ _ _ _ _ w1675 _ _ _ _ _ _ _ _ _ _] -> [_ _ _ _ _ _ _ _ w1687 _ _ _ _ _ _ _ _ _]
          seq-local: [_ _ _ _ _ _ _ w1674 _ _ _ _ _ _ _ _ _ _] -> [_ _ _ _ _ _ _ _ w1685 _ _ _ _ _ _ _ _ _]
          seq-local: [_ _ _ _ _ _ _ w1671 _ _ _ _ _ _ _ _ _ _] -> [_ _ _ _ _ _ _ _ w1690 _ _ _ _ _ _ _ _ _]
          seq-local: [_ _ _ _ _ _ _ w1670 _ _ _ _ _ _ _ _ _ _] -> [_ _ _ _ _ _ _ _ w1689 _ _ _ _ _ _ _ _ _]
          seq-local: [_ _ _ _ _ _ _ w1668 _ _ _ _ _ _ _ _ _ _] -> [_ _ _ _ _ _ _ _ w1681 _ _ _ _ _ _ _ _ _]
          seq-local: [_ _ _ _ _ _ _ _ w1690 _ _ _ _ _ _ _ _ _] -> [_ _ _ _ _ _ _ _ _ w1700 _ _ _ _ _ _ _ _]
          seq-local: [_ _ _ _ _ _ _ _ w1689 _ _ _ _ _ _ _ _ _] -> [_ _ _ _ _ _ _ _ _ w1699 _ _ _ _ _ _ _ _]
          seq-local: [_ _ _ _ _ _ _ _ w1688 _ _ _ _ _ _ _ _ _] -> [_ _ _ _ _ _ _ _ _ w1698 _ _ _ _ _ _ _ _]
          seq-local: [_ _ _ _ _ _ _ _ w1687 _ _ _ _ _ _ _ _ _] -> [_ _ _ _ _ _ _ _ _ w1697 _ _ _ _ _ _ _ _]
          seq-local: [_ _ _ _ _ _ _ _ w1684 _ _ _ _ _ _ _ _ _] -> [_ _ _ _ _ _ _ _ _ w1694 _ _ _ _ _ _ _ _]
          seq-local: [_ _ _ _ _ _ _ _ w1683 _ _ _ _ _ _ _ _ _] -> [_ _ _ _ _ _ _ _ _ w1696 _ _ _ _ _ _ _ _]
          seq-local: [_ _ _ _ _ _ _ _ w1679 _ _ _ _ _ _ _ _ _] -> [_ _ _ _ _ _ _ _ _ w1695 _ _ _ _ _ _ _ _]
          seq-local: [_ _ _ _ _ _ _ _ _ w1700 _ _ _ _ _ _ _ _] -> [_ _ _ _ _ _ _ _ _ _ w1710 _ _ _ _ _ _ _]
          seq-local: [_ _ _ _ _ _ _ _ _ w1699 _ _ _ _ _ _ _ _] -> [_ _ _ _ _ _ _ _ _ _ w1709 _ _ _ _ _ _ _]
          seq-local: [_ _ _ _ _ _ _ _ _ w1698 _ _ _ _ _ _ _ _] -> [_ _ _ _ _ _ _ _ _ _ w1708 _ _ _ _ _ _ _]
          seq-local: [_ _ _ _ _ _ _ _ _ w1697 _ _ _ _ _ _ _ _] -> [_ _ _ _ _ _ _ _ _ _ w1707 _ _ _ _ _ _ _]
          seq-local: [_ _ _ _ _ _ _ _ _ w1693 _ _ _ _ _ _ _ _] -> [_ _ _ _ _ _ _ _ _ _ w1703 _ _ _ _ _ _ _]
          seq-local: [_ _ _ _ _ _ _ _ _ w1696 _ _ _ _ _ _ _ _] -> [_ _ _ _ _ _ _ _ _ _ w1706 _ _ _ _ _ _ _]
          seq-local: [_ _ _ _ _ _ _ _ _ w1695 _ _ _ _ _ _ _ _] -> [_ _ _ _ _ _ _ _ _ _ w1705 _ _ _ _ _ _ _]
          seq-local: [_ _ _ _ _ _ _ _ _ _ w1710 _ _ _ _ _ _ _] -> [_ _ _ _ _ _ _ _ _ _ _ w1720 _ _ _ _ _ _]
          seq-local: [_ _ _ _ _ _ _ _ _ _ w1709 _ _ _ _ _ _ _] -> [_ _ _ _ _ _ _ _ _ _ _ w1719 _ _ _ _ _ _]
          seq-local: [_ _ _ _ _ _ _ _ _ _ w1708 _ _ _ _ _ _ _] -> [_ _ _ _ _ _ _ _ _ _ _ w1718 _ _ _ _ _ _]
          seq-local: [_ _ _ _ _ _ _ _ _ _ w1707 _ _ _ _ _ _ _] -> [_ _ _ _ _ _ _ _ _ _ _ w1717 _ _ _ _ _ _]
          seq-local: [_ _ _ _ _ _ _ _ _ _ w1702 _ _ _ _ _ _ _] -> [_ _ _ _ _ _ _ _ _ _ _ w1714 _ _ _ _ _ _]
          seq-local: [_ _ _ _ _ _ _ _ _ _ w1706 _ _ _ _ _ _ _] -> [_ _ _ _ _ _ _ _ _ _ _ w1716 _ _ _ _ _ _]
          seq-local: [_ _ _ _ _ _ _ _ _ _ w1705 _ _ _ _ _ _ _] -> [_ _ _ _ _ _ _ _ _ _ _ w1715 _ _ _ _ _ _]
          seq-local: [_ _ _ _ _ _ _ _ _ _ _ w1720 _ _ _ _ _ _] -> [_ _ _ _ _ _ _ _ _ _ _ _ w1730 _ _ _ _ _]
          seq-local: [_ _ _ _ _ _ _ _ _ _ _ w1719 _ _ _ _ _ _] -> [_ _ _ _ _ _ _ _ _ _ _ _ w1729 _ _ _ _ _]
          seq-local: [_ _ _ _ _ _ _ _ _ _ _ w1718 _ _ _ _ _ _] -> [_ _ _ _ _ _ _ _ _ _ _ _ w1728 _ _ _ _ _]
          seq-local: [_ _ _ _ _ _ _ _ _ _ _ w1717 _ _ _ _ _ _] -> [_ _ _ _ _ _ _ _ _ _ _ _ w1727 _ _ _ _ _]
          seq-local: [_ _ _ _ _ _ _ _ _ _ _ w1713 _ _ _ _ _ _] -> [_ _ _ _ _ _ _ _ _ _ _ _ w1724 _ _ _ _ _]
          seq-local: [_ _ _ _ _ _ _ _ _ _ _ w1716 _ _ _ _ _ _] -> [_ _ _ _ _ _ _ _ _ _ _ _ w1726 _ _ _ _ _]
          seq-local: [_ _ _ _ _ _ _ _ _ _ _ w1715 _ _ _ _ _ _] -> [_ _ _ _ _ _ _ _ _ _ _ _ w1725 _ _ _ _ _]
          seq-local: [_ _ _ _ _ _ _ _ _ _ _ _ w1730 _ _ _ _ _] -> [_ _ _ _ _ _ _ _ _ _ _ _ _ w1740 _ _ _ _]
          seq-local: [_ _ _ _ _ _ _ _ _ _ _ _ w1729 _ _ _ _ _] -> [_ _ _ _ _ _ _ _ _ _ _ _ _ w1739 _ _ _ _]
          seq-local: [_ _ _ _ _ _ _ _ _ _ _ _ w1728 _ _ _ _ _] -> [_ _ _ _ _ _ _ _ _ _ _ _ _ w1738 _ _ _ _]
          seq-local: [_ _ _ _ _ _ _ _ _ _ _ _ w1727 _ _ _ _ _] -> [_ _ _ _ _ _ _ _ _ _ _ _ _ w1737 _ _ _ _]
          seq-local: [_ _ _ _ _ _ _ _ _ _ _ _ w1726 _ _ _ _ _] -> [_ _ _ _ _ _ _ _ _ _ _ _ _ w1736 _ _ _ _]
          seq-local: [_ _ _ _ _ _ _ _ _ _ _ _ w1725 _ _ _ _ _] -> [_ _ _ _ _ _ _ _ _ _ _ _ _ w1735 _ _ _ _]
          seq-local: [_ _ _ _ _ _ _ _ _ _ _ _ w1723 _ _ _ _ _] -> [_ _ _ _ _ _ _ _ _ _ _ _ _ w1734 _ _ _ _]
          seq-local: [_ _ _ _ _ _ _ _ _ _ _ _ _ w1740 _ _ _ _] -> [_ _ _ _ _ _ _ _ _ _ _ _ _ _ w1750 _ _ _]
          seq-local: [_ _ _ _ _ _ _ _ _ _ _ _ _ w1739 _ _ _ _] -> [_ _ _ _ _ _ _ _ _ _ _ _ _ _ w1749 _ _ _]
          seq-local: [_ _ _ _ _ _ _ _ _ _ _ _ _ w1738 _ _ _ _] -> [_ _ _ _ _ _ _ _ _ _ _ _ _ _ w1748 _ _ _]
          seq-local: [_ _ _ _ _ _ _ _ _ _ _ _ _ w1737 _ _ _ _] -> [_ _ _ _ _ _ _ _ _ _ _ _ _ _ w1747 _ _ _]
          seq-local: [_ _ _ _ _ _ _ _ _ _ _ _ _ w1736 _ _ _ _] -> [_ _ _ _ _ _ _ _ _ _ _ _ _ _ w1746 _ _ _]
          seq-local: [_ _ _ _ _ _ _ _ _ _ _ _ _ w1735 _ _ _ _] -> [_ _ _ _ _ _ _ _ _ _ _ _ _ _ w1745 _ _ _]
          seq-local: [_ _ _ _ _ _ _ _ _ _ _ _ _ w1733 _ _ _ _] -> [_ _ _ _ _ _ _ _ _ _ _ _ _ _ w1744 _ _ _]
          seq-local: [_ _ _ _ _ _ _ _ _ _ _ _ _ _ w1750 _ _ _] -> [_ _ _ _ _ _ _ _ _ _ _ _ _ _ _ w1760 _ _]
          seq-local: [_ _ _ _ _ _ _ _ _ _ _ _ _ _ w1749 _ _ _] -> [_ _ _ _ _ _ _ _ _ _ _ _ _ _ _ w1759 _ _]
          seq-local: [_ _ _ _ _ _ _ _ _ _ _ _ _ _ w1748 _ _ _] -> [_ _ _ _ _ _ _ _ _ _ _ _ _ _ _ w1758 _ _]
          seq-local: [_ _ _ _ _ _ _ _ _ _ _ _ _ _ w1747 _ _ _] -> [_ _ _ _ _ _ _ _ _ _ _ _ _ _ _ w1757 _ _]
          seq-local: [_ _ _ _ _ _ _ _ _ _ _ _ _ _ w1746 _ _ _] -> [_ _ _ _ _ _ _ _ _ _ _ _ _ _ _ w1756 _ _]
          seq-local: [_ _ _ _ _ _ _ _ _ _ _ _ _ _ w1745 _ _ _] -> [_ _ _ _ _ _ _ _ _ _ _ _ _ _ _ w1755 _ _]
          seq-local: [_ _ _ _ _ _ _ _ _ _ _ _ _ _ w1743 _ _ _] -> [_ _ _ _ _ _ _ _ _ _ _ _ _ _ _ w1751 _ _]
          seq-local: [_ _ _ _ _ _ _ _ _ _ _ _ _ _ _ w1760 _ _] -> [_ _ _ _ _ _ _ _ _ _ _ _ _ _ _ _ w1771 _]
          seq-local: [_ _ _ _ _ _ _ _ _ _ _ _ _ _ _ w1759 _ _] -> [_ _ _ _ _ _ _ _ _ _ _ _ _ _ _ _ w1770 _]
          seq-local: [_ _ _ _ _ _ _ _ _ _ _ _ _ _ _ w1758 _ _] -> [_ _ _ _ _ _ _ _ _ _ _ _ _ _ _ _ w1769 _]
          seq-local: [_ _ _ _ _ _ _ _ _ _ _ _ _ _ _ w1757 _ _] -> [_ _ _ _ _ _ _ _ _ _ _ _ _ _ _ _ w1768 _]
          seq-local: [_ _ _ _ _ _ _ _ _ _ _ _ _ _ _ w1754 _ _] -> [_ _ _ _ _ _ _ _ _ _ _ _ _ _ _ _ w1766 _]
          seq-local: [_ _ _ _ _ _ _ _ _ _ _ _ _ _ _ w1756 _ _] -> [_ _ _ _ _ _ _ _ _ _ _ _ _ _ _ _ w1767 _]
          seq-local: [_ _ _ _ _ _ _ _ _ _ _ _ _ _ _ w1755 _ _] -> [_ _ _ _ _ _ _ _ _ _ _ _ _ _ _ _ w1762 _]
          seq-local: [_ _ _ _ _ _ _ _ _ _ _ _ _ _ _ _ w1771 _] -> [_ _ _ _ _ _ _ _ _ _ _ _ _ _ _ _ _ w1783]
          seq-local: [_ _ _ _ _ _ _ _ _ _ _ _ _ _ _ _ w1770 _] -> [_ _ _ _ _ _ _ _ _ _ _ _ _ _ _ _ _ w1782]
          seq-local: [_ _ _ _ _ _ _ _ _ _ _ _ _ _ _ _ w1769 _] -> [_ _ _ _ _ _ _ _ _ _ _ _ _ _ _ _ _ w1781]
          seq-local: [_ _ _ _ _ _ _ _ _ _ _ _ _ _ _ _ w1768 _] -> [_ _ _ _ _ _ _ _ _ _ _ _ _ _ _ _ _ w1780]
          seq-local: [_ _ _ _ _ _ _ _ _ _ _ _ _ _ _ _ w1765 _] -> [_ _ _ _ _ _ _ _ _ _ _ _ _ _ _ _ _ w1779]
          seq-local: [_ _ _ _ _ _ _ _ _ _ _ _ _ _ _ _ w1767 _] -> [_ _ _ _ _ _ _ _ _ _ _ _ _ _ _ _ _ w1778]
          seq-local: [_ _ _ _ _ _ _ _ _ _ _ _ _ _ _ _ w1762 _] -> [_ _ _ _ _ _ _ _ _ _ _ _ _ _ _ _ _ w1774]
          tunnel: w1570 -> [w1602 _ _ _ _ _ _ _ _ _ _ _ _ _ _ _ _ _]
          tunnel: w1569 -> [w1601 _ _ _ _ _ _ _ _ _ _ _ _ _ _ _ _ _]
          tunnel: w1560 -> [w1597 _ _ _ _ _ _ _ _ _ _ _ _ _ _ _ _ _]
          tunnel: w1559 -> [w1596 _ _ _ _ _ _ _ _ _ _ _ _ _ _ _ _ _]
          tunnel: w1558 -> [w1595 _ _ _ _ _ _ _ _ _ _ _ _ _ _ _ _ _]
          tunnel: w1557 -> [w1594 _ _ _ _ _ _ _ _ _ _ _ _ _ _ _ _ _]
          tunnel: w1537 -> [w1592 _ _ _ _ _ _ _ _ _ _ _ _ _ _ _ _ _]
          tunnel: [_ _ _ _ _ _ _ _ _ _ _ _ _ _ _ _ _ w1783] -> w1566
          tunnel: [_ _ _ _ _ _ _ _ _ _ _ _ _ _ _ _ _ w1782] -> w1565
          tunnel: [_ _ _ _ _ _ _ _ _ _ _ _ _ _ _ _ _ w1781] -> w1554
          tunnel: [_ _ _ _ _ _ _ _ _ _ _ _ _ _ _ _ _ w1780] -> w1553
          tunnel: [_ _ _ _ _ _ _ _ _ _ _ _ _ _ _ _ _ w1777] -> w1550
          tunnel: [_ _ _ _ _ _ _ _ _ _ _ _ _ _ _ _ _ w1776] -> w1549
          tunnel: [_ _ _ _ _ _ _ _ _ _ _ _ _ _ _ _ _ w1773] -> w1536
          frame #0 {
            n393 = call-poly <vilib>:"DAQmx Write.vi"("task/channels in"=w1602, "data"=TRUE, "error in"=w1601) -> ("task out"=w1599:refnum<k21>, "error out"=w1598:errorcluster)  [unwired: 10 in, 1 out]
            n394 = Wait (ms)(milliseconds to wait=u32 1000) -> ()  [unwired: 1 out]
          }
          frame #1 {
            n395 = call-poly <vilib>:"DAQmx Write.vi"("task/channels in"=w1612, "data"=FALSE, "error in"=w1611) -> ("task out"=w1609:refnum<k21>, "error out"=w1608:errorcluster)  [unwired: 10 in, 1 out]
          }
          frame #2 {
            n396 = Wait (ms)(milliseconds to wait="waiting time for\n robotic arm") -> ()  [unwired: 1 out]
          }
          frame #3 {
            n397 = call-poly <vilib>:"DAQmx Write.vi"("task/channels in"=w1632, "data"=TRUE, "error in"=w1631) -> ("task out"=w1627:refnum<k21>, "error out"=w1626:errorcluster)  [unwired: 10 in, 1 out]
            n398 = Wait (ms)(milliseconds to wait=u32 2000 ("milliseconds to wait 4")) -> ()  [unwired: 1 out]
            n399 = call-poly <vilib>:"DAQmx Write.vi"("task/channels in"=w1634, "data"=TRUE, "error in"=w1633) -> ("task out"=w1624:refnum<k21>, "error out"=w1623:errorcluster)  [unwired: 10 in, 1 out]
          }
          frame #4 {
            n400 = call-poly <vilib>:"DAQmx Write.vi"("task/channels in"=w1640, "data"=FALSE, "error in"=w1638) -> ("task out"=w1639:refnum<k21>, "error out"=w1637:errorcluster)  [unwired: 10 in, 1 out]
            n401 = Wait (ms)(milliseconds to wait=u32 500) -> ()  [unwired: 1 out]
          }
          frame #5 {
            n402 = call-poly <vilib>:"DAQmx Write.vi"("task/channels in"=w1658, "data"=TRUE, "error in"=w1657) -> ("task out"=w1656:refnum<k21>, "error out"=w1655:errorcluster)  [unwired: 10 in, 1 out]
            n403 = Wait (ms)(milliseconds to wait="shower time") -> ()  [unwired: 1 out]
            n404 = call-poly <vilib>:"DAQmx Write.vi"("task/channels in"=w1652, "data"=TRUE) -> ("task out"=w1651:refnum<k21>)  [unwired: 11 in, 2 out]
          }
          frame #6 {
            n405 = call-poly <vilib>:"DAQmx Write.vi"("task/channels in"=w1661, "data"=FALSE) -> ("task out"=w1660:refnum<k21>)  [unwired: 11 in, 2 out]
          }
          frame #7 {
            n406 = call-poly <vilib>:"DAQmx Write.vi"("task/channels in"=w1673, "data"=FALSE, "error in"=w1672) -> ("task out"=w1671:refnum<k21>, "error out"=w1670:errorcluster)  [unwired: 10 in, 1 out]
          }
          frame #8 {
            n407 = call-poly <vilib>:"DAQmx Write.vi"("task/channels in"=w1686, "data"=TRUE, "error in"=w1685) -> ("task out"=w1684:refnum<k21>, "error out"=w1683:errorcluster)  [unwired: 10 in, 1 out]
            n408 = Wait (ms)(milliseconds to wait=u32 2000) -> ()  [unwired: 1 out]
            n409 = call-poly <vilib>:"DAQmx Write.vi"("task/channels in"=w1681, "data"=TRUE) -> ("task out"=w1679:refnum<k21>)  [unwired: 11 in, 2 out]
          }
          frame #9 {
            n410 = Wait (ms)(milliseconds to wait=u32 500) -> ()  [unwired: 1 out]
            n411 = call-poly <vilib>:"DAQmx Write.vi"("task/channels in"=w1694, "data"=FALSE) -> ("task out"=w1693:refnum<k21>)  [unwired: 11 in, 2 out]
          }
          frame #10 {
            n412 = call-poly <vilib>:"DAQmx Write.vi"("task/channels in"=w1703, "data"=TRUE) -> ("task out"=w1702:refnum<k21>)  [unwired: 11 in, 2 out]
            n413 = Wait (ms)(milliseconds to wait=u32 500) -> ()  [unwired: 1 out]
          }
          frame #11 {
            n414 = call-poly <vilib>:"DAQmx Write.vi"("task/channels in"=w1714, "data"=FALSE) -> ("task out"=w1713:refnum<k21>)  [unwired: 11 in, 2 out]
            n415 = Wait (ms)(milliseconds to wait=u32 500) -> ()  [unwired: 1 out]
          }
          frame #12 {
            n416 = call-poly <vilib>:"DAQmx Write.vi"("task/channels in"=w1724, "data"=TRUE) -> ("task out"=w1723:refnum<k21>)  [unwired: 11 in, 2 out]
            n417 = Wait (ms)(milliseconds to wait=u32 500) -> ()  [unwired: 1 out]
          }
          frame #13 {
            n418 = call-poly <vilib>:"DAQmx Write.vi"("task/channels in"=w1734, "data"=FALSE) -> ("task out"=w1733:refnum<k21>)  [unwired: 11 in, 2 out]
            n419 = Wait (ms)(milliseconds to wait=u32 500) -> ()  [unwired: 1 out]
          }
          frame #14 {
            n420 = call-poly <vilib>:"DAQmx Write.vi"("task/channels in"=w1744, "data"=TRUE) -> ("task out"=w1743:refnum<k21>)  [unwired: 11 in, 2 out]
            n421 = Wait (ms)(milliseconds to wait=u32 3000) -> ()  [unwired: 1 out]
          }
          frame #15 {
            n422 = call-poly <vilib>:"DAQmx Write.vi"("task/channels in"=w1751, "data"=FALSE) -> ("task out"=w1754:refnum<k21>)  [unwired: 11 in, 2 out]
            n423 = Wait (ms)(milliseconds to wait=u32 500) -> ()  [unwired: 1 out]
          }
          frame #16 {
            n424 = local write "tube changing #"(0 ("tube changing #")) -> ()
            n425 = call-poly <vilib>:"DAQmx Write.vi"("task/channels in"=w1766, "data"=TRUE) -> ("task out"=w1765:refnum<k21>)  [unwired: 11 in, 2 out]
            n426 = Wait (ms)(milliseconds to wait="washing time") -> ()  [unwired: 1 out]
          }
          frame #17 {
            n427 = call-poly <vilib>:"DAQmx Write.vi"("task/channels in"=w1779, "data"=FALSE, "error in"=w1778) -> ("task out"=w1777:refnum<k21>, "error out"=w1776:errorcluster)  [unwired: 10 in, 1 out]
            n428 = call-poly <vilib>:"DAQmx Write.vi"("task/channels in"=w1774, "data"=FALSE) -> ("task out"=w1773:refnum<k21>)  [unwired: 11 in, 2 out]
          }
        }
        n429 = call <vilib>:"DAQmx Stop Task.vi"("task/channels in"=w1550, "error in"=w1549) -> ("task out"=w1552:refnum<k21>, "error out"=w1551:errorcluster)  [unwired: 12 in]
        n430 = call <vilib>:"DAQmx Stop Task.vi"("task/channels in"=w1566, "error in"=w1565) -> ("task out"=w1568:refnum<k21>, "error out"=w1567:errorcluster)  [unwired: 12 in]
        n431 = call <vilib>:"DAQmx Stop Task.vi"("task/channels in"=w1554, "error in"=w1553) -> ("task out"=w1556:refnum<k21>, "error out"=w1555:errorcluster)  [unwired: 12 in]
        n432 = call <vilib>:"DAQmx Clear Task.vi"("task in"=w1552, "error in"=w1551) -> ()  [unwired: 13 in, 1 out]
        n433 = call <vilib>:"DAQmx Clear Task.vi"("task in"=w1568, "error in"=w1567) -> ()  [unwired: 13 in, 1 out]
        n434 = call <vilib>:"DAQmx Clear Task.vi"("task in"=w1556, "error in"=w1555) -> ()  [unwired: 13 in, 1 out]
      }
      frame "manual loading" {
        # "shower valves"
        n435 = flat-sequence {
          tunnel: w1845 -> [w1891]
          tunnel: w1844 -> [w1893]
          tunnel: w1843 -> [w1892]
          tunnel: [w1893] -> w1842
          tunnel: [w1892] -> w1841
          tunnel: [w1888] -> w1840
          tunnel: w1842 -> [w1901]
          tunnel: w1841 -> [w1900]
          tunnel: w1840 -> [w1896]
          tunnel: [w1896] -> w1839
          tunnel: [w1895] -> w1838
          tunnel: [w1894] -> w1833
          tunnel: w1839 -> [w1903]
          tunnel: w1838 -> [w1907]
          tunnel: [w1905] -> w1837
          tunnel: w1833 -> [w1904]
          tunnel: [w1904] -> w1829
          tunnel: [w1903] -> w1828
          tunnel: w1837 -> [w1915]
          tunnel: [w1914] -> w1836
          tunnel: [w1913] -> w1830
          tunnel: w1829 -> [w1913]
          tunnel: w1828 -> [w1912]
          tunnel: [w1909] -> w1819
          tunnel: w1836 -> [w1921]
          tunnel: [w1920] -> w1835
          tunnel: [w1919] -> w1831
          tunnel: w1830 -> [w1919]
          tunnel: w1819 -> [w1917]
          tunnel: [w1917] -> w1817
          tunnel: w1835 -> [w1927]
          tunnel: [w1926] -> w1834
          tunnel: [w1925] -> w1832
          tunnel: w1831 -> [w1925]
          tunnel: [w1923] -> w1818
          tunnel: w1817 -> [w1923]
          tunnel: w1834 -> [w1934]
          tunnel: w1832 -> [w1933]
          tunnel: [w1931] -> w1821
          tunnel: [w1930] -> w1820
          tunnel: [w1929] -> w1816
          tunnel: w1818 -> [w1929]
          frame #0 {
            n436 = call-poly <vilib>:"DAQmx Write.vi"("task/channels in"=w1891, "data"=TRUE) -> ("task out"=w1888:refnum<k21>)  [unwired: 11 in, 2 out]
            n437 = Wait (ms)(milliseconds to wait=u32 1000) -> ()  [unwired: 1 out]
          }
          frame #1 {
            n438 = call-poly <vilib>:"DAQmx Write.vi"("task/channels in"=w1901, "data"=TRUE) -> ("task out"=w1894:refnum<k21>)  [unwired: 11 in, 2 out]
            n439 = call-poly <vilib>:"DAQmx Write.vi"("task/channels in"=w1900, "data"=TRUE) -> ("task out"=w1895:refnum<k21>)  [unwired: 11 in, 2 out]
            n440 = Wait (ms)(milliseconds to wait="shower time(ms)") -> ()  [unwired: 1 out]
          }
          frame #2 {
            n441 = call-poly <vilib>:"DAQmx Write.vi"("task/channels in"=w1907, "data"=FALSE) -> ("task out"=w1905:refnum<k21>)  [unwired: 11 in, 2 out]
            n442 = Wait (ms)(milliseconds to wait=u32 500) -> ()  [unwired: 1 out]
          }
          frame #3 {
            n443 = call-poly <vilib>:"DAQmx Write.vi"("task/channels in"=w1915, "data"=TRUE ("auto start")) -> ("task out"=w1914:refnum<k21>)  [unwired: 11 in, 2 out]
            n444 = call-poly <vilib>:"DAQmx Write.vi"("task/channels in"=w1912, "data"=FALSE) -> ("task out"=w1909:refnum<k21>)  [unwired: 11 in, 2 out]
            n445 = Wait (ms)(milliseconds to wait=u32 500) -> ()  [unwired: 1 out]
          }
          frame #4 {
            n446 = call-poly <vilib>:"DAQmx Write.vi"("task/channels in"=w1921, "data"=FALSE ("auto start")) -> ("task out"=w1920:refnum<k21>)  [unwired: 11 in, 2 out]
            n447 = Wait (ms)(milliseconds to wait=u32 500) -> ()  [unwired: 1 out]
          }
          frame #5 {
            n448 = call-poly <vilib>:"DAQmx Write.vi"("task/channels in"=w1927, "data"=TRUE ("auto start")) -> ("task out"=w1926:refnum<k21>)  [unwired: 11 in, 2 out]
            n449 = Wait (ms)(milliseconds to wait=u32 2000) -> ()  [unwired: 1 out]
          }
          frame #6 {
            n450 = call-poly <vilib>:"DAQmx Write.vi"("task/channels in"=w1934, "data"=FALSE ("auto start")) -> ("task out"=w1931:refnum<k21>)  [unwired: 11 in, 2 out]
            n451 = call-poly <vilib>:"DAQmx Write.vi"("task/channels in"=w1933, "data"=FALSE) -> ("task out"=w1930:refnum<k21>)  [unwired: 11 in, 2 out]
          }
        }
        n452 = call-poly <vilib>:"DAQmx Create Virtual Channel.vi"("lines"=tag "Dev1/port1/line2") -> ("task out"=w1851:refnum<k21>, "error out"=w1850:errorcluster)  [unwired: 13 in]
        n453 = call-poly <vilib>:"DAQmx Create Virtual Channel.vi"("lines"=tag "Dev1/port1/line3") -> ("task out"=w1849:refnum<k21>, "error out"=w1848:errorcluster)  [unwired: 13 in]
        n454 = call <vilib>:"DAQmx Start Task.vi"("task/channels in"=w1851, "error in"=w1850) -> ("task out"=w1844:refnum<k21>)  [unwired: 12 in, 1 out]
        n455 = call-poly <vilib>:"DAQmx Create Virtual Channel.vi"("lines"=tag "Dev1/port1/line4") -> ("task out"=w1847:refnum<k21>, "error out"=w1846:errorcluster)  [unwired: 13 in]
        n456 = call <vilib>:"DAQmx Start Task.vi"("task/channels in"=w1849, "error in"=w1848) -> ("task out"=w1843:refnum<k21>)  [unwired: 12 in, 1 out]
        n457 = call <vilib>:"DAQmx Start Task.vi"("task/channels in"=w1847, "error in"=w1846) -> ("task out"=w1845:refnum<k21>)  [unwired: 12 in, 1 out]
        n458 = local read "Continuous\nacquisition"() -> (w1815:bool)
        n459 = case shown="True" w1815 {
          tunnel: [states."Chilling" states."auto imaging"] -> w1814
          frame False {
          }
          frame True {
          }
        }
        n460 = call <vilib>:"DAQmx Stop Task.vi"("task/channels in"=w1821) -> ("task out"=w1827:refnum<k21>, "error out"=w1826:errorcluster)  [unwired: 13 in]
        n461 = call <vilib>:"DAQmx Stop Task.vi"("task/channels in"=w1816) -> ("task out"=w1823:refnum<k21>, "error out"=w1822:errorcluster)  [unwired: 13 in]
        n462 = call <vilib>:"DAQmx Stop Task.vi"("task/channels in"=w1820) -> ("task out"=w1825:refnum<k21>, "error out"=w1824:errorcluster)  [unwired: 13 in]
        n463 = call <vilib>:"DAQmx Clear Task.vi"("task in"=w1823, "error in"=w1822) -> ()  [unwired: 13 in, 1 out]
        n464 = call <vilib>:"DAQmx Clear Task.vi"("task in"=w1827, "error in"=w1826) -> ()  [unwired: 13 in, 1 out]
        n465 = call <vilib>:"DAQmx Clear Task.vi"("task in"=w1825, "error in"=w1824) -> ()  [unwired: 13 in, 1 out]
      }
      frame "Edgehunting" {
        w1943 = 0
        w1950 = 0 items=["DEFAULT", "NO BUFFERING"] ("Buffering Mode")
        w1966 = u32 2049184 items=["SENSOR MODE"=4212128, "SENSOR MODE LINE BUNDLE HEIGHT"=4212192, "READOUT DIRECTION"=4211904, "BIT PER CHANNEL"=4342976, "EXPOSURE TIME"=2049184, "CONTRAST GAIN"=3163312, "BINNING"=4215968, "TIMING READOUT TIME"=4223904, "INTERNAL FRAME RATE"=4225952, "INTERNAL FRAME INTERVAL"=4225968, "INTERNAL LINE SPEED"=4226000, "IMAGE WIDTH"=4343200, "IMAGE HEIGHT"=4343216, "IMAGE ROWBYTES"=4343232, "IMAGE FRAMEBYTES"=4343248, "IMAGE PIXEL TYPE"=4343296] ("Parameter")
        w1971 = u32 2049184 items=["SENSOR MODE"=4212128, "SENSOR MODE LINE BUNDLE HEIGHT"=4212192, "READOUT DIRECTION"=4211904, "BIT PER CHANNEL"=4342976, "EXPOSURE TIME"=2049184, "CONTRAST GAIN"=3163312, "BINNING"=4215968, "TIMING READOUT TIME"=4223904, "INTERNAL FRAME RATE"=4225952, "INTERNAL FRAME INTERVAL"=4225968, "INTERNAL LINE SPEED"=4226000, "IMAGE WIDTH"=4343200, "IMAGE HEIGHT"=4343216, "IMAGE ROWBYTES"=4343232, "IMAGE FRAMEBYTES"=4343248, "IMAGE PIXEL TYPE"=4343296] ("Parameter")
        w1946 = 0 ("element")
        w2012 = 120 ("dimension size")
        # "We manually set the exposure time for edge hunting to force 20 fps,\nfor this step only."
        n466 = call-poly <vilib>:"DAQmx Write.vi"("task/channels in"=w1948, "data"=FALSE) -> ()  [unwired: 11 in, 3 out]
        n467 = while "stage Loop" {
          tunnel: w2031 -> [w2095]
          tunnel: [w2092] -> w1986
          tunnel: ["scanning distance (um)"] -> _
          tunnel: ["Edge-hunting Direction"] -> _
          tunnel: [w2088] -> w2017
          tunnel: [w2087] -> w2020
          stop <- w2090 stop-if-true
          n468 = stacked-sequence {
            tunnel: w2095 -> [w2097 w2106 _]
            tunnel: "Main/Sub" -> [w2098 w2112 _]
            tunnel: "scanning distance (um)" -> [_ w2109 _]
            tunnel: "Edge-hunting Direction" -> [_ w2108 _]
            tunnel: "\r\n" -> [w2096 w2107 _]
            tunnel: [_ _ TRUE] -> w2090
            tunnel: [_ w2106 _] -> w2088
            tunnel: [_ w2107 _] -> w2087
            frame #0 {
              w2101 = u8 2 items=["0", "1", "2", "3", "4"] ("Axis Number")
              n469 = call "RS232C_SetSpeed.vi"("Low Speed"=u32 100, "High Speed"="High Speed 2", "Acceleration Time"=u16 100, "Axis Number"=w2101, "Delimiter"=w2096, "VISAリソース名"=w2097, "Axis Count"=u8 2, "Range"=TRUE, "Main/Sub"=w2098) -> ()  [unwired: 2 out]
              n470 = local write "OK Done"(FALSE ("OK Done")) -> ()
            }
            frame #1 {
              w2110 = u8 2 items=["0", "1", "2", "3", "4"] ("Axis Number")
              n471 = call "RS232C_Move.vi"("VISAリソース名"=w2106, "Axis Count"=u8 2, "Axis Number"=w2110, "Pulse Number"=w2109, "Direction"=w2108, "Delimiter"=w2107, "Main/Sub"=w2112) -> ()  [unwired: 2 out]
            }
            frame #2 {
            }
          }
          n472 = call <extravilib>:"Write.vi"("element"=w2090) -> ("channel"=w2092:T13)  [unwired: 1 out]
        }
        n473 = call "name.vi"("Save directory"=w1935, "tempro number"=w1938) -> ("temprory data name"=w1937:string)  [unwired: 7 in, 2 out]
        n474 = call <userlib>:"tm_setparameter_40.vi"("error in (no error)"=w1973, "Value in"=0.01953125, "Parameter"=w1971, "Handle in"=w1974) -> ("error out"=w1972:errorcluster, "Handle out"=w1952:u32)  [unwired: 6 in]
        n475 = Initialize Array(w1943, w1943, w1943) -> (w1944:i32[][])
        n476 = Bundle(w1944, w1943) -> (w1942:cluster{i32[][], i32})  [unwired: 1 in]
        n477 = Obtain Queue(name (unnamed)="stream", element data type=w1942) -> (queue out=w1941:refnum<queue>)  [unwired: 3 in, 2 out]
        n478 = Initialize Array(w1946, w1946) -> (w1985:i32[])
        n479 = Increment(x=w2003) -> (x+1=w2002:i32)
        n480 = while {
          shift-right: [w2080] -> _
          shift-left: w1941 -> [w2081]
          tunnel: w1986 -> [w2079]
          shift-right: [w2070] -> _
          shift-left: w1985 -> [w2071]
          stop <- w2078 stop-if-true
          n481 = call <extravilib>:"Read.vi"("channel"=w2079) -> ("element"=w2078:bool)  [unwired: 1 in, 1 out]
          n482 = Dequeue Element(queue=w2081) -> (queue out=w2080:refnum<queue>, element=w2077:cluster{i32[][], i32})  [unwired: 2 in, 2 out]
          n483 = Unbundle(w2077) -> (w2076:i32[][], w2072:i32)
          n484 = Array Max & Min(array=w2076) -> (max value=w2075:i32)  [unwired: 3 out]
          "max value" <- w2075
          n485 = Greater Or Equal?(x=w2075, y=300) -> (x >= y?=w2073:bool)
          n486 = case shown="True" w2073 {
            tunnel: w2072 -> [_ w2085]
            tunnel: w2071 -> [w2082 w2086]
            tunnel: [w2082 w2083] -> w2070
            frame False {
            }
            frame True {
              n487 = Insert Into Array(array=w2086, index=w2085, new element=1 ("new element/subarray")) -> (w2083:i32[])
            }
          }
        }
        n488 = String To Path(string=w1937) -> (path=w1936:path)
        n489 = call <userlib>:"tm_startrecorder_40.vi"("Buffering Mode"=w1950, "frames"=120, "File"=w1936, "Handle in"=w1952) -> ("Handle out"=w1953:u32)  [unwired: 6 in, 1 out]
        n490 = call <userlib>:"tm_startcapture_40.vi"("error in (no error)"=w1972, "Handle in"=w1953) -> ("error out"=w2029:errorcluster, "Handle out"=w2030:u32)  [unwired: 8 in]
        n491 = Initialize Array(0.0 ("element"), 0 ("dimension size")) -> (w1964:dbl[])
        n492 = local read "Continuous\nacquisition"() -> (w2015:bool)
        n493 = call <vilib>:"High Resolution Relative Seconds.vi"() -> ("relative seconds"=w2007:dbl)
        n494 = Initialize Array(0.0 ("element"), w2012) -> (w2024:dbl[])
        n495 = while {
          tunnel: w2030 -> [w2142]
          tunnel: w2029 -> [w2141]
          tunnel: [w2133] -> w2028
          tunnel: [w2134] -> w2027
          tunnel: [w2122] -> w2022
          tunnel: w2026 -> [w2122]
          tunnel: [w2119] -> _
          tunnel: w1986 -> [w2131]
          shift-right: [w2128] -> w2023
          shift-left: w2024 -> [w2129]
          tunnel: [w2119] -> w2013
          shift-right: [w2123] -> w1963
          shift-left: w1964 -> [w2124]
          shift-right: [w2117] -> w1940
          shift-left: w1941 -> [w2118]
          stop <- w2132 stop-if-true
          (unwired) TRUE ("Keep/Replace Value (Replace)")
          n496 = call <extravilib>:"Read.vi"("channel"=w2131) -> ("element"=w2132:bool)  [unwired: 1 in, 1 out]
          n497 = call <userlib>:"tm_waitnextframe_40.vi"("error in (no error)"=w2141, "Handle in"=w2142) -> ("error out"=w2134:errorcluster, "Frame Count"=w2119:i32, "Frame Index"=w2116:i32, "Handle out"=w2133:u32)  [unwired: 6 in]
          n498 = local read "XS x px start"() -> (w2139:i32)
          n499 = local read "XS y length"() -> (w2136:i32)
          n500 = local read "XS y px start"() -> (w2140:i32)
          n501 = local read "XS x length"() -> (w2135:i32)
          n502 = Index Array(array=w2122, index=w2116) -> (element=w2121:T12)
          n503 = local write "Frame count"(w2119) -> ()
          n504 = Multiply(x=w2136, y=w2135) -> (x*y=w2126:i32)
          n505 = call "IMAQ ImageToArray"("Image"=w2121) -> ("Image Pixels (U16)"=w2120:u16[][])  [unwired: 3 in, 4 out]
          n506 = local write "Obtained image"(w2120) -> ()
          n507 = local read "Mean trigger"() -> (w2137:i32)
          n508 = Array Subset(array=w2120, index (row)=w2140, length (row)=w2136, index (col)=w2139, length (col)=w2135) -> (w2114:u16[][])
          n509 = Bundle(w2114, "Frame Index"=w2116) -> (w2115:cluster{u16[][], "Frame Index":i32})  [unwired: 1 in]
          n510 = Enqueue Element(queue=w2118, element=w2115) -> (queue out=w2117:refnum<queue>)  [unwired: 2 in, 2 out]
          n511 = local write "Sub image"(w2114) -> ()
          n512 = Bundle(w2114, "Frame Index"=w2116) -> ()  [unwired: 1 in, 1 out]
          n513 = Reshape Array(w2120, w2126) -> (w2138:u16[])
          n514 = call-poly <vilib>:"Mean.vi"("X"=w2138) -> ("mean"=w2130:dbl)  [unwired: 1 out]
          n515 = local write "Sub img mean"(w2130) -> ()
          n516 = Greater Or Equal?(x=w2130, y=w2137) -> (x >= y?=w2125:bool)
          n517 = case shown="False" w2125 {
            tunnel: w2121 -> [_ w2148]
            tunnel: w2124 -> [w2143 w2145]
            tunnel: [w2143 w2144] -> w2123
            tunnel: w2120 -> [_ _]
            tunnel: w2119 -> [_ _]
            frame False {
            }
            frame True {
              n518 = call "IMAQ Centroid"("Image"=w2148) -> ("Centroid"=w2147:cluster{"X Centroid":sgl, "Y Centroid":sgl})  [unwired: 3 in, 1 out]
              n519 = Unbundle(w2147) -> ("X Centroid"=w2146:sgl)  [unwired: 1 out]
              n520 = Build Array (concatenate)(w2145, w2146) -> (w2144:dbl[])
            }
          }
          n521 = Boolean To (0,1)(Boolean=w2125) -> (0, 1=w2127:i16)
          n522 = Replace Array Subset(array=w2129, new element=w2127, index=w2119) -> (w2128:dbl[])
        }
        "larvae size in scan" <- w2023
        n523 = stacked-sequence {
          seq-local: [w2047 _ _] -> [_ w2063 _]
          seq-local: [w2045 _ _] -> [_ w2062 _]
          seq-local: [w2046 _ _] -> [_ w2061 _]
          seq-local: [w2046 _ _] -> [_ w2059 _]
          seq-local: [w2045 _ _] -> [_ w2057 _]
          seq-local: [_ w2063 _] -> [_ _ w2067]
          seq-local: [_ w2062 _] -> [_ _ w2066]
          seq-local: [_ w2061 _] -> [_ _ w2065]
          seq-local: [_ w2053 _] -> [_ _ w2064]
          tunnel: w2023 -> [w2050 _ _]
          tunnel: w2022 -> [w2047 _ _]
          tunnel: w2020 -> [_ _ _]
          tunnel: [w2045 _ _] -> w2016
          tunnel: w2013 -> [_ w2060 _]
          tunnel: w2012 -> [_ w2058 _]
          tunnel: [_ w2056 _] -> w1979
          tunnel: [_ w2054 _] -> w1980
          tunnel: [_ _ w2067] -> w2021
          tunnel: [_ _ w2066] -> w2019
          tunnel: [_ _ w2065] -> w2018
          frame #0 {
            n524 = Reverse 1D Array(array=w2050) -> (reversed array=w2049:dbl[])
            n525 = Search 1D Array(1D array=w2050, element=1.0, start index (0)=0) -> (index of element=w2045:i32)
            n526 = Search 1D Array(1D array=w2049, element=1.0) -> (index of element=w2046:i32)  [unwired: 1 in]
          }
          frame #1 {
            n527 = Subtract(x=w2058, y=w2059) -> (x-y=w2056:i32)
            "real R2" <- w2056
            n528 = Subtract(x=w2060, y=w2056) -> ()  [unwired: 1 out]
            n529 = Subtract(x=w2056, y=w2057) -> (x-y=w2054:i32)
            "Larva length (# frames)" <- w2054
            n530 = Greater?(x=10.0, y=w2054) -> (0:w2053:bool)
          }
          frame #2 {
            n531 = case shown="True" w2064 {
              frame False {
                n532 = local write "um to move"("um to move long") -> ()
              }
              frame True {
                n533 = local write "um to move"("um to move short") -> ()
              }
            }
          }
        }
        n534 = Less?(x=16 ("y"), y=w1979) -> (x < y?=w1996:bool)
        n535 = Less?(x=w1980, y="maximum") -> (x < y?=w1981:bool)
        n536 = Less?(x="BUBBLE SIZE", y=w1980) -> (x < y?=w1982:bool)
        n537 = Greater?(x=w2016, y=0) -> (0:w1997:bool)
        n538 = And(x=w1982, y=w1981) -> (x .and. y?=w1977:bool)
        n539 = Less Or Equal?(x=w1979, y=85) -> (x <= y?=w1990:bool)
        n540 = And(x=w1997, y=w1996) -> (x .and. y?=w1992:bool)
        n541 = And(x=w1992, y=w1990) -> (x .and. y?=w1988:bool)
        n542 = And(x=w1977, y=w1988) -> (x .and. y?=w1989:bool)
        n543 = case shown="True" w2015 {
          tunnel: [states."Position_check" w2158] -> w2032
          tunnel: w1989 -> [_ w2157]
          tunnel: [w2151 w2156] -> w2004
          tunnel: w1963 -> [w2150 w2155]
          tunnel: [w2149 w2154] -> w1962
          tunnel: w1936 -> [_ w2153]
          frame False {
            n544 = call <vilib>:"High Resolution Relative Seconds.vi"() -> ("relative seconds"=w2151:dbl)
            n545 = call-poly <vilib>:"Mean.vi"("X"=w2150) -> ("mean"=w2149:dbl)  [unwired: 1 out]
            n546 = local write "center"(w2149) -> ()
          }
          frame True {
            n547 = case shown="True" w2157 {
              tunnel: [states."homing" states."Position_check"] -> w2158
              tunnel: w2155 -> [_ w2162]
              tunnel: [0.0 ("mean") w2161] -> w2154
              tunnel: w2153 -> [_ _]
              frame False {
              }
              frame True {
                n548 = call-poly <vilib>:"Mean.vi"("X"=w2162) -> ("mean"=w2161:dbl)  [unwired: 1 out]
                "center" <- w2161
              }
            }
            n549 = call <vilib>:"High Resolution Relative Seconds.vi"() -> ("relative seconds"=w2156:dbl)
          }
        }
        n550 = Subtract(x=w2004, y=w2007) -> (x-y=w2006:dbl)
        n551 = Insert Into Array(array=w2009, index=w2003, new element=w2006) -> (w2008:dbl[])
        n552 = Release Queue(queue=w1940) -> ()  [unwired: 2 in, 3 out]
        n553 = call <userlib>:"tm_stopcapture_40.vi"("error in (no error)"=w2027, "Handle in"=w2028) -> ("error out"=w1968:errorcluster, "Handle out"=w1955:u32)  [unwired: 8 in]
        n554 = call <userlib>:"tm_stoprecorder_40.vi"("Handle in"=w1955) -> ("Handle out"=w1954:u32)  [unwired: 9 in, 1 out]
        n555 = local read "Exposure time"() -> (w1939:dbl)
        n556 = call <userlib>:"tm_setparameter_40.vi"("error in (no error)"=w1968, "Value in"=w1939, "Parameter"=w1966, "Handle in"=w1954) -> ("error out"=w1967:errorcluster, "Handle out"=w1969:u32)  [unwired: 6 in]
        n557 = Build Array (concatenate)(w1960, w1962) -> (w1961:dbl[])
        "#of edgehunting" <- w2003
      }
      frame "Position_check" {
        n558 = stacked-sequence {
          seq-local: [w2220 _ _] -> [_ w2228 _]
          seq-local: [w2221 _ _] -> [_ w2226 _]
          seq-local: [_ w2227 _] -> [_ _ _]
          seq-local: [_ w2226 _] -> [_ _ _]
          seq-local: [_ w2223 _] -> [_ _ w2245]
          tunnel: [w2220 _ _] -> w2169
          tunnel: w2166 -> [w2220 _ _]
          tunnel: [_ w2225 _] -> w2168
          tunnel: [_ w2224 _] -> w2167
          tunnel: [_ _ w2245] -> w2165
          tunnel: [_ w2222 _] -> w2164
          frame #0 {
            n559 = call <vilib>:"Check if File or Folder Exists.vi"("path"=w2220) -> ("file or folder exists?"=w2221:bool)  [unwired: 8 in, 2 out]
          }
          frame #1 {
            n560 = case shown="True" w2226 {
              tunnel: w2228 -> [w2232 w2244]
              tunnel: [w2232 w2244] -> w2227
              tunnel: [1 ("Total Frames") w2234] -> w2225
              tunnel: [w2229 w2237] -> w2224
              tunnel: [1.0 w2241] -> w2223
              tunnel: [w2229 w2233] -> w2222
              frame False {
                w2229 = 0 ("Edge 1")
              }
              frame True {
                n561 = call "darksider.vi"("Path"=w2244) -> ("Edge 2"=w2233:i32, "lateral position indexs"=w2243:dbl[], "Total Frames"=w2236:i32, "index of element"=w2237:i32)  [unwired: 5 in, 2 out]
                "lateral position\n indexs" <- w2243
                n562 = Subtract(x=w2236, y=10) -> (x-y=w2234:i32)
                n563 = local read "um to move"() -> (w2240:u32)
                n564 = Array Size(array=w2243) -> (size(s)=w2242:i32)
                n565 = Multiply(x=w2240, y=u32 5) -> (x*y=w2238:u32)
                n566 = Divide(x=w2238, y=w2242) -> (x/y=w2241:dbl)
              }
            }
          }
          frame #2 {
          }
        }
        n567 = local read "Last saved #"() -> (w2183:i32)
        n568 = call <vilib>:"High Resolution Relative Seconds.vi"() -> ("relative seconds"=w2186:dbl)
        n569 = call-poly <vilib>:"DAQmx Write.vi"("task/channels in"=w2171, "data"=2.0) -> ("task out"=w2172:refnum<k21>)  [unwired: 11 in, 2 out]
        n570 = while {
          tunnel: w2196 -> [_]
          tunnel: w2198 -> [_]
          tunnel: w2201 -> [w2272]
          tunnel: [w2273] -> w2199
          tunnel: [w2269] -> w2180
          tunnel: w2168 -> [w2268]
          tunnel: w2167 -> [w2267]
          tunnel: w2164 -> [w2266]
          stop <- w2270 stop-if-true
          n571 = case shown="True" TRUE {
            tunnel: [w2275 w2294] -> w2273
            tunnel: [TRUE ("OK Done") w2283] -> w2270
            tunnel: w2272 -> [w2275 w2293]
            tunnel: [-1 w2281] -> w2269
            tunnel: w2268 -> [_ w2280]
            tunnel: w2267 -> [_ _]
            tunnel: w2266 -> [_ w2278]
            frame False {
            }
            frame True {
              n572 = flat-sequence {
                tunnel: [w2307] -> w2291
                tunnel: [w2299] -> w2289
                tunnel: [w2297] -> w2279
                tunnel: w2293 -> [w2307]
                tunnel: "\r\n" -> [w2299]
                tunnel: w2280 -> [w2297]
                tunnel: w2278 -> [w2296]
                tunnel: [w2295] -> w2277
                tunnel: w2291 -> [w2317]
                tunnel: [w2317] -> w2290
                tunnel: w2289 -> [w2316]
                tunnel: [w2316] -> w2288
                tunnel: [w2310] -> w2287
                tunnel: [w2310] -> w2281
                tunnel: w2279 -> [w2309]
                tunnel: w2277 -> [w2308]
                tunnel: [w2319] -> w2294
                tunnel: w2290 -> [w2319]
                tunnel: w2288 -> [w2318]
                tunnel: w2287 -> [w2320]
                tunnel: [w2323] -> w2286
                tunnel: [w2319] -> w2285
                tunnel: [w2318] -> w2284
                tunnel: w2286 -> [w2329]
                tunnel: w2285 -> [w2332]
                tunnel: w2284 -> [w2331]
                tunnel: [w2330] -> w2283
                tunnel: w2282 -> [w2328]
                frame #0 {
                  w2302 = u8 2 items=["0", "1", "2", "3", "4"] ("Axis Number")
                  n573 = Subtract(x=w2297, y=w2296) -> (x-y=w2295:i32)
                  n574 = call "RS232C_SetSpeed.vi"("Low Speed"=u32 100, "High Speed"=u32 20000, "Acceleration Time"=u16 100, "Axis Number"=w2302, "Delimiter"=w2299, "VISAリソース名"=w2307, "Axis Count"=u8 2, "Range"=TRUE, "Main/Sub"=FALSE) -> ()  [unwired: 2 out]
                  n575 = Wait (ms)(milliseconds to wait=u32 500) -> ()  [unwired: 1 out]
                }
                frame #1 {
                  n576 = local read "scanning distance (um)"() -> (w2314:u32)
                  n577 = Divide(x=w2308, y=w2309) -> (x/y=w2315:dbl)
                  n578 = Multiply(x=w2315, y=w2314) -> (x*y=w2312:dbl)
                  n579 = Add(x=w2312, y="correction") -> (x+y=w2311:dbl)
                  n580 = To Long Integer(number=w2311) -> (32bit integer=w2310:i32)
                  "backwards pulses" <- w2310
                }
                frame #2 {
                  w2326 = u8 2 items=["0", "1", "2", "3", "4"] ("Axis Number")
                  n581 = Wait (ms)(milliseconds to wait=u32 500) -> ()  [unwired: 1 out]
                  n582 = local read "Edge-hunting Direction"() -> (w2322:bool)
                  n583 = Not(x=w2322) -> (.not. x?=w2321:bool)
                  n584 = call "RS232C_Move.vi"("VISAリソース名"=w2319, "Axis Count"=u8 2, "Axis Number"=w2326, "Pulse Number"=w2320, "Direction"=w2321, "Delimiter"=w2318, "Main/Sub"=FALSE) -> ("OK Done"=w2323:bool)  [unwired: 1 out]
                }
                frame #3 {
                  n585 = case shown="False" w2328 {
                    tunnel: w2332 -> [_ w2341]
                    tunnel: w2331 -> [_ w2340]
                    tunnel: [w2333 w2335] -> w2330
                    tunnel: w2329 -> [w2333 _]
                    frame False {
                    }
                    frame True {
                      w2336 = u8 2 items=["0", "1", "2", "3", "4"] ("Axis Number")
                      w2338 = u32 2000 ("Low Speed")
                      n586 = Wait (ms)(milliseconds to wait=u32 500) -> ()  [unwired: 1 out]
                      n587 = call "RS232C_SetSpeed.vi"("Low Speed"=w2338, "High Speed"=w2338, "Acceleration Time"=u16 0, "Axis Number"=w2336, "Delimiter"=w2340, "VISAリソース名"=w2341, "Axis Count"=u8 2, "Range"=TRUE, "Main/Sub"=FALSE) -> ("OK Done"=w2335:bool)  [unwired: 1 out]
                    }
                  }
                }
              }
              n588 = local read "Enable screening\n(during flow zoometry)"() -> (w2282:bool)
            }
          }
        }
        n589 = local read "Continuous\nacquisition"() -> (w2181:bool)
        n590 = case shown="True" w2181 {
          tunnel: [w2249 w2256] -> w2193
          tunnel: [w2250 w2255] -> w2185
          tunnel: w2180 -> [w2246 _]
          tunnel: w2169 -> [_ _]
          frame False {
            n591 = Less?(x=w2246, y=0) -> (x < y?=w2247:bool)
            n592 = call <vilib>:"High Resolution Relative Seconds.vi"() -> ("relative seconds"=w2250:dbl)
            n593 = case shown="False" w2247 {
              tunnel: [states."Stream w/o flow" states."homing"] -> w2249
              frame False {
              }
              frame True {
                n594 = Wait (ms)(milliseconds to wait=u32 1000) -> ()  [unwired: 1 out]
              }
            }
          }
          frame True {
            n595 = case shown="False" "Enable screening\n(during flow zoometry)" {
              tunnel: [w2259 states."2000"] -> w2256
              tunnel: [w2258 w2264] -> w2255
              frame False {
                n596 = case shown="False" "4c" {
                  tunnel: [states."4climbo" states."405"] -> w2259
                  tunnel: [w2260 w2262] -> w2258
                  frame False {
                    n597 = call <vilib>:"High Resolution Relative Seconds.vi"() -> ("relative seconds"=w2260:dbl)
                  }
                  frame True {
                    n598 = call <vilib>:"High Resolution Relative Seconds.vi"() -> ("relative seconds"=w2262:dbl)
                  }
                }
              }
              frame True {
                n599 = call <vilib>:"High Resolution Relative Seconds.vi"() -> ("relative seconds"=w2264:dbl)
              }
            }
          }
        }
        n600 = Subtract(x=w2185, y=w2186) -> (x-y=w2184:dbl)
        "gp" <- w2184
        n601 = Insert Into Array(array=w2187, index=w2183, new element=w2184) -> (w2182:dbl[])
      }
      frame "homing" {
        n602 = local write "Moving"(TRUE ("Moving")) -> ()
        n603 = call <vilib>:"Check if File or Folder Exists.vi"("path"=w2348) -> ("file or folder exists?"=w2351:bool, "dup path"=w2350:path)  [unwired: 8 in, 1 out]
        n604 = flat-sequence {
          tunnel: w2371 -> [w2413]
          tunnel: w2351 -> [w2411]
          tunnel: w2350 -> [w2410]
          tunnel: [w2402] -> w2345
          tunnel: [w2435] -> w2372
          tunnel: w2361 -> [w2430]
          tunnel: w2359 -> [w2429]
          tunnel: [w2417] -> w2349
          tunnel: [w2416] -> w2346
          tunnel: w2345 -> [w2416]
          tunnel: w2372 -> [w2516]
          tunnel: w2371 -> [w2517]
          tunnel: w2346 -> [w2509]
          frame #0 {
            w2402 = "\r\n"
            w2408 = u8 2 items=["0", "1", "2", "3", "4"] ("Axis Number")
            n605 = case shown="False" w2411 {
              tunnel: w2410 -> [_ w2414]
              frame False {
              }
              frame True {
                n606 = Delete(path (use dialog)=w2414) -> ()  [unwired: 4 in, 3 out]
              }
            }
            n607 = call "RS232C_SetSpeed.vi"("Low Speed"=u32 100, "High Speed"=u32 20000 ("Go to edge speed 2"), "Acceleration Time"=u16 100, "Axis Number"=w2408, "Delimiter"=w2402, "VISAリソース名"=w2413, "Axis Count"=u8 2, "Range"=TRUE, "Main/Sub"=TRUE) -> ("OK Done"=→"homing speed":bool)  [unwired: 1 out]
          }
          frame #1 {
            n608 = local read "Larva length (# frames)"() -> (w2418:i32)
            n609 = local read "maximum"() -> (w2419:i32)
            n610 = local read "BUBBLE SIZE"() -> (w2421:i32)
            n611 = local read "screening"() -> (w2433:bool)
            n612 = local read "real R2"() -> (w2424:i32)
            n613 = local read "real R2"() -> (w2427:i32)
            n614 = Greater?(x=w2419, y=w2418) -> (0:w2420:bool)
            n615 = Wait (ms)(milliseconds to wait=u32 500) -> ()  [unwired: 1 out]
            n616 = Greater?(x=w2430, y=0) -> (0:w2431:bool)
            n617 = local read "4c"() -> (w2415:bool)
            n618 = Less?(x=w2427, y=16) -> (x < y?=w2425:bool)
            "r216" <- w2425
            n619 = Less Or Equal?(x=w2424, y=85) -> (x <= y?=w2422:bool)
            "r285" <- w2422
            n620 = Greater?(x=w2418, y=w2421) -> (0:w2428:bool)
            "larva size" <- w2428
            n621 = case shown="True" w2415 {
              tunnel: [w2438 w2450] -> w2435
              tunnel: w2433 -> [w2437 _]
              tunnel: w2431 -> [_ w2449]
              tunnel: w2429 -> [_ w2448]
              tunnel: w2428 -> [_ w2447]
              tunnel: w2425 -> [_ w2446]
              tunnel: w2422 -> [_ w2445]
              tunnel: w2420 -> [_ w2444]
              tunnel: [TRUE w2443] -> w2417
              frame False {
                n622 = case shown="False" w2437 {
                  tunnel: [w2439 w2441] -> w2438
                  frame False {
                    n623 = local read "scanning distance (um)"() -> (w2439:u32)
                  }
                  frame True {
                    n624 = local read "backwards pulses"() -> (w2440:i32)
                    n625 = local read "scanning distance (um)"() -> (w2442:u32)
                    n626 = Subtract(x=w2442, y=w2440) -> (x-y=w2441:u32)
                  }
                }
              }
              frame True {
                n627 = case shown="True" w2449 {
                  tunnel: [w2452 w2462] -> w2450
                  tunnel: w2448 -> [_ w2458]
                  tunnel: w2447 -> [_ w2457]
                  tunnel: w2446 -> [_ w2456]
                  tunnel: w2445 -> [_ w2455]
                  tunnel: w2444 -> [_ w2454]
                  tunnel: [TRUE w2453] -> w2443
                  frame False {
                    n628 = local read "scanning distance (um)"() -> (w2452:u32)
                  }
                  frame True {
                    n629 = local read "backwards pulses"() -> (w2461:i32)
                    n630 = Greater?(x=w2461, y=0) -> (0:w2459:bool)
                    n631 = case shown="True" w2459 {
                      tunnel: [w2464 w2472] -> w2462
                      tunnel: w2461 -> [_ w2471]
                      tunnel: w2458 -> [_ w2470]
                      tunnel: w2457 -> [_ w2469]
                      tunnel: w2456 -> [_ w2468]
                      tunnel: w2455 -> [_ w2467]
                      tunnel: w2454 -> [_ w2466]
                      tunnel: [TRUE w2465] -> w2453
                      frame False {
                        n632 = local read "scanning distance (um)"() -> (w2464:u32)
                      }
                      frame True {
                        n633 = case shown="False" w2470 {
                          tunnel: [w2479 w2508] -> w2472
                          tunnel: w2471 -> [w2478 _]
                          tunnel: w2469 -> [w2477 _]
                          tunnel: w2468 -> [w2476 _]
                          tunnel: w2467 -> [w2475 _]
                          tunnel: w2466 -> [w2474 _]
                          tunnel: [w2473 TRUE] -> w2465
                          frame False {
                            n634 = case shown="True" w2477 {
                              tunnel: [w2481 w2487] -> w2479
                              tunnel: w2478 -> [_ w2486]
                              tunnel: w2476 -> [_ w2485]
                              tunnel: w2475 -> [_ w2484]
                              tunnel: w2474 -> [_ w2483]
                              tunnel: [TRUE w2482] -> w2473
                              frame False {
                                n635 = local read "scanning distance (um)"() -> (w2481:u32)
                              }
                              frame True {
                                n636 = case shown="False" w2485 {
                                tunnel: [w2492 w2506] -> w2487
                                tunnel: w2486 -> [w2491 _]
                                tunnel: w2484 -> [w2490 _]
                                tunnel: w2483 -> [w2489 _]
                                tunnel: [w2488 TRUE] -> w2482
                                frame False {
                                n637 = case shown="True" w2490 {
                                tunnel: [w2494 w2498] -> w2492
                                tunnel: w2491 -> [_ w2497]
                                tunnel: w2489 -> [_ w2496]
                                tunnel: [TRUE w2495] -> w2488
                                frame False {
                                n638 = local read "scanning distance (um)"() -> (w2494:u32)
                                }
                                frame True {
                                n639 = case shown="True" w2496 {
                                tunnel: [w2500 w2503] -> w2498
                                tunnel: w2497 -> [_ w2502]
                                tunnel: [TRUE FALSE] -> w2495
                                frame False {
                                n640 = local read "scanning distance (um)"() -> (w2500:u32)
                                }
                                frame True {
                                n641 = local read "scanning distance (um)"() -> (w2504:u32)
                                n642 = Subtract(x=w2504, y=w2502) -> (x-y=w2503:u32)
                                }
                                }
                                }
                                }
                                }
                                frame True {
                                n643 = local read "scanning distance (um)"() -> (w2506:u32)
                                }
                                }
                              }
                            }
                          }
                          frame True {
                            n644 = local read "scanning distance (um)"() -> (w2508:u32)
                          }
                        }
                      }
                    }
                  }
                }
              }
            }
            "Homing distance" <- w2435
          }
          frame #2 {
            w2513 = u8 2 items=["0", "1", "2", "3", "4"] ("Axis Number")
            n645 = local write "screening"(FALSE ("screening 2")) -> ()
            n646 = call "RS232C_Move.vi"("VISAリソース名"=w2517, "Axis Count"=u8 2, "Axis Number"=w2513, "Pulse Number"=w2516, "Direction"=TRUE, "Delimiter"=w2509, "Main/Sub"=FALSE) -> ("OK Done"=→"homing":bool)  [unwired: 1 out]
          }
        }
        n647 = Increment(x=w2394) -> (x+1=w2393:i32)
        "False triggers" <- w2393
        n648 = local read "maximum"() -> (w2358:i32)
        n649 = local read "Larva length (# frames)"() -> (w2367:i32)
        n650 = local read "Continuous\nacquisition"() -> (w2399:bool)
        n651 = Greater?(x=w2367, y=w2358) -> (0:w2364:bool)
        n652 = Less?(x=w2367, y=100) -> (x < y?=w2365:bool)
        n653 = And(x=w2365, y=w2364) -> (x .and. y?=w2359:bool)
        n654 = case shown="True" w2399 {
          tunnel: [states."Chilling" w2523] -> w2398
          tunnel: [FALSE ("homing speed") FALSE ("homing speed")] -> w2370
          tunnel: w2359 -> [_ w2521]
          tunnel: w2349 -> [_ w2520]
          frame False {
          }
          frame True {
            n655 = case shown="False" w2521 {
              tunnel: [w2525 states."light reverse"] -> w2523
              tunnel: w2520 -> [w2524 _]
              frame False {
                n656 = case shown="False" w2524 {
                  tunnel: [states."405_r" states."auto imaging"] -> w2525
                  frame False {
                  }
                  frame True {
                  }
                }
              }
              frame True {
              }
            }
          }
        }
        n657 = local write "homing speed"(w2370) -> ()
        n658 = local write "homing"(w2370) -> ()
      }
      frame "Acquire" {
        w2536 = "_" ("string")
        # "file naming"
        n659 = Format Into String(format string="%04d", w2556) -> (resulting string=w2587:string)  [unwired: 2 in, 1 out]
        n660 = local read "Frames in memory 2"() -> (w2533:i32)
        n661 = Increment(x=w2594) -> (x+1=w2593:i32)
        n662 = Increment(x=w2551) -> (x+1=w2555:i32)
        n663 = local read "Last saved file number 2000"() -> (w2562:i32)
        n664 = Number To Decimal String(number=w2562, width (-)=i16 0) -> ()  [unwired: 1 out]
        n665 = Add(x=1, y=w2556) -> (x+y=w2612:i32)
        n666 = local write "screening"(FALSE ("screening 2")) -> ()
        n667 = Insert Into Array(array=w2615, index=w2612, new element=w2614) -> (w2613:string[])
        n668 = local read "lateral position\n indexs"() -> (w2544:dbl[])
        n669 = Path To String(path=w2529) -> (string=w2598:string)
        n670 = Concatenate Strings(w2598, "\\temp\\" ("string"), w2604, w2536, w2587, w2536) -> (w2636:string)
        n671 = call-poly <vilib>:"DAQmx Write.vi"("task/channels in"=w2538, "data"=FALSE) -> ()  [unwired: 11 in, 3 out]
        n672 = node-c288("Focus changing \nperiod (ms)") -> (w2541:T6)  [unwired: 3 in]
        n673 = String To Path(string=w2636) -> (path=w2599:path)
        "Last saved file" <- w2599
        n674 = call <userlib>:"tm_startrecorder_40.vi"("error in (no error)"=w2628, "frames"=w2533, "File"=w2599, "Handle in"=w2627) -> ("error out"=w2626:errorcluster, "Handle out"=w2625:u32)  [unwired: 6 in]
        n675 = call <userlib>:"tm_startcapture_40.vi"("error in (no error)"=w2626, "Handle in"=w2625) -> ("error out"=w2624:errorcluster, "Handle out"=w2623:u32)  [unwired: 8 in]
        n676 = Array Size(array=w2544) -> (size(s)=w2530:i32)
        n677 = Less?(x="# to measure", y=w2612) -> (x < y?=w2633:bool)
        n678 = flat-sequence {
          tunnel: [w2781] -> w2619
          tunnel: [w2782] -> w2628
          tunnel: [w2783] -> w2627
          tunnel: [w2775] -> w2630
          tunnel: w2641 -> [w2781]
          tunnel: w2644 -> [w2782]
          tunnel: w2643 -> [w2783]
          frame #0 {
            w2775 = "\r\n"
            w2777 = u8 2 items=["0", "1", "2", "3", "4"] ("Axis Number")
            n679 = Wait (ms)(milliseconds to wait=u32 100) -> ()  [unwired: 1 out]
            n680 = call "RS232C_SetSpeed.vi"("Low Speed"="Acquire speed (um/s)", "High Speed"="Acquire speed (um/s)", "Acceleration Time"=u16 0, "Axis Number"=w2777, "Delimiter"=w2775, "VISAリソース名"=w2781, "Axis Count"=u8 2, "Range"="Range 2", "Main/Sub"=TRUE) -> ()  [unwired: 2 out]
          }
        }
        n681 = Or(x=w2633, y="Continuous\nacquisition") -> ()  [unwired: 1 out]
        n682 = local read "Larvae until move"() -> (w2595:i32)
        n683 = local read "loading tube#"() -> (w2573:i32)
        n684 = Less?(x=w2573, y=7) -> (x < y?=w2570:bool)
        n685 = Greater?(x=w2595, y="Larva # to move") -> (0:w2571:bool)
        n686 = And(x=w2571, y=w2570) -> ()  [unwired: 1 out]
        n687 = local read "backwards pulses"() -> (w2569:i32)
        n688 = local read "scanning distance (um)"() -> (w2554:u32)
        n689 = local read "um to move"() -> (w2550:u32)
        n690 = Add(x=w2550, y=w2569) -> (x+y=w2578:u32)
        n691 = Subtract(x=w2554, y=w2550) -> (x-y=w2567:u32)
        n692 = Subtract(x=w2554, y=w2578) -> (x-y=w2576:u32)
        n693 = Greater?(x=0, y=w2569) -> (0:w2577:bool)
        n694 = while {
          tunnel: w2630 -> [w2730]
          tunnel: w2619 -> [w2736]
          tunnel: [w2735] -> w2532
          tunnel: [w2734] -> w2542
          tunnel: [w2733] -> w2549
          tunnel: "Movement direction" -> [w2733]
          tunnel: [w2732] -> _
          tunnel: [w2731] -> _
          tunnel: [w2728] -> w2617
          tunnel: [w2727] -> _
          tunnel: [w2728] -> w2534
          stop <- w2729 stop-if-true
          # "Move to scan larva"
          n695 = stacked-sequence {
            seq-local: [w2739 _ _] -> [_ w2752 _]
            seq-local: [w2738 _ _] -> [_ w2747 _]
            seq-local: [_ w2752 _] -> [_ _ w2756]
            tunnel: w2736 -> [w2739 _ _]
            tunnel: w2733 -> [w2738 _ _]
            tunnel: [w2737 _ _] -> w2731
            tunnel: w2730 -> [_ _ _]
            tunnel: w2730 -> [_ w2748 _]
            tunnel: [_ "um to move" _] -> w2728
            tunnel: [_ "um to move" _] -> w2727
            tunnel: [_ w2745 _] -> w2729
            tunnel: [_ _ w2756] -> w2735
            tunnel: [_ _ w2753] -> w2732
            frame #0 {
              n696 = Wait (ms)(milliseconds to wait=u32 500) -> ()  [unwired: 1 out]
              n697 = for {
                N: 1 -> [_]
                tunnel: [w2742] -> w2737
                n698 = local read "Sub img mean"() -> (w2743:dbl)
                n699 = local read "Mean trigger"() -> (w2744:i32)
                n700 = Greater Or Equal?(x=w2743, y=w2744) -> (x >= y?=w2742:bool)
              }
            }
            frame #1 {
              w2750 = u8 2 items=["0", "1", "2", "3", "4"] ("Axis Number")
              # "Extra scan"
              n701 = call "RS232C_Move.vi"("VISAリソース名"=w2752, "Axis Count"=u8 2, "Axis Number"=w2750, "Pulse Number"="um to move", "Direction"=w2747, "Delimiter"=w2748, "Main/Sub"=FALSE) -> ("OK Done"=w2745:bool)  [unwired: 1 out]
            }
            frame #2 {
              n702 = local read "Mean trigger"() -> (w2755:i32)
              n703 = local read "Sub img mean"() -> (w2754:dbl)
              n704 = Greater?(x=w2754, y=w2755) -> (0:w2753:bool)
            }
          }
          n705 = call <extravilib>:"Write.vi"("element"=w2729) -> ("channel"=w2734:T13)  [unwired: 1 out]
        }
        n706 = timed-loop {
          shift-right: [w2680] -> w2545
          shift-left: w2546 -> [w2681]
          tunnel: w2544 -> [w2679]
          tunnel: "Focus changing \nperiod (ms)" -> [_]
          tunnel: w2542 -> [w2678]
          timing: w2541 -> [_]
          timing-out: [_] -> w2540
          tunnel: w2530 -> [w2676]
          i -> [w2677]
          stop <- w2673 stop-if-true
          n707 = node-c288() -> ()  [unwired: 1 in, 1 out]
          n708 = Index Array(array=w2679, index=w2677) -> (element=w2672:dbl)
          n709 = Subtract(x=w2672, y="element 3") -> (x-y=w2670:dbl)
          n710 = Divide(x=w2670, y="y 2") -> (x/y=w2669:dbl)
          n711 = Multiply(x="x", y=w2669) -> (x*y=w2666:dbl)
          n712 = Add(x=w2666, y="y 3") -> (x+y=w2664:dbl)
          "Focal position" <- w2664
          n713 = Greater?(x=w2677, y=w2676) -> (0:w2675:bool)
          n714 = call <extravilib>:"Read.vi"("channel"=w2678) -> ("element"=w2674:bool)  [unwired: 1 in, 1 out]
          n715 = call-poly <vilib>:"DAQmx Write.vi"("task/channels in"=w2681, "data"=w2664) -> ("task out"=w2680:refnum<k21>)  [unwired: 11 in, 2 out]
          n716 = Or(x=w2674, y=w2675) -> (x .or. y?=w2673:bool)
          n717 = node-c288() -> ()  [unwired: 1 in, 1 out]
          "Timed loop#" <- w2677
        }
        n718 = while {
          tunnel: w2623 -> [w2772]
          tunnel: w2624 -> [w2771]
          tunnel: [w2768] -> w2640
          tunnel: [w2767] -> w2639
          tunnel: w2542 -> [w2770]
          tunnel: w2629 -> [w2764]
          stop <- w2769 stop-if-true
          n719 = call <userlib>:"tm_waitnextframe_40.vi"("error in (no error)"=w2771, "Handle in"=w2772) -> ("error out"=w2767:errorcluster, "Frame Count"=w2763:i32, "Frame Index"=w2766:i32, "Handle out"=w2768:u32)  [unwired: 6 in]
          n720 = call <extravilib>:"Read.vi"("channel"=w2770) -> ("element"=w2769:bool)  [unwired: 1 in, 1 out]
          n721 = local write "Frame count"(w2763) -> ()
          n722 = Index Array(array=w2764, index=w2766) -> (element=w2765:T12)
          n723 = Multiply(x=2048, y=2048) -> (x*y=w2762:i32)
          n724 = call "IMAQ ImageToArray"("Image"=w2765) -> ("Image Pixels (U16)"=w2759:u16[][])  [unwired: 3 in, 4 out]
          n725 = local write "Obtained image"(w2759) -> ()
          n726 = Reshape Array(w2759, w2762) -> (w2758:u16[])
          n727 = call-poly <vilib>:"Mean.vi"("X"=w2758) -> ("mean"=w2757:dbl)  [unwired: 1 out]
          n728 = local write "Mean intensity\nof frame"(w2757) -> ()
        }
        n729 = node-c288(w2540) -> ()  [unwired: 1 out]
        n730 = call <userlib>:"tm_stopcapture_40.vi"("error in (no error)"=w2639, "Handle in"=w2640) -> ("error out"=w2637:errorcluster, "Handle out"=w2638:u32)  [unwired: 8 in]
        n731 = call <userlib>:"tm_stoprecorder_40.vi"("error in (no error)"=w2637, "Handle in"=w2638) -> ("error out"=w2601:errorcluster, "Handle out"=w2603:u32)  [unwired: 8 in]
        n732 = flat-sequence {
          tunnel: w2548 -> [w2717]
          tunnel: w2532 -> [w2716]
          tunnel: [w2716] -> w2622
          tunnel: [w2717] -> w2621
          tunnel: [w2715] -> w2620
          tunnel: [w2724] -> w2631
          tunnel: w2622 -> [w2724]
          tunnel: w2621 -> [w2720]
          tunnel: w2620 -> [w2723]
          tunnel: w2618 -> [_]
          tunnel: w2617 -> [_]
          tunnel: w2583 -> [_]
          tunnel: w2534 -> [w2718]
          frame #0 {
            w2709 = u8 2 items=["0", "1", "2", "3", "4"] ("Axis Number")
            w2715 = "\r\n"
            n733 = call "RS232C_SetSpeed.vi"("Low Speed"=u32 100, "High Speed"=u16 10000 ("Acceleration Time"), "Acceleration Time"=u16 100, "Axis Number"=w2709, "Delimiter"=w2715, "VISAリソース名"=w2716, "Axis Count"=u8 2, "Range"=TRUE, "Main/Sub"=TRUE) -> ()  [unwired: 2 out]
          }
          frame #1 {
            w2725 = u8 2 items=["0", "1", "2", "3", "4"] ("Axis Number")
            n734 = Wait (ms)(milliseconds to wait=u32 500) -> ()  [unwired: 1 out]
            n735 = Not(x=w2720) -> (.not. x?=w2719:bool)
            n736 = call "RS232C_Move.vi"("VISAリソース名"=w2724, "Axis Count"=u8 2, "Axis Number"=w2725, "Pulse Number"=w2718, "Direction"=w2719, "Delimiter"=w2723, "Main/Sub"=FALSE) -> ()  [unwired: 2 out]
          }
        }
        n737 = stacked-sequence {
          seq-local: [w2646 _] -> [_ w2663]
          seq-local: [w2649 _] -> [_ w2662]
          seq-local: [w2648 _] -> [_ w2653]
          seq-local: [w2647 _] -> [_ w2661]
          tunnel: w2603 -> [w2646 _]
          tunnel: w2601 -> [w2649 _]
          tunnel: w2599 -> [w2648 _]
          tunnel: w2598 -> [w2647 _]
          tunnel: [_ w2663] -> w2602
          tunnel: [_ w2662] -> w2600
          frame #0 {
            n738 = Wait (ms)(milliseconds to wait=u32 100) -> ()  [unwired: 1 out]
          }
          frame #1 {
            n739 = Path To String(path=w2653) -> (string=w2652:string)
            n740 = Strip Path(path=w2653) -> (name=w2657:string)  [unwired: 1 out]
            n741 = Concatenate Strings(w2652, ".dcimg" ("string")) -> (w2650:string)
            n742 = Concatenate Strings(w2657, ".dcimg" ("string")) -> (w2655:string)
            n743 = Concatenate Strings(w2661, "\\raw\\" ("string"), w2655) -> (w2659:string)
            n744 = String To Path(string=w2650) -> (path=w2654:path)
            n745 = String To Path(string=w2659) -> (path=w2658:path)
            n746 = Move(source path=w2654, 10:w2658) -> ()  [unwired: 3 in, 3 out]
          }
        }
        n747 = Greater?(x=w2551, y=1.0) -> (0:w2553:bool)
        n748 = case shown="True" w2577 {
          tunnel: w2576 -> [w2693 _]
          tunnel: [w2692 w2702] -> w2583
          tunnel: w2567 -> [_ w2703]
          tunnel: w2550 -> [w2691 w2701]
          tunnel: w2553 -> [w2688 w2700]
          tunnel: w2549 -> [w2690 w2699]
          tunnel: [w2689 w2698] -> w2548
          frame False {
            n749 = case shown="True" w2688 {
              tunnel: w2693 -> [w2694 w2697]
              tunnel: [w2694 w2697] -> w2692
              tunnel: w2691 -> [_ _]
              tunnel: w2690 -> [w2695 w2696]
              tunnel: [w2695 w2696] -> w2689
              frame False {
              }
              frame True {
              }
            }
          }
          frame True {
            n750 = case shown="False" w2700 {
              tunnel: w2703 -> [w2704 w2707]
              tunnel: [w2704 w2707] -> w2702
              tunnel: w2701 -> [_ _]
              tunnel: w2699 -> [w2705 w2706]
              tunnel: [w2705 w2706] -> w2698
              frame False {
              }
              frame True {
              }
            }
          }
        }
        "Last saved #" <- w2556
      }
      frame "acquire without AF" {
        w2791 = "_" ("string")
        n751 = local read "Last saved file number 2000"() -> (w2810:i32)
        n752 = local read "Frames in memory 2"() -> (w2787:i32)
        n753 = Increment(x=w2799) -> (x+1=w2803:i32)
        n754 = Number To Decimal String(number=w2810, width (-)=i16 0) -> ()  [unwired: 1 out]
        n755 = local write "screening"(FALSE ("screening 2")) -> ()
        n756 = Format Into String(format string="%04d", w2788) -> (resulting string=w2836:string)  [unwired: 2 in, 1 out]
        n757 = Insert Into Array(array=w2860, index=w2788, new element=w2859) -> (w2858:string[])
        n758 = local read "Continuous\nacquisition"() -> (w2786:bool)
        n759 = Path To String(path=w2882) -> (string=w2844:string)
        n760 = Concatenate Strings(w2844, "\\temp\\" ("string"), w2850, w2791, w2836, w2791, "noaf" ("string")) -> (w2883:string)
        n761 = String To Path(string=w2883) -> (path=w2845:path)
        "Last saved file 2" <- w2845
        n762 = call-poly <vilib>:"DAQmx Write.vi"("task/channels in"=w2793, "data"=FALSE) -> ()  [unwired: 11 in, 3 out]
        n763 = call <userlib>:"tm_startrecorder_40.vi"("error in (no error)"=w2873, "frames"=w2787, "File"=w2845, "Handle in"=w2872) -> ("error out"=w2871:errorcluster, "Handle out"=w2870:u32)  [unwired: 6 in]
        n764 = call <userlib>:"tm_startcapture_40.vi"("error in (no error)"=w2871, "Handle in"=w2870) -> ("error out"=w2869:errorcluster, "Handle out"=w2868:u32)  [unwired: 8 in]
        n765 = Less?(x="# to measure 2", y=w2788) -> (x < y?=w2879:bool)
        n766 = flat-sequence {
          tunnel: [w3017] -> w2864
          tunnel: [w3018] -> w2873
          tunnel: [w3019] -> w2872
          tunnel: [w3011] -> w2875
          tunnel: w2888 -> [w3017]
          tunnel: w2891 -> [w3018]
          tunnel: w2890 -> [w3019]
          frame #0 {
            w3011 = "\r\n"
            w3013 = u8 2 items=["0", "1", "2", "3", "4"] ("Axis Number")
            n767 = local read "Acquire speed (um/s)"() -> (w3009:u32)
            n768 = Wait (ms)(milliseconds to wait=u32 100) -> ()  [unwired: 1 out]
            n769 = call "RS232C_SetSpeed.vi"("Low Speed"=w3009, "High Speed"=w3009, "Acceleration Time"=u16 0, "Axis Number"=w3013, "Delimiter"=w3011, "VISAリソース名"=w3017, "Axis Count"=u8 2, "Range"="Range 3", "Main/Sub"=TRUE) -> ()  [unwired: 2 out]
          }
        }
        n770 = Or(x=w2879, y=w2786) -> (x .or. y?=w2878:bool)
        n771 = local read "Larvae until move"() -> (w2841:i32)
        n772 = local read "Larva # to move"() -> (w2785:i32)
        n773 = local read "loading tube#"() -> (w2822:i32)
        n774 = Less?(x=w2822, y=7) -> (x < y?=w2819:bool)
        n775 = local read "405 2"() -> (w2805:bool)
        n776 = Greater?(x=w2841, y=w2785) -> (0:w2820:bool)
        n777 = And(x=w2820, y=w2819) -> (x .and. y?=w2818:bool)
        n778 = local read "Movement direction"() -> (w2784:bool)
        n779 = while {
          tunnel: w2875 -> [w2966]
          tunnel: w2864 -> [w2972]
          tunnel: [w2971] -> w2877
          tunnel: [w2970] -> w2795
          tunnel: w2784 -> [w2969]
          tunnel: [w2969] -> _
          tunnel: [w2968] -> _
          tunnel: [w2967] -> _
          tunnel: [w2965] -> w2862
          tunnel: [w2964] -> _
          stop <- w2963 stop-if-true
          # "Move to scan larva"
          n780 = stacked-sequence {
            seq-local: [w2975 _ _] -> [_ w2988 _]
            seq-local: [w2974 _ _] -> [_ w2983 _]
            seq-local: [_ w2988 _] -> [_ _ w2992]
            tunnel: w2972 -> [w2975 _ _]
            tunnel: w2969 -> [w2974 _ _]
            tunnel: [w2973 _ _] -> w2967
            tunnel: w2966 -> [_ _ _]
            tunnel: w2966 -> [_ w2984 _]
            tunnel: [_ w2981 _] -> w2965
            tunnel: [_ w2981 _] -> w2964
            tunnel: [_ w2982 _] -> w2963
            tunnel: [_ _ w2992] -> w2971
            tunnel: [_ _ w2989] -> w2968
            frame #0 {
              n781 = Wait (ms)(milliseconds to wait=u32 500) -> ()  [unwired: 1 out]
              n782 = for {
                N: 1 -> [_]
                tunnel: [w2978] -> w2973
                n783 = local read "Sub img mean"() -> (w2979:dbl)
                n784 = local read "Mean trigger"() -> (w2980:i32)
                n785 = Greater Or Equal?(x=w2979, y=w2980) -> (x >= y?=w2978:bool)
              }
            }
            frame #1 {
              w2986 = u8 2 items=["0", "1", "2", "3", "4"] ("Axis Number")
              # "Extra scan"
              n786 = local read "um to move"() -> (w2981:u32)
              n787 = call "RS232C_Move.vi"("VISAリソース名"=w2988, "Axis Count"=u8 2, "Axis Number"=w2986, "Pulse Number"=w2981, "Direction"=w2983, "Delimiter"=w2984, "Main/Sub"=FALSE) -> ("OK Done"=w2982:bool)  [unwired: 1 out]
            }
            frame #2 {
              n788 = local read "Mean trigger"() -> (w2991:i32)
              n789 = local read "Sub img mean"() -> (w2990:dbl)
              n790 = Greater?(x=w2990, y=w2991) -> (0:w2989:bool)
            }
          }
          n791 = call <extravilib>:"Write.vi"("element"=w2963) -> ("channel"=w2970:T13)  [unwired: 1 out]
        }
        n792 = while {
          tunnel: w2868 -> [w3008]
          tunnel: w2869 -> [w3007]
          tunnel: [w3004] -> w2887
          tunnel: [w3003] -> w2886
          tunnel: w2795 -> [w3006]
          tunnel: w2874 -> [w3000]
          stop <- w3005 stop-if-true
          n793 = call <userlib>:"tm_waitnextframe_40.vi"("error in (no error)"=w3007, "Handle in"=w3008) -> ("error out"=w3003:errorcluster, "Frame Count"=w2999:i32, "Frame Index"=w3002:i32, "Handle out"=w3004:u32)  [unwired: 6 in]
          n794 = call <extravilib>:"Read.vi"("channel"=w3006) -> ("element"=w3005:bool)  [unwired: 1 in, 1 out]
          n795 = local write "Frame count"(w2999) -> ()
          n796 = Index Array(array=w3000, index=w3002) -> (element=w3001:T12)
          n797 = Multiply(x=2048, y=2048) -> (x*y=w2998:i32)
          n798 = call "IMAQ ImageToArray"("Image"=w3001) -> ("Image Pixels (U16)"=w2995:u16[][])  [unwired: 3 in, 4 out]
          n799 = local write "Obtained image"(w2995) -> ()
          n800 = Reshape Array(w2995, w2998) -> (w2994:u16[])
          n801 = call-poly <vilib>:"Mean.vi"("X"=w2994) -> ("mean"=w2993:dbl)  [unwired: 1 out]
          n802 = local write "Mean intensity\nof frame"(w2993) -> ()
        }
        n803 = call <userlib>:"tm_stopcapture_40.vi"("error in (no error)"=w2886, "Handle in"=w2887) -> ("error out"=w2884:errorcluster, "Handle out"=w2885:u32)  [unwired: 8 in]
        n804 = call <userlib>:"tm_stoprecorder_40.vi"("error in (no error)"=w2884, "Handle in"=w2885) -> ("error out"=w2847:errorcluster, "Handle out"=w2849:u32)  [unwired: 8 in]
        n805 = stacked-sequence {
          seq-local: [w2893 _] -> [_ w2910]
          seq-local: [w2896 _] -> [_ w2909]
          seq-local: [w2895 _] -> [_ w2900]
          seq-local: [w2894 _] -> [_ w2908]
          tunnel: w2849 -> [w2893 _]
          tunnel: w2847 -> [w2896 _]
          tunnel: w2845 -> [w2895 _]
          tunnel: w2844 -> [w2894 _]
          tunnel: [_ w2910] -> w2848
          tunnel: [_ w2909] -> w2846
          frame #0 {
            n806 = Wait (ms)(milliseconds to wait=u32 100) -> ()  [unwired: 1 out]
          }
          frame #1 {
            n807 = Path To String(path=w2900) -> (string=w2899:string)
            n808 = Strip Path(path=w2900) -> (name=w2904:string)  [unwired: 1 out]
            n809 = Concatenate Strings(w2899, ".dcimg" ("string")) -> (w2897:string)
            n810 = Concatenate Strings(w2904, ".dcimg" ("string")) -> (w2902:string)
            n811 = Concatenate Strings(w2908, "\\raw\\" ("string"), w2902) -> (w2906:string)
            n812 = String To Path(string=w2897) -> (path=w2901:path)
            n813 = String To Path(string=w2906) -> (path=w2905:path)
            n814 = Move(source path=w2901, 10:w2905) -> ()  [unwired: 3 in, 3 out]
          }
        }
        n815 = local read "backwards pulses"() -> (w2817:i32)
        n816 = Greater?(x=0, y=w2817) -> (0:w2826:bool)
        n817 = case shown="True" w2878 {
          tunnel: [states."Chilling" w2953] -> w2880
          tunnel: w2818 -> [_ w2952]
          tunnel: w2826 -> [_ w2951]
          tunnel: w2805 -> [_ w2950]
          frame False {
          }
          frame True {
            n818 = case shown="False" w2950 {
              tunnel: [w2956 states."auto imaging"] -> w2953
              tunnel: w2952 -> [w2955 _]
              tunnel: w2951 -> [w2954 _]
              frame False {
                n819 = case shown="True" w2955 {
                  tunnel: [w2958 states."405_r"] -> w2956
                  tunnel: w2954 -> [w2957 _]
                  frame False {
                    n820 = case shown="True" w2957 {
                      tunnel: [states."405_r" states."405_r"] -> w2958
                      frame False {
                      }
                      frame True {
                      }
                    }
                  }
                  frame True {
                  }
                }
              }
              frame True {
              }
            }
          }
        }
        n821 = flat-sequence {
          tunnel: w2797 -> [w2940]
          tunnel: w2877 -> [w2939]
          tunnel: [w2939] -> w2867
          tunnel: [w2940] -> w2866
          tunnel: [w2938] -> w2865
          tunnel: [w2946] -> w2876
          tunnel: w2867 -> [w2946]
          tunnel: w2866 -> [w2942]
          tunnel: w2865 -> [w2945]
          tunnel: w2863 -> [_]
          tunnel: w2862 -> [_]
          tunnel: w2832 -> [w2941]
          frame #0 {
            w2932 = u8 2 items=["0", "1", "2", "3", "4"] ("Axis Number")
            w2938 = "\r\n"
            n822 = call "RS232C_SetSpeed.vi"("Low Speed"=u32 100, "High Speed"=u16 10000 ("Acceleration Time"), "Acceleration Time"=u16 100, "Axis Number"=w2932, "Delimiter"=w2938, "VISAリソース名"=w2939, "Axis Count"=u8 2, "Range"=TRUE, "Main/Sub"=TRUE) -> ()  [unwired: 2 out]
          }
          frame #1 {
            w2947 = u8 2 items=["0", "1", "2", "3", "4"] ("Axis Number")
            n823 = Wait (ms)(milliseconds to wait=u32 500) -> ()  [unwired: 1 out]
            n824 = call "RS232C_Move.vi"("VISAリソース名"=w2946, "Axis Count"=u8 2, "Axis Number"=w2947, "Pulse Number"=w2941, "Direction"=w2942, "Delimiter"=w2945, "Main/Sub"=FALSE) -> ()  [unwired: 2 out]
          }
        }
        n825 = local read "um to move"() -> (w2798:u32)
        n826 = local read "scanning distance (um)"() -> (w2802:u32)
        n827 = Add(x=w2798, y=w2817) -> (x+y=w2827:u32)
        n828 = Subtract(x=w2802, y=w2827) -> (x-y=w2825:u32)
        n829 = Subtract(x=w2802, y=w2798) -> (x-y=w2815:u32)
        n830 = Greater?(x=w2799, y=1.0) -> (0:w2801:bool)
        n831 = case shown="True" w2826 {
          tunnel: w2825 -> [w2916 _]
          tunnel: [w2915 w2925] -> w2832
          tunnel: w2815 -> [_ w2926]
          tunnel: w2798 -> [w2914 w2924]
          tunnel: w2801 -> [w2911 w2923]
          tunnel: w2784 -> [w2913 w2922]
          tunnel: [w2912 w2921] -> w2797
          frame False {
            n832 = case shown="True" w2911 {
              tunnel: w2916 -> [w2917 w2920]
              tunnel: [w2917 w2920] -> w2915
              tunnel: w2914 -> [_ _]
              tunnel: w2913 -> [w2918 w2919]
              tunnel: [w2918 w2919] -> w2912
              frame False {
              }
              frame True {
              }
            }
          }
          frame True {
            n833 = case shown="False" w2923 {
              tunnel: w2926 -> [w2927 w2930]
              tunnel: [w2927 w2930] -> w2925
              tunnel: w2924 -> [_ _]
              tunnel: w2922 -> [w2928 w2929]
              tunnel: [w2928 w2929] -> w2921
              frame False {
              }
              frame True {
              }
            }
          }
        }
        "Last saved # 2" <- w2788
      }
      frame "4c acquirement" {
        w3040 = "%04d" ("format string")
        n834 = Increment(x=w3032) -> (x+1=w3031:i32)
        n835 = flat-sequence {
          tunnel: w3020 -> [w3143]
          tunnel: w3108 -> [w3152]
          tunnel: [w3152] -> w3098
          tunnel: [w3151] -> w3097
          tunnel: [w3143] -> w3044
          tunnel: [w3159] -> w3107
          tunnel: w3098 -> [w3159]
          tunnel: w3097 -> [w3158]
          tunnel: w3095 -> [_]
          tunnel: w3094 -> [_]
          tunnel: w3058 -> [w3155]
          tunnel: w3044 -> [w3154]
          frame #0 {
            w3145 = u8 2 items=["0", "1", "2", "3", "4"] ("Axis Number")
            w3151 = "\r\n"
            n836 = call "RS232C_SetSpeed.vi"("Low Speed"=u32 100, "High Speed"=u16 2000 ("Acceleration Time"), "Acceleration Time"=u16 100, "Axis Number"=w3145, "Delimiter"=w3151, "VISAリソース名"=w3152, "Axis Count"=u8 2, "Range"=TRUE, "Main/Sub"=TRUE) -> ()  [unwired: 2 out]
          }
          frame #1 {
            w3160 = u8 2 items=["0", "1", "2", "3", "4"] ("Axis Number")
            n837 = Not(x=w3154) -> (.not. x?=w3153:bool)
            n838 = Wait (ms)(milliseconds to wait=u32 500) -> ()  [unwired: 1 out]
            n839 = call "RS232C_Move.vi"("VISAリソース名"=w3159, "Axis Count"=u8 2, "Axis Number"=w3160, "Pulse Number"=w3155, "Direction"=w3153, "Delimiter"=w3158, "Main/Sub"=FALSE) -> ()  [unwired: 2 out]
          }
        }
        n840 = local read "Larvae until move"() -> (w3070:i32)
        n841 = local read "Larva # to move"() -> (w3053:i32)
        n842 = Increment(x=w3068) -> (x+1=w3067:i32)
        n843 = local write "Last saved #"(w3032) -> ()
        n844 = local read "# to measure"() -> (w3052:i32)
        n845 = local read "Continuous\nacquisition"() -> (w3054:bool)
        n846 = flat-sequence {
          tunnel: [w3220] -> w3096
          tunnel: [w3221] -> w3104
          tunnel: [w3222] -> w3103
          tunnel: [w3214] -> w3106
          tunnel: w3118 -> [w3220]
          tunnel: w3121 -> [w3221]
          tunnel: w3120 -> [w3222]
          frame #0 {
            w3214 = "\r\n"
            w3216 = u8 2 items=["0", "1", "2", "3", "4"] ("Axis Number")
            n847 = local read "Acquire speed (um/s)"() -> (w3212:u32)
            n848 = Wait (ms)(milliseconds to wait=u32 100) -> ()  [unwired: 1 out]
            n849 = call "RS232C_SetSpeed.vi"("Low Speed"=w3212, "High Speed"=w3212, "Acceleration Time"=u16 0, "Axis Number"=w3216, "Delimiter"=w3214, "VISAリソース名"=w3220, "Axis Count"=u8 2, "Range"=FALSE, "Main/Sub"=TRUE) -> ()  [unwired: 2 out]
          }
        }
        n850 = Insert Into Array(array=w3092, index=w3031, new element=w3091) -> (w3090:string[])
        n851 = Less?(x=w3052, y=w3031) -> (x < y?=w3109:bool)
        n852 = Greater?(x=w3070, y=w3053) -> (0:w3069:bool)
        n853 = Or(x=w3109, y=w3054) -> ()  [unwired: 1 out]
        n854 = flat-sequence {
          tunnel: w3077 -> [w3126]
          tunnel: w3078 -> [w3127]
          tunnel: w3080 -> [w3128]
          tunnel: w3082 -> [w3125]
          tunnel: [w3125] -> w3076
          tunnel: [w3128] -> w3075
          tunnel: [w3127] -> w3074
          tunnel: [w3126] -> w3073
          tunnel: [w3142] -> w3081
          tunnel: [w3141] -> w3079
          tunnel: w3076 -> [w3142]
          tunnel: w3075 -> [w3141]
          tunnel: w3074 -> [w3132]
          tunnel: w3073 -> [w3140]
          frame #0 {
            n855 = Wait (ms)(milliseconds to wait=u32 100) -> ()  [unwired: 1 out]
          }
          frame #1 {
            n856 = Path To String(path=w3132) -> (string=w3131:string)
            n857 = Strip Path(path=w3132) -> (name=w3136:string)  [unwired: 1 out]
            n858 = Concatenate Strings(w3131, ".dcimg" ("string")) -> (w3129:string)
            n859 = Concatenate Strings(w3136, ".dcimg" ("string")) -> (w3134:string)
            n860 = Concatenate Strings(w3140, "\\raw\\" ("string"), w3134) -> (w3138:string)
            n861 = String To Path(string=w3129) -> (path=w3133:path)
            n862 = String To Path(string=w3138) -> (path=w3137:path)
            n863 = Move(source path=w3133, 10:w3137) -> ()  [unwired: 3 in, 3 out]
          }
        }
        n864 = local read "Frames in memory 2"() -> (w3021:i32)
        n865 = local read "Movement direction"() -> (w3055:bool)
        n866 = Format Into String(format string=w3040, w3032) -> (resulting string=w3063:string)  [unwired: 2 in, 1 out]
        n867 = Format Into String(format string=w3040, w3037) -> (resulting string=w3039:string)  [unwired: 2 in, 1 out]
        n868 = Path To String(path=w3111) -> (string=w3077:string)
        n869 = Concatenate Strings(w3077, "\\temp\\" ("string"), "4c Base file name", "_" ("string"), w3063, "wavelength", w3039) -> (w3112:string)
        n870 = local read "um to move"() -> (w3024:u32)
        n871 = String To Path(string=w3112) -> (path=w3078:path)
        "Last saved file 4c" <- w3078
        n872 = call <userlib>:"tm_startrecorder_40.vi"("error in (no error)"=w3104, "frames"=w3021, "File"=w3078, "Handle in"=w3103) -> ("error out"=w3102:errorcluster, "Handle out"=w3101:u32)  [unwired: 6 in]
        n873 = call <userlib>:"tm_startcapture_40.vi"("error in (no error)"=w3102, "Handle in"=w3101) -> ("error out"=w3100:errorcluster, "Handle out"=w3099:u32)  [unwired: 8 in]
        n874 = while {
          tunnel: w3106 -> [w3165]
          tunnel: w3096 -> [w3175]
          tunnel: [w3174] -> w3108
          tunnel: [w3173] -> w3115
          tunnel: [w3171] -> w3020
          tunnel: w3055 -> [w3171]
          tunnel: [w3167] -> _
          tunnel: [w3166] -> _
          tunnel: [w3164] -> w3094
          stop <- w3172 stop-if-true
          # "Move to scan larva"
          n875 = flat-sequence {
            tunnel: w3171 -> [w3176]
            tunnel: w3175 -> [w3178]
            tunnel: [w3178] -> w3170
            tunnel: [w3176] -> w3169
            tunnel: [w3177] -> w3166
            tunnel: w3165 -> [_]
            tunnel: [w3176] -> _
            tunnel: [w3191] -> w3172
            tunnel: w3165 -> [w3186]
            tunnel: w3170 -> [w3190]
            tunnel: w3169 -> [w3185]
            tunnel: [w3190] -> w3168
            tunnel: [w3184] -> w3164
            tunnel: [w3195] -> w3174
            tunnel: w3168 -> [w3195]
            tunnel: [w3192] -> w3167
            frame #0 {
              n876 = for {
                N: 1 -> [_]
                tunnel: [w3181] -> w3177
                # "Delete"
                n877 = local read "Sub img mean"() -> (w3182:dbl)
                n878 = local read "Mean trigger"() -> (w3183:i32)
                n879 = Greater Or Equal?(x=w3182, y=w3183) -> (x >= y?=w3181:bool)
              }
              n880 = Wait (ms)(milliseconds to wait=u32 500) -> ()  [unwired: 1 out]
            }
            frame #1 {
              w3188 = u8 2 items=["0", "1", "2", "3", "4"] ("Axis Number")
              n881 = local read "um to move"() -> (w3184:u32)
              n882 = call "RS232C_Move.vi"("VISAリソース名"=w3190, "Axis Count"=u8 2, "Axis Number"=w3188, "Pulse Number"=w3184, "Direction"=w3185, "Delimiter"=w3186, "Main/Sub"=FALSE) -> ("OK Done"=w3191:bool)  [unwired: 1 out]
            }
            frame #2 {
              n883 = local read "Sub img mean"() -> (w3193:dbl)
              n884 = local read "Mean trigger"() -> (w3194:i32)
              n885 = Greater?(x=w3193, y=w3194) -> (0:w3192:bool)
            }
          }
          n886 = call <extravilib>:"Write.vi"("element"=w3172) -> ("channel"=w3173:T13)  [unwired: 1 out]
        }
        n887 = while {
          tunnel: w3099 -> [w3211]
          tunnel: w3100 -> [w3210]
          tunnel: [w3207] -> w3117
          tunnel: [w3206] -> w3116
          tunnel: w3115 -> [w3209]
          tunnel: w3105 -> [w3203]
          stop <- w3208 stop-if-true
          n888 = call <userlib>:"tm_waitnextframe_40.vi"("error in (no error)"=w3210, "Handle in"=w3211) -> ("error out"=w3206:errorcluster, "Frame Count"=w3202:i32, "Frame Index"=w3205:i32, "Handle out"=w3207:u32)  [unwired: 6 in]
          n889 = call <extravilib>:"Read.vi"("channel"=w3209) -> ("element"=w3208:bool)  [unwired: 1 in, 1 out]
          n890 = local write "Frame count"(w3202) -> ()
          n891 = Index Array(array=w3203, index=w3205) -> (element=w3204:T12)
          n892 = Multiply(x=2048, y=2048) -> (x*y=w3201:i32)
          n893 = call "IMAQ ImageToArray"("Image"=w3204) -> ("Image Pixels (U16)"=w3198:u16[][])  [unwired: 3 in, 4 out]
          n894 = local write "Obtained image"(w3198) -> ()
          n895 = Reshape Array(w3198, w3201) -> (w3197:u16[])
          n896 = call-poly <vilib>:"Mean.vi"("X"=w3197) -> ("mean"=w3196:dbl)  [unwired: 1 out]
          n897 = local write "Mean intensity\nof frame"(w3196) -> ()
        }
        n898 = local read "backwards pulses"() -> (w3025:i32)
        n899 = Greater?(x=0, y=w3041) -> (0:w3060:bool)
        n900 = local read "scanning distance (um)"() -> (w3022:u32)
        n901 = local read "Continuous\nacquisition"() -> (w3035:bool)
        n902 = Add(x=w3025, y=w3024) -> (x+y=w3023:u32)
        n903 = Subtract(x=w3023, y=w3022) -> (x-y=w3059:u32)
        n904 = case shown="False" w3060 {
          tunnel: w3059 -> [_ _]
          tunnel: [w3122 u32 0] -> w3058
          tunnel: w3024 -> [w3122 _]
          frame False {
          }
          frame True {
          }
        }
        n905 = case shown="True" w3035 {
          tunnel: [states."homing" states."4climbo"] -> w3110
          tunnel: w3069 -> [_ _]
          frame False {
          }
          frame True {
          }
        }
        n906 = call <userlib>:"tm_stopcapture_40.vi"("error in (no error)"=w3116, "Handle in"=w3117) -> ("error out"=w3113:errorcluster, "Handle out"=w3114:u32)  [unwired: 8 in]
        n907 = call <userlib>:"tm_stoprecorder_40.vi"("error in (no error)"=w3113, "Handle in"=w3114) -> ("error out"=w3080:errorcluster, "Handle out"=w3082:u32)  [unwired: 8 in]
      }
      frame "594" {
        w3225 = FALSE ("data")
        w3243 = TRUE ("data")
        w3244 = FALSE ("data")
        w3245 = FALSE ("data")
        w3246 = FALSE ("data")
        n908 = local write "647 i"(w3225) -> ()
        n909 = call-poly <vilib>:"DAQmx Write.vi"("task/channels in"=w3230, "data"=w3225) -> ()  [unwired: 11 in, 3 out]
        n910 = local write "405 i"(w3246) -> ()
        n911 = local read "4c direction"() -> (w3237:bool)
        n912 = call-poly <vilib>:"DAQmx Write.vi"("task/channels in"=w3254, "data"=w3246) -> ()  [unwired: 11 in, 3 out]
        n913 = local read "Continuous\nacquisition"() -> (w3248:bool)
        n914 = invoke class="StepperMotorChannel" method="SetMoveAbsolutePosition"(reference=w3250, "position"="594 filter") -> (reference out=w3255:refnum<k24>)  [unwired: 2 in, 3 out]
        n915 = local write "Movement direction"(w3237) -> ()
        n916 = case shown="True" w3248 {
          tunnel: [states."4cini" w3284] -> w3247
          frame False {
          }
          frame True {
            n917 = local read "4c"() -> (w3283:bool)
            n918 = case shown="True" w3283 {
              tunnel: [states."Acquire" w3288] -> w3284
              frame False {
                n919 = local write "594 i"(FALSE ("594 i")) -> ()
              }
              frame True {
                n920 = case shown="True" "594?" {
                  tunnel: [states."4climbo" states."4c acquirement"] -> w3288
                  frame False {
                  }
                  frame True {
                  }
                }
              }
            }
          }
        }
        n921 = local write "488 i"(w3245) -> ()
        n922 = call-poly <vilib>:"DAQmx Write.vi"("task/channels in"=w3253, "data"=w3245) -> ()  [unwired: 11 in, 3 out]
        n923 = invoke class="StepperMotorChannel" method="MoveAbsolute"(reference=w3255, "waitTimeout"=1000) -> (reference out=w3249:refnum<k24>)  [unwired: 2 in, 3 out]
        n924 = local write "532 i"(w3244) -> ()
        n925 = call-poly <vilib>:"DAQmx Write.vi"("task/channels in"=w3252, "data"=w3244) -> ()  [unwired: 11 in, 3 out]
        n926 = local write "wavelength"("_594" ("wavelength")) -> ()
        n927 = local write "594 i"(w3243) -> ()
        n928 = call-poly <vilib>:"DAQmx Write.vi"("task/channels in"=w3251, "data"=w3243) -> ()  [unwired: 11 in, 3 out]
      }
      frame "647" {
        w3294 = TRUE ("data")
        w3311 = FALSE ("data")
        w3312 = FALSE ("data")
        w3313 = FALSE ("data")
        w3314 = FALSE ("data")
        n929 = invoke class="StepperMotorChannel" method="SetMoveAbsolutePosition"(reference=w3318, "position"="647 filter") -> (reference out=w3323:refnum<k24>)  [unwired: 2 in, 3 out]
        n930 = local write "405 i"(w3314) -> ()
        n931 = call-poly <vilib>:"DAQmx Write.vi"("task/channels in"=w3322, "data"=w3314) -> ()  [unwired: 11 in, 3 out]
        n932 = local read "Continuous\nacquisition"() -> (w3316:bool)
        n933 = local write "wavelength"("_647" ("wavelength")) -> ()
        n934 = local write "488 i"(w3313) -> ()
        n935 = call-poly <vilib>:"DAQmx Write.vi"("task/channels in"=w3321, "data"=w3313) -> ()  [unwired: 11 in, 3 out]
        n936 = case shown="False" w3316 {
          tunnel: [states."4cini" w3352] -> w3315
          frame False {
          }
          frame True {
            n937 = local read "4c"() -> (w3351:bool)
            n938 = case shown="True" w3351 {
              tunnel: [states."Acquire" w3356] -> w3352
              frame False {
                n939 = local write "647 i"(FALSE ("data")) -> ()
              }
              frame True {
                n940 = case shown="True" "647?" {
                  tunnel: [states."4climbo" states."4c acquirement"] -> w3356
                  frame False {
                  }
                  frame True {
                  }
                }
              }
            }
          }
        }
        n941 = invoke class="StepperMotorChannel" method="MoveAbsolute"(reference=w3323, "waitTimeout"=1000) -> (reference out=w3317:refnum<k24>)  [unwired: 2 in, 3 out]
        n942 = call-poly <vilib>:"DAQmx Write.vi"("task/channels in"=w3320, "data"=w3312) -> ()  [unwired: 11 in, 3 out]
        n943 = local write "532 i"(w3312) -> ()
        n944 = local read "4c direction"() -> (w3306:bool)
        n945 = local write "594 i"(w3311) -> ()
        n946 = call-poly <vilib>:"DAQmx Write.vi"("task/channels in"=w3319, "data"=w3311) -> ()  [unwired: 11 in, 3 out]
        n947 = local write "Movement direction"(w3306) -> ()
        n948 = local write "647 i"(w3294) -> ()
        n949 = call-poly <vilib>:"DAQmx Write.vi"("task/channels in"=w3299, "data"=w3294) -> ()  [unwired: 11 in, 3 out]
      }
      frame "532" {
        w3361 = FALSE ("data")
        w3382 = FALSE ("data")
        w3381 = TRUE ("data")
        w3380 = FALSE ("data")
        w3379 = FALSE ("data")
        n950 = local write "488 i"(w3380) -> ()
        n951 = local write "405 i"(w3379) -> ()
        n952 = call-poly <vilib>:"DAQmx Write.vi"("task/channels in"=w3389, "data"=w3380) -> ()  [unwired: 11 in, 3 out]
        n953 = invoke class="StepperMotorChannel" method="SetMoveAbsolutePosition"(reference=w3386, "position"="532 filter") -> (reference out=w3391:refnum<k24>)  [unwired: 2 in, 3 out]
        n954 = call-poly <vilib>:"DAQmx Write.vi"("task/channels in"=w3390, "data"=w3379) -> ()  [unwired: 11 in, 3 out]
        n955 = local write "647 i"(w3361) -> ()
        n956 = local read "Continuous\nacquisition"() -> (w3384:bool)
        n957 = call-poly <vilib>:"DAQmx Write.vi"("task/channels in"=w3362, "data"=w3361) -> ()  [unwired: 11 in, 3 out]
        n958 = case shown="True" w3384 {
          tunnel: [states."4cini" w3420] -> w3383
          frame False {
          }
          frame True {
            n959 = local read "4c"() -> (w3419:bool)
            n960 = case shown="False" w3419 {
              tunnel: [states."Acquire" w3424] -> w3420
              frame False {
                n961 = local write "532 i"(FALSE ("data")) -> ()
              }
              frame True {
                n962 = case shown="True" "532?" {
                  tunnel: [states."4climbo" states."4c acquirement"] -> w3424
                  frame False {
                  }
                  frame True {
                  }
                }
              }
            }
          }
        }
        n963 = invoke class="StepperMotorChannel" method="MoveAbsolute"(reference=w3391, "waitTimeout"=2000) -> (reference out=w3385:refnum<k24>)  [unwired: 2 in, 3 out]
        n964 = local write "532 i"(w3381) -> ()
        n965 = call-poly <vilib>:"DAQmx Write.vi"("task/channels in"=w3388, "data"=w3381) -> ()  [unwired: 11 in, 3 out]
        n966 = local read "4c direction"() -> (w3373:bool)
        n967 = local write "594 i"(w3382) -> ()
        n968 = call-poly <vilib>:"DAQmx Write.vi"("task/channels in"=w3387, "data"=w3382) -> ()  [unwired: 11 in, 3 out]
        n969 = local write "Movement direction"(w3373) -> ()
        n970 = local write "wavelength"("_532" ("wavelength")) -> ()
      }
      frame "4cini" {
        n971 = Increment(x=w3444) -> (x+1=w3443:i32)
        n972 = local read "position"() -> (w3441:dbl)
        n973 = invoke class="StepperMotorChannel" method="SetMoveAbsolutePosition"(reference=w3456, "position"=w3441) -> (reference out=w3461:refnum<k24>)  [unwired: 2 in, 3 out]
        n974 = local read "405"() -> (w3437:bool)
        n975 = local write "405 i"(w3437) -> ()
        n976 = local read "647"() -> (w3429:bool)
        n977 = call-poly <vilib>:"DAQmx Write.vi"("task/channels in"=w3460, "data"=w3437) -> ()  [unwired: 11 in, 3 out]
        n978 = local read "488"() -> (w3438:bool)
        n979 = local write "488 i"(w3438) -> ()
        n980 = call-poly <vilib>:"DAQmx Write.vi"("task/channels in"=w3434, "data"=w3429) -> ()  [unwired: 11 in, 3 out]
        n981 = call-poly <vilib>:"DAQmx Write.vi"("task/channels in"=w3459, "data"=w3438) -> ()  [unwired: 11 in, 3 out]
        n982 = invoke class="StepperMotorChannel" method="MoveAbsolute"(reference=w3461, "waitTimeout"=2000) -> (reference out=w3455:refnum<k24>)  [unwired: 2 in, 3 out]
        n983 = local read "594"() -> (w3440:bool)
        n984 = local read "Continuous\nacquisition"() -> (w3454:bool)
        n985 = local write "594 i"(w3440) -> ()
        n986 = call-poly <vilib>:"DAQmx Write.vi"("task/channels in"=w3457, "data"=w3440) -> ()  [unwired: 11 in, 3 out]
        n987 = case shown="True" w3454 {
          tunnel: [states."homing" states."homing"] -> w3453
          frame False {
          }
          frame True {
          }
        }
        n988 = local read "532"() -> (w3439:bool)
        n989 = local write "532 i"(w3439) -> ()
        n990 = call-poly <vilib>:"DAQmx Write.vi"("task/channels in"=w3458, "data"=w3439) -> ()  [unwired: 11 in, 3 out]
        n991 = local write "wavelength"("532" ("wavelength")) -> ()
        n992 = local write "Movement direction"(TRUE ("Movement direction")) -> ()
      }
      frame "488" {
        w3491 = FALSE ("data")
        w3510 = FALSE ("data")
        w3511 = FALSE ("data")
        w3512 = TRUE ("data")
        w3513 = FALSE ("data")
        n993 = invoke class="StepperMotorChannel" method="SetMoveAbsolutePosition"(reference=w3517, "position"="488 filter") -> (reference out=w3522:refnum<k24>)  [unwired: 2 in, 3 out]
        n994 = local write "405 i"(w3513) -> ()
        n995 = call-poly <vilib>:"DAQmx Write.vi"("task/channels in"=w3521, "data"=w3513) -> ()  [unwired: 11 in, 3 out]
        n996 = Wait (ms)(milliseconds to wait=u32 2000) -> ()  [unwired: 1 out]
        n997 = local write "488 i"(w3512) -> ()
        n998 = call-poly <vilib>:"DAQmx Write.vi"("task/channels in"=w3520, "data"=w3512) -> ()  [unwired: 11 in, 3 out]
        n999 = invoke class="StepperMotorChannel" method="MoveAbsolute"(reference=w3522, "waitTimeout"=1000) -> (reference out=w3516:refnum<k24>)  [unwired: 2 in, 3 out]
        n1000 = local write "532 i"(w3511) -> ()
        n1001 = call-poly <vilib>:"DAQmx Write.vi"("task/channels in"=w3519, "data"=w3511) -> ()  [unwired: 11 in, 3 out]
        n1002 = local write "594 i"(w3510) -> ()
        n1003 = local read "Continuous\nacquisition"() -> (w3515:bool)
        n1004 = call-poly <vilib>:"DAQmx Write.vi"("task/channels in"=w3518, "data"=w3510) -> ()  [unwired: 11 in, 3 out]
        n1005 = local write "wavelength"("_488" ("wavelength")) -> ()
        n1006 = local read "4c direction"() -> (w3503:bool)
        n1007 = local write "647 i"(w3491) -> ()
        n1008 = local write "Movement direction"(w3503) -> ()
        n1009 = call-poly <vilib>:"DAQmx Write.vi"("task/channels in"=w3492, "data"=w3491) -> ()  [unwired: 11 in, 3 out]
        n1010 = case shown="True" w3515 {
          tunnel: [states."4cini" w3551] -> w3514
          frame False {
          }
          frame True {
            n1011 = local read "4c"() -> (w3550:bool)
            n1012 = case shown="True" w3550 {
              tunnel: [states."Acquire" w3555] -> w3551
              frame False {
                n1013 = local write "488 i"(FALSE ("data")) -> ()
              }
              frame True {
                n1014 = case shown="True" "488?" {
                  tunnel: [states."4climbo" states."4c acquirement"] -> w3555
                  frame False {
                  }
                  frame True {
                  }
                }
              }
            }
          }
        }
      }
      frame "405" {
        w3560 = FALSE ("data")
        w3578 = FALSE ("data")
        w3579 = FALSE ("data")
        w3580 = FALSE ("data")
        w3581 = TRUE ("data")
        n1015 = invoke class="StepperMotorChannel" method="SetMoveAbsolutePosition"(reference=w3585, "position"="405 filter") -> (reference out=w3590:refnum<k24>)  [unwired: 2 in, 3 out]
        n1016 = local write "647 i"(w3560) -> ()
        n1017 = call-poly <vilib>:"DAQmx Write.vi"("task/channels in"=w3589, "data"=w3581) -> ()  [unwired: 11 in, 3 out]
        n1018 = local write "405 i"(w3581) -> ()
        n1019 = call-poly <vilib>:"DAQmx Write.vi"("task/channels in"=w3561, "data"=w3560) -> ()  [unwired: 11 in, 3 out]
        n1020 = local read "Continuous\nacquisition"() -> (w3583:bool)
        n1021 = invoke class="StepperMotorChannel" method="MoveAbsolute"(reference=w3590, "waitTimeout"=2000) -> (reference out=w3584:refnum<k24>)  [unwired: 2 in, 3 out]
        n1022 = local write "488 i"(w3580) -> ()
        n1023 = call-poly <vilib>:"DAQmx Write.vi"("task/channels in"=w3588, "data"=w3580) -> ()  [unwired: 11 in, 3 out]
        n1024 = case shown="True" w3583 {
          tunnel: [states."auto imaging" w3619] -> w3582
          frame False {
          }
          frame True {
            n1025 = local read "4c"() -> (w3618:bool)
            n1026 = case shown="False" w3618 {
              tunnel: [states."Acquire" w3623] -> w3619
              frame False {
                n1027 = local write "405 i"(FALSE ("data")) -> ()
              }
              frame True {
                n1028 = case shown="False" "405?" {
                  tunnel: [states."4climbo" states."4c acquirement"] -> w3623
                  frame False {
                  }
                  frame True {
                  }
                }
              }
            }
          }
        }
        n1029 = local write "532 i"(w3579) -> ()
        n1030 = call-poly <vilib>:"DAQmx Write.vi"("task/channels in"=w3587, "data"=w3579) -> ()  [unwired: 11 in, 3 out]
        n1031 = local write "wavelength"("_405" ("wavelength")) -> ()
        n1032 = local write "594 i"(w3578) -> ()
        n1033 = local read "4c direction"() -> (w3572:bool)
        n1034 = call-poly <vilib>:"DAQmx Write.vi"("task/channels in"=w3586, "data"=w3578) -> ()  [unwired: 11 in, 3 out]
        n1035 = local write "Movement direction"(w3572) -> ()
      }
      frame "405_r" {
        w3628 = FALSE ("data")
        n1036 = invoke class="StepperMotorChannel" method="SetMoveAbsolutePosition"(reference=w3653, "position"=0.16 ("405 filter 2")) -> (reference out=w3658:refnum<k24>)  [unwired: 2 in, 3 out]
        n1037 = local write "647 i"(w3628) -> ()
        n1038 = local write "wavelength"("_405" ("wavelength")) -> ()
        n1039 = local read "4c direction"() -> (w3640:bool)
        n1040 = call-poly <vilib>:"DAQmx Write.vi"("task/channels in"=w3629, "data"=w3628) -> ()  [unwired: 11 in, 3 out]
        n1041 = call-poly <vilib>:"DAQmx Write.vi"("task/channels in"=w3657, "data"=TRUE) -> ()  [unwired: 11 in, 3 out]
        n1042 = local write "Movement direction"(w3640) -> ()
        n1043 = local read "Continuous\nacquisition"() -> (w3651:bool)
        n1044 = invoke class="StepperMotorChannel" method="MoveAbsolute"(reference=w3658, "waitTimeout"=2000) -> (reference out=w3652:refnum<k24>)  [unwired: 2 in, 3 out]
        n1045 = call-poly <vilib>:"DAQmx Write.vi"("task/channels in"=w3656, "data"=FALSE) -> ()  [unwired: 11 in, 3 out]
        n1046 = case shown="False" w3651 {
          tunnel: [states."auto imaging" states."auto imaging"] -> w3650
          frame False {
          }
          frame True {
            n1047 = local write "405 i"(FALSE ("405 i")) -> ()
          }
        }
        n1048 = call-poly <vilib>:"DAQmx Write.vi"("task/channels in"=w3655, "data"=FALSE) -> ()  [unwired: 11 in, 3 out]
        n1049 = call-poly <vilib>:"DAQmx Write.vi"("task/channels in"=w3654, "data"=FALSE) -> ()  [unwired: 11 in, 3 out]
      }
      frame "4climbo" {
        n1050 = local read "4c"() -> (w3688:bool)
        n1051 = case shown="False" w3688 {
          tunnel: [w3738 w3768] -> w3701
          tunnel: w3698 -> [_ _]
          tunnel: w3697 -> [_ _]
          tunnel: w3696 -> [_ _]
          tunnel: w3695 -> [_ _]
          frame False {
            n1052 = local read "405 2"() -> (w3757:bool)
            n1053 = local read "594  2"() -> (w3754:bool)
            n1054 = local read "532  2"() -> (w3755:bool)
            n1055 = local read "647 2"() -> (w3736:bool)
            n1056 = local read "488 2"() -> (w3756:bool)
            n1057 = Boolean To (0,1)(Boolean=w3757) -> (0, 1=w3752:i16)
            n1058 = Boolean To (0,1)(Boolean=w3756) -> (0, 1=w3750:i16)
            n1059 = Boolean To (0,1)(Boolean=w3755) -> (0, 1=w3748:i16)
            n1060 = Boolean To (0,1)(Boolean=w3754) -> (0, 1=w3746:i16)
            n1061 = Boolean To (0,1)(Boolean=w3736) -> (0, 1=w3735:i16)
            n1062 = Initialize Array(0.0 ("element"), 5 ("dimension size")) -> (w3743:dbl[])
            n1063 = Replace Array Subset(array=w3743, new element #1=w3752, index #1=0 ("index"), new element #2=w3750, index #2=1 ("index"), new element #3=w3748, index #3=2 ("index"), new element #4=w3746, index #4=3 ("index"), new element #5=w3735, index #5=4 ("index")) -> (w3742:dbl[])
            n1064 = Search 1D Array(1D array=w3742, element=1.0, start index (0)=0) -> (index of element=w3739:i32)
            n1065 = case shown="1" w3739 {
              tunnel: [states."405" states."532" states."594" states."647" states."Chilling" states."488"] -> w3738
              frame 0 {
              }
              frame 2 {
              }
              frame 3 {
              }
              frame 4 {
              }
              frame 5, Default {
              }
              frame 1 {
              }
            }
          }
          frame True {
            n1066 = local read "647 i"() -> (w3766:bool)
            n1067 = local read "488 i"() -> (w3770:bool)
            n1068 = local read "594 i"() -> (w3771:bool)
            n1069 = local read "532 i"() -> (w3769:bool)
            n1070 = local read "405 i"() -> (w3772:bool)
            n1071 = Boolean To (0,1)(Boolean=w3772) -> (0, 1=w3786:i16)
            n1072 = Boolean To (0,1)(Boolean=w3770) -> (0, 1=w3784:i16)
            n1073 = Boolean To (0,1)(Boolean=w3769) -> (0, 1=w3783:i16)
            n1074 = Boolean To (0,1)(Boolean=w3771) -> (0, 1=w3782:i16)
            n1075 = Boolean To (0,1)(Boolean=w3766) -> (0, 1=w3764:i16)
            n1076 = Initialize Array(0.0 ("element"), 5 ("dimension size")) -> (w3779:dbl[])
            n1077 = Replace Array Subset(array=w3779, new element #1=w3786, index #1=0 ("index"), new element #2=w3784, index #2=1 ("index"), new element #3=w3783, index #3=2 ("index"), new element #4=w3782, index #4=3 ("index"), new element #5=w3764, index #5=4 ("index")) -> (w3778:dbl[])
            n1078 = Search 1D Array(1D array=w3778, element=1.0, start index (0)=0) -> (index of element=w3767:i32)
            n1079 = case shown="0" w3767 {
              tunnel: [states."488" states."594" states."647" states."homing" states."4cini" states."532"] -> w3768
              frame 0 {
              }
              frame 2 {
              }
              frame 3 {
              }
              frame 4 {
              }
              frame 5, Default {
              }
              frame 1 {
              }
            }
          }
        }
      }
      frame "save" {
        n1080 = Increment(x=w3815) -> (x+1=w3814:i32)
        "Last saved file number 4" <- w3814
        n1081 = Insert Into Array(array=w3842, index=w3814, new element=w3841) -> (w3840:string[])
        n1082 = Path To String(path=w3861) -> (string=w3833:string)
        n1083 = local read "Frames in memory 2"() -> (w3793:i32)
        n1084 = flat-sequence {
          tunnel: [w3948] -> w3846
          tunnel: [w3949] -> w3852
          tunnel: [w3950] -> w3851
          tunnel: [w3942] -> w3854
          tunnel: w3868 -> [w3948]
          tunnel: w3871 -> [w3949]
          tunnel: w3870 -> [w3950]
          frame #0 {
            w3942 = "\r\n"
            w3944 = u8 2 items=["0", "1", "2", "3", "4"] ("Axis Number")
            n1085 = local read "Acquire speed (um/s)"() -> (w3940:u32)
            n1086 = Wait (ms)(milliseconds to wait=u32 200) -> ()  [unwired: 1 out]
            n1087 = call "RS232C_SetSpeed.vi"("Low Speed"=w3940, "High Speed"=w3940, "Acceleration Time"=u16 0, "Axis Number"=w3944, "Delimiter"=w3942, "VISAリソース名"=w3948, "Axis Count"=u8 2, "Range"="High speed?", "Main/Sub"=TRUE) -> ()  [unwired: 2 out]
          }
        }
        n1088 = local read "# to measure"() -> (w3824:i32)
        n1089 = Number To Decimal String(number=w3815, width (-)=i16 3) -> (decimal integer string=w3822:string)
        n1090 = Concatenate Strings(w3833, w3823, w3822) -> (w3862:string)
        n1091 = String To Path(string=w3862) -> (path=w3834:path)
        n1092 = local read "Last saved file number 4"() -> (w3830:i32)
        n1093 = Less?(x=w3824, y=w3814) -> (x < y?=w3858:bool)
        n1094 = call <userlib>:"tm_startrecorder_40.vi"("error in (no error)"=w3852, "frames"=w3793, "File"=w3834, "Handle in"=w3851) -> ("error out"=w3850:errorcluster, "Handle out"=w3849:u32)  [unwired: 6 in]
        n1095 = local read "Continuous\nacquisition"() -> (w3819:bool)
        n1096 = Or(x=w3858, y=w3819) -> (x .or. y?=w3818:bool)
        n1097 = call <userlib>:"tm_startcapture_40.vi"("error in (no error)"=w3850, "Handle in"=w3849) -> ("error out"=w3848:errorcluster, "Handle out"=w3847:u32)  [unwired: 8 in]
        n1098 = local read "Movement direction"() -> (w3825:bool)
        n1099 = Greater?(x=w3830, y=100) -> (0:w3828:bool)
        n1100 = case shown="True" w3818 {
          tunnel: [states."Chilling" w3894] -> w3859
          tunnel: w3828 -> [_ w3893]
          frame False {
          }
          frame True {
            n1101 = case shown="False" w3893 {
              tunnel: [states."antic\n" states."auto imaging"] -> w3894
              frame False {
              }
              frame True {
              }
            }
          }
        }
        n1102 = while {
          tunnel: w3854 -> [w3898]
          tunnel: w3846 -> [w3905]
          tunnel: [w3904] -> w3857
          tunnel: [w3903] -> w3865
          tunnel: [w3901] -> w3855
          tunnel: w3825 -> [w3901]
          tunnel: [w3900] -> _
          tunnel: [w3899] -> _
          tunnel: [w3897] -> w3844
          stop <- w3902 stop-if-true
          # "Move to scan larva"
          n1103 = stacked-sequence {
            seq-local: [w3908 _ _] -> [_ w3920 _]
            seq-local: [w3907 _ _] -> [_ w3915 _]
            seq-local: [_ w3920 _] -> [_ _ w3925]
            tunnel: w3905 -> [w3908 _ _]
            tunnel: w3901 -> [w3907 _ _]
            tunnel: [w3906 _ _] -> w3899
            tunnel: w3898 -> [_ _ _]
            tunnel: [_ w3921 _] -> w3902
            tunnel: w3898 -> [_ w3916 _]
            tunnel: [_ w3914 _] -> w3897
            tunnel: [_ _ w3925] -> w3904
            tunnel: [_ _ w3922] -> w3900
            frame #0 {
              n1104 = for {
                N: 1 -> [_]
                tunnel: [w3911] -> w3906
                n1105 = local read "Sub img mean"() -> (w3912:dbl)
                n1106 = local read "Mean trigger"() -> (w3913:i32)
                n1107 = Greater Or Equal?(x=w3912, y=w3913) -> (x >= y?=w3911:bool)
              }
              n1108 = Wait (ms)(milliseconds to wait=u32 500) -> ()  [unwired: 1 out]
            }
            frame #1 {
              w3918 = u8 2 items=["0", "1", "2", "3", "4"] ("Axis Number")
              # "Extra scan"
              n1109 = local read "um to move"() -> (w3914:u32)
              n1110 = call "RS232C_Move.vi"("VISAリソース名"=w3920, "Axis Count"=u8 2, "Axis Number"=w3918, "Pulse Number"=w3914, "Direction"=w3915, "Delimiter"=w3916, "Main/Sub"=FALSE) -> ("OK Done"=w3921:bool)  [unwired: 1 out]
            }
            frame #2 {
              n1111 = local read "Sub img mean"() -> (w3923:dbl)
              n1112 = local read "Mean trigger"() -> (w3924:i32)
              n1113 = Greater?(x=w3923, y=w3924) -> (0:w3922:bool)
            }
          }
          n1114 = call <extravilib>:"Write.vi"("element"=w3902) -> ("channel"=w3903:T13)  [unwired: 1 out]
        }
        n1115 = while {
          tunnel: w3847 -> [w3939]
          tunnel: w3848 -> [w3938]
          tunnel: [w3935] -> w3867
          tunnel: [w3934] -> w3866
          tunnel: w3865 -> [w3937]
          tunnel: w3853 -> [w3931]
          stop <- w3936 stop-if-true
          # "Camera streaming during acquisition"
          n1116 = call <userlib>:"tm_waitnextframe_40.vi"("error in (no error)"=w3938, "Handle in"=w3939) -> ("error out"=w3934:errorcluster, "Frame Count"=w3930:i32, "Frame Index"=w3933:i32, "Handle out"=w3935:u32)  [unwired: 6 in]
          n1117 = call <extravilib>:"Read.vi"("channel"=w3937) -> ("element"=w3936:bool)  [unwired: 1 in, 1 out]
          n1118 = local write "Frame count"(w3930) -> ()
          n1119 = Index Array(array=w3931, index=w3933) -> (element=w3932:T12)
          n1120 = call "IMAQ ImageToArray"("Image"=w3932) -> ("Image Pixels (U16)"=w3928:u16[][])  [unwired: 3 in, 4 out]
          n1121 = local write "Obtained image"(w3928) -> ()
          n1122 = Reshape Array(w3928, 4194304 ("dimension size")) -> (w3927:u16[])
          n1123 = call-poly <vilib>:"Mean.vi"("X"=w3927) -> ("mean"=w3926:dbl)  [unwired: 1 out]
          n1124 = local write "Mean intensity\nof frame"(w3926) -> ()
        }
        n1125 = stacked-sequence {
          seq-local: [w3879 _] -> [_ w3889]
          seq-local: [w3880 _] -> [_ w3882]
          seq-local: [w3878 _] -> [_ w3888]
          tunnel: w3857 -> [w3879 _]
          tunnel: w3855 -> [w3880 _]
          tunnel: [_ w3889] -> w3856
          tunnel: w3845 -> [_ w3885]
          tunnel: w3844 -> [_ w3883]
          frame #0 {
            w3872 = u8 2 items=["0", "1", "2", "3", "4"] ("Axis Number")
            w3874 = u16 3000 ("Acceleration Time")
            w3878 = "\r\n"
            n1126 = call "RS232C_SetSpeed.vi"("Low Speed"=w3874, "High Speed"=w3874, "Acceleration Time"=u16 0, "Axis Number"=w3872, "Delimiter"=w3878, "VISAリソース名"=w3879, "Axis Count"=u8 2, "Range"=TRUE, "Main/Sub"=TRUE) -> ()  [unwired: 2 out]
          }
          frame #1 {
            w3890 = u8 2 items=["0", "1", "2", "3", "4"] ("Axis Number")
            n1127 = Not(x=w3882) -> (.not. x?=w3881:bool)
            n1128 = Wait (ms)(milliseconds to wait=u32 500) -> ()  [unwired: 1 out]
            n1129 = Add(x=w3883, y=w3885) -> (x+y=w3884:u32)
            n1130 = call "RS232C_Move.vi"("VISAリソース名"=w3889, "Axis Count"=u8 2, "Axis Number"=w3890, "Pulse Number"=w3884, "Direction"=w3881, "Delimiter"=w3888, "Main/Sub"=FALSE) -> ()  [unwired: 2 out]
          }
        }
        n1131 = call <userlib>:"tm_stopcapture_40.vi"("error in (no error)"=w3866, "Handle in"=w3867) -> ("error out"=w3863:errorcluster, "Handle out"=w3864:u32)  [unwired: 8 in]
        n1132 = call <userlib>:"tm_stoprecorder_40.vi"("error in (no error)"=w3863, "Handle in"=w3864) -> ("error out"=w3826:errorcluster, "Handle out"=w3827:u32)  [unwired: 8 in]
      }
      frame "4000" {
        # "Set stage speed for acquisition"
        n1133 = Number To Decimal String(number=w3996, width (-)=i16 3) -> (decimal integer string=w4018:string)
        n1134 = flat-sequence {
          tunnel: [w4135] -> w4022
          tunnel: [w4136] -> w4031
          tunnel: [w4137] -> w4030
          tunnel: [w4129] -> w4033
          tunnel: w4053 -> [w4135]
          tunnel: w4056 -> [w4136]
          tunnel: w4055 -> [w4137]
          frame #0 {
            w4129 = "\r\n"
            w4131 = u8 2 items=["0", "1", "2", "3", "4"] ("Axis Number")
            n1135 = Wait (ms)(milliseconds to wait=u32 500) -> ()  [unwired: 1 out]
            n1136 = call "RS232C_SetSpeed.vi"("Low Speed"="Acquire speed 2 (um/s)", "High Speed"="Acquire speed 2 (um/s)", "Acceleration Time"=u16 0, "Axis Number"=w4131, "Delimiter"=w4129, "VISAリソース名"=w4135, "Axis Count"=u8 2, "Range"=TRUE, "Main/Sub"=FALSE) -> ("OK Done"=→"OK Done 4":bool)  [unwired: 1 out]
          }
        }
        n1137 = Add(x=1, y=w3996) -> (x+y=w3980:i32)
        n1138 = Initialize Array("", 1000 ("dimension size")) -> (w4010:string[])
        n1139 = Less?(x="Samples to measure 4000", y=w3980) -> (x < y?=w4041:bool)
        n1140 = Insert Into Array(array=w4010, index=w3980, new element=w4017) -> ()  [unwired: 1 out]
        n1141 = local read "Frames in memory 2"() -> (w3951:i32)
        n1142 = Path To String(path="Save base file name 4000") -> (string=w4047:string)
        n1143 = Or(x=w4041, y="EH speed 2") -> (x .or. y?=w4039:bool)
        n1144 = case shown="False" w4039 {
          tunnel: [states."Chilling" w4085] -> w4042
          tunnel: "calibration?" -> [_ w4084]
          frame False {
          }
          frame True {
            n1145 = case shown="True" w4084 {
              tunnel: [states."Acquire" states."homing"] -> w4085
              frame False {
              }
              frame True {
              }
            }
          }
        }
        n1146 = Concatenate Strings(w4047, w4018) -> (w4046:string)
        n1147 = String To Path(string=w4046) -> (path=w4003:path)
        "Last saved file 4000" <- w4003
        n1148 = local read "Movement direction"() -> (w3992:bool)
        n1149 = call <userlib>:"tm_startrecorder_40.vi"("error in (no error)"=w4031, "frames"=w3951, "File"=w4003, "Handle in"=w4030) -> ("error out"=w4029:errorcluster, "Handle out"=w4028:u32)  [unwired: 6 in]
        n1150 = Initialize Array(0.0 ("element"), 200 ("dimension size"), 2048 ("dimension size"), 2048 ("dimension size")) -> (w4007:dbl[][][])
        n1151 = call <userlib>:"tm_startcapture_40.vi"("error in (no error)"=w4029, "Handle in"=w4028) -> ("error out"=w4027:errorcluster, "Handle out"=w4026:u32)  [unwired: 8 in]
        n1152 = Initialize Array(0.0 ("element"), 1000 ("dimension size")) -> (w3981:dbl[])
        n1153 = while {
          tunnel: w4033 -> [w4089]
          tunnel: w4022 -> [w4097]
          tunnel: [w4096] -> w4038
          tunnel: [w4095] -> w4050
          tunnel: [w4093] -> w4036
          tunnel: w3992 -> [w4093]
          tunnel: [w4088] -> w4020
          stop <- w4094 stop-if-true
          # "Move to scan larva"
          n1154 = flat-sequence {
            tunnel: w4093 -> [w4098]
            tunnel: w4097 -> [w4099]
            tunnel: [w4099] -> w4092
            tunnel: [w4098] -> w4091
            tunnel: w4089 -> [_]
            tunnel: [w4108] -> w4094
            tunnel: w4089 -> [w4103]
            tunnel: w4092 -> [w4107]
            tunnel: w4091 -> [w4102]
            tunnel: [w4107] -> w4090
            tunnel: [w4101] -> w4088
            tunnel: [w4109] -> w4096
            tunnel: w4090 -> [w4109]
            frame #0 {
              n1155 = Wait (ms)(milliseconds to wait=u32 500) -> ()  [unwired: 1 out]
            }
            frame #1 {
              w4105 = u8 2 items=["0", "1", "2", "3", "4"] ("Axis Number")
              # "Extra scan"
              n1156 = local read "um to move"() -> (w4101:u32)
              n1157 = call "RS232C_Move.vi"("VISAリソース名"=w4107, "Axis Count"=u8 2, "Axis Number"=w4105, "Pulse Number"=w4101, "Direction"=w4102, "Delimiter"=w4103, "Main/Sub"=FALSE) -> ("OK Done"=w4108:bool)  [unwired: 1 out]
            }
            frame #2 {
            }
          }
          n1158 = call <extravilib>:"Write.vi"("element"=w4094) -> ("channel"=w4095:T13)  [unwired: 1 out]
        }
        n1159 = while {
          tunnel: w4026 -> [w4125]
          tunnel: w4027 -> [w4124]
          tunnel: [w4121] -> w4052
          tunnel: [w4120] -> w4051
          tunnel: w4050 -> [w4123]
          tunnel: w4032 -> [w4117]
          shift-right: [w4115] -> w4006
          shift-left: w4007 -> [w4116]
          stop <- w4122 stop-if-true
          n1160 = call <extravilib>:"Read.vi"("channel"=w4123) -> ("element"=w4122:bool)  [unwired: 1 in, 1 out]
          n1161 = call <userlib>:"tm_waitnextframe_40.vi"("error in (no error)"=w4124, "Handle in"=w4125) -> ("error out"=w4120:errorcluster, "Frame Count"=w4114:i32, "Frame Index"=w4119:i32, "Handle out"=w4121:u32)  [unwired: 6 in]
          n1162 = Index Array(array=w4117, index=w4119) -> (element=w4118:T12)
          n1163 = local write "Frame count"(w4114) -> ()
          n1164 = call "IMAQ ImageToArray"("Image"=w4118) -> ("Image Pixels (U16)"=w4112:u16[][])  [unwired: 3 in, 4 out]
          n1165 = local write "Obtained image"(w4112) -> ()
          n1166 = Reshape Array(w4112, 4194304 ("dimension size")) -> (w4113:u16[])
          n1167 = Replace Array Subset(array=w4116, new element=w4112, index (dim 0)=w4114) -> (w4115:dbl[][][])  [unwired: 2 in]
          n1168 = call-poly <vilib>:"Mean.vi"("X"=w4113) -> ("mean"=w4111:dbl)  [unwired: 1 out]
          n1169 = local write "Mean intensity\nof frame"(w4111) -> ()
        }
        n1170 = for {
          tunnel: w4006 -> [w4064] mode=indexing
          tunnel: [w4059] -> w3991 mode=indexing
          tunnel: [w4057] -> _ mode=indexing
          workers-P: _ -> [_]
          tunnel: [w4057] -> _ mode=indexing
          w4063 = 2048 ("dimension size")
          n1171 = Multiply(x=w4063, y=w4063) -> (x*y=w4062:i32)
          n1172 = Reshape Array(w4064, w4062) -> (w4061:dbl[])
          n1173 = call-poly <vilib>:"Mean.vi"("X"=w4061) -> ("mean"=w4057:dbl)  [unwired: 1 out]
          n1174 = Greater?(x=w4057, y="wave trigger") -> (0:w4060:bool)
          n1175 = Boolean To (0,1)(Boolean=w4060) -> (0, 1=w4059:i16)
        }
        n1176 = call-poly <vilib>:"Write Waveforms to File.vi"("waveform"=w3991, "file path (dialog if empty)"=w4003) -> ()  [unwired: 8 in, 2 out]
        n1177 = Reverse 1D Array(array=w3991) -> (reversed array=w4001:i16[])
        n1178 = Search 1D Array(1D array=w3991, element=i16 1) -> (index of element=w3990:i32)  [unwired: 1 in]
        n1179 = Search 1D Array(1D array=w4001, element=i16 1) -> (index of element=w3998:i32)  [unwired: 1 in]
        n1180 = Add(x=w3990, y=w3998) -> (x+y=w3999:i32)
        n1181 = Subtract(x=200, y=w3999) -> (x-y=w3989:i32)
        n1182 = Array Subset(array=w3981, index=w3990, length=w3989) -> (w3988:dbl[])
        n1183 = call-poly <vilib>:"Mean.vi"("X"=w3988) -> ("mean"=w3978:dbl)  [unwired: 1 out]
        n1184 = Insert Into Array(array=w3979, index=w3980, new element=w3978) -> (w3977:dbl[])
        n1185 = Insert Into Array(array=w3994, index=w3980, new element=w3989) -> (w3993:i16[])
        n1186 = flat-sequence {
          tunnel: w4036 -> [w4073]
          tunnel: w4038 -> [w4072]
          tunnel: [w4072] -> w4025
          tunnel: [w4073] -> w4024
          tunnel: [w4071] -> w4023
          tunnel: [w4080] -> w4037
          tunnel: w4025 -> [w4080]
          tunnel: w4024 -> [w4076]
          tunnel: w4023 -> [w4079]
          tunnel: w4020 -> [w4074]
          frame #0 {
            w4065 = u8 2 items=["0", "1", "2", "3", "4"] ("Axis Number")
            w4067 = u16 2000 ("Acceleration Time")
            w4071 = "\r\n"
            n1187 = call "RS232C_SetSpeed.vi"("Low Speed"=w4067, "High Speed"=w4067, "Acceleration Time"=u16 0, "Axis Number"=w4065, "Delimiter"=w4071, "VISAリソース名"=w4072, "Axis Count"=u8 2, "Range"=TRUE, "Main/Sub"=FALSE) -> ()  [unwired: 2 out]
          }
          frame #1 {
            w4081 = u8 2 items=["0", "1", "2", "3", "4"] ("Axis Number")
            n1188 = Not(x=w4076) -> (.not. x?=w4075:bool)
            n1189 = Wait (ms)(milliseconds to wait=u32 500) -> ()  [unwired: 1 out]
            n1190 = call "RS232C_Move.vi"("VISAリソース名"=w4080, "Axis Count"=u8 2, "Axis Number"=w4081, "Pulse Number"=w4074, "Direction"=w4075, "Delimiter"=w4079, "Main/Sub"=FALSE) -> ()  [unwired: 2 out]
          }
        }
        n1191 = local write "screening"(TRUE ("screening")) -> ()
        n1192 = call <userlib>:"tm_stopcapture_40.vi"("error in (no error)"=w4051, "Handle in"=w4052) -> ("error out"=w4048:errorcluster, "Handle out"=w4049:u32)  [unwired: 8 in]
        n1193 = call <vilib>:"High Resolution Relative Seconds.vi"() -> ("relative seconds"=w3958:dbl)
        n1194 = call <userlib>:"tm_stoprecorder_40.vi"("error in (no error)"=w4048, "Handle in"=w4049) -> ("error out"=w4034:errorcluster, "Handle out"=w4035:u32)  [unwired: 8 in]
      }
      frame "screening" {
        n1195 = case shown="False" "2000?" {
          tunnel: [w4197 w4198] -> w4155
          frame False {
            n1196 = local read "Last saved file 4000"() -> (w4197:path)
          }
          frame True {
            n1197 = local read "Last saved file 2000"() -> (w4202:path)
            n1198 = Path To String(path=w4202) -> (string=w4201:string)
            n1199 = Concatenate Strings(w4201, ".dcimg" ("string")) -> (w4199:string)
            n1200 = String To Path(string=w4199) -> (path=w4198:path)
          }
        }
        n1201 = case shown="\"MAX INTENSITY\"" "screening method" {
          tunnel: w4155 -> [w4208 w4242 w4280 w4320]
          tunnel: "Count threshold" -> [w4207 w4241 w4281 w4318]
          tunnel: [w4206 _ _ _] -> _
          tunnel: [w4205 w4240 _ _] -> _
          tunnel: [FALSE FALSE w4278 w4319] -> w4150
          frame "Pix count" {
            n1202 = for {
              N: 0 -> [_]
              tunnel: w4208 -> [w4218]
              tunnel: [w4209] -> w4205 mode=indexing
              tunnel: w4207 -> [w4215]
              tunnel: [w4212] -> w4206 mode=indexing
              n1203 = call <userlib>:"tm_opendcimgfile_40.vi"("Path"=w4218) -> ("error out"=w4220:errorcluster, "Total Frames"=w4210:i32, "File Handle"=w4221:u32)  [unwired: 8 in]
              n1204 = for {
                N: w4210 -> [_]
                tunnel: w4221 -> [w4233]
                tunnel: w4220 -> [w4232]
                tunnel: [w4231] -> w4219
                tunnel: [w4229] -> w4217
                tunnel: [w4226] -> w4216 mode=indexing
                tunnel: w4215 -> [w4224]
                i -> [w4230]
                n1205 = call <userlib>:"tm_getdcimgframe.vi"("error in (no error)"=w4232, "Frame Index"=w4230, "File Handle in"=w4233) -> ("error out"=w4231:errorcluster, "Data"=w4228:u16[][], "File Handle out"=w4229:u32)  [unwired: 5 in, 1 out]
                n1206 = for {
                  tunnel: w4228 -> [w4235] mode=indexing
                  tunnel: [w4236] -> w4227 mode=indexing
                  workers-P: 36 -> [_]
                  tunnel: w4224 -> [w4234]
                  n1207 = call <vilib>:"Threshold Detector.vi"("width"=1, "threshold"=w4234, "X"=w4235) -> ("count"=w4236:i32)  [unwired: 2 out]
                }
                n1208 = Add Array Elements(numeric array=w4227) -> (sum=w4226:i32)
              }
              n1209 = call <userlib>:"tm_closedcimgfile_40.vi"("error in (no error)"=w4219, "File Handle"=w4217) -> ()  [unwired: 9 in, 1 out]
              n1210 = Add Array Elements(numeric array=w4216) -> (sum=w4211:i32)
              n1211 = Divide(x=w4211, y=w4210) -> (x/y=w4209:dbl)
              n1212 = Greater?(x=w4209, y=9000 ("x")) -> (0:w4213:bool)
              n1213 = case shown="True" w4213 {
                tunnel: [1 ("index") 2 ("index")] -> w4212
                frame False {
                  # "PURE NON TUBBY"
                }
                frame True {
                  # "TUBBY"
                }
              }
            }
            n1214 = call <vilib>:"High Resolution Relative Seconds.vi"() -> ()  [unwired: 1 out]
          }
          frame "Average int" {
            n1215 = for {
              N: 0 -> [_]
              tunnel: w4242 -> [w4250]
              tunnel: [w4247] -> _ mode=indexing
              tunnel: [w4246] -> _ mode=indexing
              tunnel: [w4244] -> w4240 mode=indexing
              tunnel: w4241 -> [w4243]
              n1216 = call <userlib>:"tm_opendcimgfile_40.vi"("Path"=w4250) -> ("error out"=w4252:errorcluster, "Total Frames"=w4249:i32, "File Handle"=w4253:u32)  [unwired: 8 in]
              n1217 = for {
                N: w4249 -> [_]
                tunnel: w4253 -> [w4265]
                tunnel: w4252 -> [w4264]
                tunnel: [w4263] -> w4251
                tunnel: [w4261] -> w4248
                tunnel: [w4258] -> w4246 mode=indexing
                tunnel: [w4257] -> w4245 mode=indexing
                tunnel: w4243 -> [w4254]
                i -> [w4262]
                n1218 = call <userlib>:"tm_getdcimgframe.vi"("error in (no error)"=w4264, "Frame Index"=w4262, "File Handle in"=w4265) -> ("error out"=w4263:errorcluster, "Data"=w4260:u16[][], "File Handle out"=w4261:u32)  [unwired: 5 in, 1 out]
                n1219 = for {
                  tunnel: w4260 -> [w4271] mode=indexing
                  tunnel: [w4272] -> w4259 mode=indexing
                  workers-P: 36 -> [_]
                  tunnel: [w4269] -> w4255 mode=indexing
                  tunnel: w4254 -> [w4266]
                  n1220 = call <vilib>:"Threshold Detector.vi"("width"=1, "threshold"=w4266, "X"=w4271) -> ("count"=w4272:i32, "Indices"=w4270:i32[])  [unwired: 1 out]
                  n1221 = for {
                    tunnel: w4271 -> [w4276]
                    tunnel: w4270 -> [w4275] mode=indexing
                    tunnel: [w4274] -> w4268 mode=indexing
                    n1222 = Index Array(array=w4276, index=w4275) -> (element=w4274:u16)
                  }
                  n1223 = Array Size(array=w4268) -> (size(s)=→"size(s)":i32)
                  n1224 = call-poly <vilib>:"Mean.vi"("X"=w4268) -> ("mean"=w4269:dbl)  [unwired: 1 out]
                }
                n1225 = call-poly <vilib>:"Mean.vi"("X"=w4255) -> ("mean"=w4257:dbl)  [unwired: 1 out]
                "mean 5" <- w4257
                n1226 = Add Array Elements(numeric array=w4259) -> (sum=w4258:i32)
                "Frame 2" <- w4262
              }
              n1227 = call <userlib>:"tm_closedcimgfile_40.vi"("error in (no error)"=w4251, "File Handle"=w4248) -> ()  [unwired: 9 in, 1 out]
              n1228 = Add Array Elements(numeric array=w4246) -> (sum=w4247:i32)
              n1229 = call-poly <vilib>:"Mean.vi"("X"=w4245) -> ("mean"=w4244:dbl)  [unwired: 1 out]
              "mean 4" <- w4244
            }
            n1230 = call <vilib>:"High Resolution Relative Seconds.vi"() -> ()  [unwired: 1 out]
          }
          frame "MAX INTENSITY" {
            n1231 = call <userlib>:"tm_opendcimgfile_40.vi"("Path"=w4280) -> ("error out"=w4286:errorcluster, "Total Frames"=w4287:i32, "File Handle"=w4285:u32)  [unwired: 8 in]
            n1232 = for {
              N: w4287 -> [_]
              tunnel: w4285 -> [w4317]
              tunnel: w4286 -> [w4316]
              tunnel: [w4315] -> _
              tunnel: [w4311] -> w4292
              tunnel: w4281 -> [_]
              tunnel: [w4305] -> w4290 mode=indexing
              workers-P: _ -> [_]
              i -> [w4314]
              n1233 = Multiply(x=2048.0, y=2048.0) -> (x*y=w4303:dbl)
              n1234 = call <userlib>:"tm_getdcimgframe.vi"("error in (no error)"=w4316, "Frame Index"=w4314, "File Handle in"=w4317) -> ("error out"=w4315:errorcluster, "Data"=w4304:u16[][], "File Handle out"=w4311:u32)  [unwired: 5 in, 1 out]
              n1235 = Reshape Array(w4304, w4303) -> (w4302:u16[])
              n1236 = call "Sort 1D Array.vim"("unsorted array"=w4302) -> ("sorted array"=w4310:u16[])  [unwired: 10 in]
              n1237 = Reverse 1D Array(array=w4310) -> (reversed array=w4309:u16[])
              n1238 = Array Subset(array=w4309, index=0, length=5) -> (w4306:u16[])
              n1239 = call-poly <vilib>:"Mean.vi"("X"=w4306) -> ("mean"=w4305:dbl)  [unwired: 1 out]
              "Numeric 4" <- w4314
            }
            n1240 = call "Sort 1D Array.vim"("unsorted array"=w4290) -> ("sorted array"=w4291:dbl[])  [unwired: 10 in]
            n1241 = Reverse 1D Array(array=w4291) -> (reversed array=w4288:dbl[])
            n1242 = Array Subset(array=w4288, index=0, length=5) -> (w4289:dbl[])
            n1243 = call-poly <vilib>:"Mean.vi"("X"=w4289) -> ("mean"=w4279:dbl)  [unwired: 1 out]
            n1244 = Greater?(x="max intensity threshold", y=w4279) -> (0:w4278:bool)
            n1245 = case shown="True" w4278 {
              tunnel: [1 ("index") 2 ("index")] -> w4277
              tunnel: w4292 -> [w4295 w4300]
              tunnel: [w4295 w4300] -> w4293
              tunnel: [w4294 w4298] -> _
              frame False {
                # "PURE NON TUBBY"
                n1246 = Wait (ms)(milliseconds to wait=u32 5) -> ()  [unwired: 1 out]
                n1247 = call <vilib>:"High Resolution Relative Seconds.vi"() -> ("relative seconds"=w4294:dbl)
              }
              frame True {
                # "TUBBY"
                n1248 = Wait (ms)(milliseconds to wait=u32 5) -> ()  [unwired: 1 out]
                n1249 = call <vilib>:"High Resolution Relative Seconds.vi"() -> ("relative seconds"=w4298:dbl)
              }
            }
            "index" <- w4277
            n1250 = call <userlib>:"tm_closedcimgfile_40.vi"("File Handle"=w4293) -> ()  [unwired: 10 in, 1 out]
          }
          frame "morphology" {
            w4322 = 0 ("start index (0)")
            w4328 = i16 1 ("element")
            n1251 = call <userlib>:"tm_opendcimgfile_40.vi"("Path"=w4320) -> ("error out"=w4333:errorcluster, "Total Frames"=w4325:i32, "File Handle"=w4332:u32)  [unwired: 8 in]
            n1252 = for {
              N: w4325 -> [_]
              tunnel: w4332 -> [w4362]
              tunnel: w4333 -> [w4361]
              tunnel: [w4360] -> _
              tunnel: [w4356] -> w4334
              tunnel: w4318 -> [_]
              tunnel: [w4344] -> w4330 mode=indexing
              workers-P: 6 -> [_]
              i -> [w4359]
              n1253 = Multiply(x=2048.0, y=2048.0) -> (x*y=w4349:dbl)
              n1254 = call <userlib>:"tm_getdcimgframe.vi"("error in (no error)"=w4361, "Frame Index"=w4359, "File Handle in"=w4362) -> ("error out"=w4360:errorcluster, "Data"=w4350:u16[][], "File Handle out"=w4356:u32)  [unwired: 5 in, 1 out]
              n1255 = Reshape Array(w4350, w4349) -> (w4348:u16[])
              n1256 = call "Sort 1D Array.vim"("unsorted array"=w4348) -> ("sorted array"=w4355:u16[])  [unwired: 10 in]
              n1257 = Reverse 1D Array(array=w4355) -> (reversed array=w4354:u16[])
              n1258 = Array Subset(array=w4354, index=0, length=4194304) -> (w4351:u16[])
              n1259 = call-poly <vilib>:"Mean.vi"("X"=w4351) -> ("mean"=w4347:dbl)  [unwired: 1 out]
              n1260 = Greater?(x=w4347, y="Setting 2") -> (0:w4345:bool)
              n1261 = Boolean To (0,1)(Boolean=w4345) -> (0, 1=w4344:i16)
              "Numeric 8" <- w4359
            }
            n1262 = Reverse 1D Array(array=w4330) -> (reversed array=w4329:i16[])
            n1263 = Search 1D Array(1D array=w4330, element=w4328, start index (0)=w4322) -> (index of element=w4327:i32)
            n1264 = Search 1D Array(1D array=w4329, element=w4328, start index (0)=w4322) -> (index of element=w4326:i32)
            n1265 = Add(x=w4327, y=w4326) -> (x+y=w4324:i32)
            n1266 = Subtract(x=w4325, y=w4324) -> (x-y=w4323:i32)
            n1267 = Greater?(x="morphology\nthreshold", y=w4323) -> (0:w4319:bool)
            n1268 = case shown="False" w4319 {
              tunnel: [1 ("index") 2 ("index")] -> _
              tunnel: w4334 -> [w4337 w4342]
              tunnel: [w4337 w4342] -> w4335
              tunnel: [w4336 w4340] -> _
              frame False {
                # "PURE NON TUBBY"
                n1269 = Wait (ms)(milliseconds to wait=u32 5) -> ()  [unwired: 1 out]
                n1270 = call <vilib>:"High Resolution Relative Seconds.vi"() -> ("relative seconds"=w4336:dbl)
              }
              frame True {
                # "TUBBY"
                n1271 = Wait (ms)(milliseconds to wait=u32 5) -> ()  [unwired: 1 out]
                n1272 = call <vilib>:"High Resolution Relative Seconds.vi"() -> ("relative seconds"=w4340:dbl)
              }
            }
            n1273 = call <userlib>:"tm_closedcimgfile_40.vi"("File Handle"=w4335) -> ()  [unwired: 10 in, 1 out]
          }
        }
        n1274 = case shown="True" w4150 {
          tunnel: [states."Acquire" states."homing"] -> w4151
          tunnel: [w4188 w4195] -> _
          tunnel: [w4187 w4192] -> w4144
          frame False {
            n1275 = call <vilib>:"High Resolution Relative Seconds.vi"() -> ("relative seconds"=w4187:dbl)
            n1276 = Wait (ms)(milliseconds to wait=u32 500) -> ()  [unwired: 1 out]
            n1277 = call <vilib>:"High Resolution Relative Seconds.vi"() -> ("relative seconds"=w4188:dbl)
            n1278 = local write "screening"(FALSE ("screening 2")) -> ()
          }
          frame True {
            n1279 = call <vilib>:"High Resolution Relative Seconds.vi"() -> ("relative seconds"=w4192:dbl)
            n1280 = call <vilib>:"High Resolution Relative Seconds.vi"() -> ("relative seconds"=w4195:dbl)
            n1281 = Wait (ms)(milliseconds to wait=u32 500) -> ()  [unwired: 1 out]
            n1282 = local write "screening"(TRUE ("screening 2")) -> ()
          }
        }
        n1283 = Subtract(x=w4144, y=w4145) -> ()  [unwired: 1 out]
        "screening" <- FALSE ("screening 2")
      }
      frame "2000" {
        w4368 = i16 1 ("element")
        n1284 = local read "Movement direction"() -> (w4404:bool)
        n1285 = Initialize Array("", 1000 ("dimension size")) -> (w4417:string[])
        n1286 = Less?(x="Samples to measure 2000", y=w4369) -> (x < y?=w4453:bool)
        n1287 = Number To Decimal String(number=w4369, width (-)=i16 3) -> (decimal integer string=w4427:string)
        n1288 = Increment(x=w4369) -> (x+1=w4370:i32)
        n1289 = Or(x=w4453, y="EH speed 3") -> (x .or. y?=w4451:bool)
        n1290 = Insert Into Array(array=w4417, index=w4370, new element=w4426) -> ()  [unwired: 1 out]
        n1291 = while {
          tunnel: w4445 -> [w4504]
          tunnel: w4433 -> [w4514]
          tunnel: [w4513] -> w4450
          tunnel: [w4512] -> w4461
          tunnel: [w4510] -> w4448
          tunnel: w4404 -> [w4510]
          tunnel: [w4506] -> _
          tunnel: [w4505] -> w4430
          tunnel: [w4503] -> w4432
          stop <- w4511 stop-if-true
          # "Move to scan larva"
          n1292 = flat-sequence {
            tunnel: w4510 -> [w4516]
            tunnel: w4514 -> [w4517]
            tunnel: [w4517] -> w4509
            tunnel: [w4516] -> w4508
            tunnel: [w4515] -> w4505
            tunnel: w4504 -> [_]
            tunnel: [w4530] -> w4511
            tunnel: w4504 -> [w4525]
            tunnel: w4509 -> [w4529]
            tunnel: w4508 -> [w4524]
            tunnel: [w4529] -> w4507
            tunnel: [w4523] -> w4503
            tunnel: [w4534] -> w4513
            tunnel: w4507 -> [w4534]
            tunnel: [w4531] -> w4506
            frame #0 {
              n1293 = for {
                N: 1 -> [_]
                tunnel: [w4520] -> w4515
                n1294 = local read "Mean trigger"() -> (w4522:i32)
                n1295 = local read "Sub img mean"() -> (w4521:dbl)
                n1296 = Greater Or Equal?(x=w4521, y=w4522) -> (x >= y?=w4520:bool)
              }
              n1297 = Wait (ms)(milliseconds to wait=u32 500) -> ()  [unwired: 1 out]
            }
            frame #1 {
              w4527 = u8 2 items=["0", "1", "2", "3", "4"] ("Axis Number")
              # "Extra scan"
              n1298 = local read "um to move"() -> (w4523:u32)
              n1299 = call "RS232C_Move.vi"("VISAリソース名"=w4529, "Axis Count"=u8 2, "Axis Number"=w4527, "Pulse Number"=w4523, "Direction"=w4524, "Delimiter"=w4525, "Main/Sub"=FALSE) -> ("OK Done"=w4530:bool)  [unwired: 1 out]
            }
            frame #2 {
              n1300 = local read "Sub img mean"() -> (w4532:dbl)
              n1301 = local read "Mean trigger"() -> (w4533:i32)
              n1302 = Greater?(x=w4532, y=w4533) -> (0:w4531:bool)
            }
          }
          n1303 = call <extravilib>:"Write.vi"("element"=w4511) -> ("channel"=w4512:T13)  [unwired: 1 out]
        }
        n1304 = flat-sequence {
          tunnel: [w4559] -> w4433
          tunnel: [w4560] -> w4443
          tunnel: [w4561] -> w4442
          tunnel: [w4553] -> w4445
          tunnel: w4464 -> [w4559]
          tunnel: w4467 -> [w4560]
          tunnel: w4466 -> [w4561]
          frame #0 {
            w4553 = "\r\n"
            w4555 = u8 2 items=["0", "1", "2", "3", "4"] ("Axis Number")
            n1305 = Wait (ms)(milliseconds to wait=u32 500) -> ()  [unwired: 1 out]
            n1306 = call "RS232C_SetSpeed.vi"("Low Speed"="Acquire speed 3 (um/s)", "High Speed"="Acquire speed 3 (um/s)", "Acceleration Time"=u16 0, "Axis Number"=w4555, "Delimiter"=w4553, "VISAリソース名"=w4559, "Axis Count"=u8 2, "Range"=TRUE, "Main/Sub"=FALSE) -> ()  [unwired: 2 out]
          }
        }
        n1307 = Path To String(path="Save base file name 2000") -> (string=w4458:string)
        n1308 = Concatenate Strings(w4458, w4427) -> (w4457:string)
        n1309 = local read "Last saved file number 2000"() -> (w4423:i32)
        n1310 = String To Path(string=w4457) -> (path=w4410:path)
        "Last saved file 2000" <- w4410
        n1311 = local read "Frames in memory 2"() -> (w4437:i32)
        n1312 = Initialize Array(0.0 ("element"), 200 ("dimension size"), 2048 ("dimension size"), 2048 ("dimension size")) -> (w4414:dbl[][][])
        n1313 = call <userlib>:"tm_startrecorder_40.vi"("error in (no error)"=w4443, "frames"=w4437, "File"=w4410, "Handle in"=w4442) -> ("error out"=w4441:errorcluster, "Handle out"=w4440:u32)  [unwired: 6 in]
        n1314 = Initialize Array(0.0 ("element"), 1000 ("dimension size")) -> (w4389:dbl[])
        n1315 = call <userlib>:"tm_startcapture_40.vi"("error in (no error)"=w4441, "Handle in"=w4440) -> ("error out"=w4439:errorcluster, "Handle out"=w4438:u32)  [unwired: 8 in]
        n1316 = while {
          tunnel: w4438 -> [w4550]
          tunnel: w4439 -> [w4549]
          tunnel: [w4546] -> w4463
          tunnel: [w4545] -> w4462
          tunnel: w4461 -> [w4548]
          tunnel: w4444 -> [w4542]
          shift-right: [w4540] -> w4413
          shift-left: w4414 -> [w4541]
          stop <- w4547 stop-if-true
          # "Camera streaming during acquisition"
          n1317 = call <extravilib>:"Read.vi"("channel"=w4548) -> ("element"=w4547:bool)  [unwired: 1 in, 1 out]
          n1318 = call <userlib>:"tm_waitnextframe_40.vi"("error in (no error)"=w4549, "Handle in"=w4550) -> ("error out"=w4545:errorcluster, "Frame Count"=w4539:i32, "Frame Index"=w4544:i32, "Handle out"=w4546:u32)  [unwired: 6 in]
          n1319 = local write "Frame count"(w4539) -> ()
          n1320 = Index Array(array=w4542, index=w4544) -> (element=w4543:T12)
          n1321 = call "IMAQ ImageToArray"("Image"=w4543) -> ("Image Pixels (U16)"=w4537:u16[][])  [unwired: 3 in, 4 out]
          n1322 = Replace Array Subset(array=w4541, new element=w4537, index (dim 0)=w4539) -> (w4540:dbl[][][])  [unwired: 2 in]
          n1323 = Reshape Array(w4537, 4194304) -> (w4538:u16[])
          n1324 = local write "Obtained image"(w4537) -> ()
          n1325 = call-poly <vilib>:"Mean.vi"("X"=w4538) -> ("mean"=w4536:dbl)  [unwired: 1 out]
          n1326 = local write "Mean intensity\nof frame"(w4536) -> ()
        }
        n1327 = call <userlib>:"tm_stopcapture_40.vi"("error in (no error)"=w4462, "Handle in"=w4463) -> ("error out"=w4459:errorcluster, "Handle out"=w4460:u32)  [unwired: 8 in]
        n1328 = call <userlib>:"tm_stoprecorder_40.vi"("error in (no error)"=w4459, "Handle in"=w4460) -> ("error out"=w4446:errorcluster, "Handle out"=w4447:u32)  [unwired: 8 in]
        n1329 = flat-sequence {
          tunnel: w4448 -> [w4487]
          tunnel: w4450 -> [w4486]
          tunnel: [w4486] -> w4436
          tunnel: [w4487] -> w4435
          tunnel: [w4485] -> w4434
          tunnel: [w4495] -> w4449
          tunnel: w4436 -> [w4495]
          tunnel: w4435 -> [w4491]
          tunnel: w4434 -> [w4494]
          tunnel: w4432 -> [w4489]
          tunnel: w4386 -> [_]
          tunnel: [w4488] -> w4371
          frame #0 {
            w4479 = u8 2 items=["0", "1", "2", "3", "4"] ("Axis Number")
            w4481 = u16 4000 ("Acceleration Time")
            w4485 = "\r\n"
            n1330 = call "RS232C_SetSpeed.vi"("Low Speed"=w4481, "High Speed"=w4481, "Acceleration Time"=u16 0, "Axis Number"=w4479, "Delimiter"=w4485, "VISAリソース名"=w4486, "Axis Count"=u8 2, "Range"=TRUE, "Main/Sub"=FALSE) -> ()  [unwired: 2 out]
          }
          frame #1 {
            w4496 = u8 2 items=["0", "1", "2", "3", "4"] ("Axis Number")
            n1331 = Not(x=w4491) -> (.not. x?=w4490:bool)
            n1332 = Wait (ms)(milliseconds to wait=u32 500) -> ()  [unwired: 1 out]
            n1333 = call "RS232C_Move.vi"("VISAリソース名"=w4495, "Axis Count"=u8 2, "Axis Number"=w4496, "Pulse Number"=w4489, "Direction"=w4490, "Delimiter"=w4494, "Main/Sub"=FALSE) -> ()  [unwired: 2 out]
            n1334 = call <vilib>:"High Resolution Relative Seconds.vi"() -> ("relative seconds"=w4488:dbl)
          }
        }
        n1335 = for {
          tunnel: w4413 -> [w4474] mode=indexing
          tunnel: [w4471] -> w4392 mode=indexing
          tunnel: [w4469] -> _ mode=indexing
          workers-P: _ -> [_]
          tunnel: [w4469] -> w4394 mode=indexing
          n1336 = local read "wave trigger"() -> (w4470:dbl)
          n1337 = Reshape Array(w4474, 4194304 ("dimension size")) -> (w4473:dbl[])
          n1338 = call-poly <vilib>:"Mean.vi"("X"=w4473) -> ("mean"=w4469:dbl)  [unwired: 1 out]
          n1339 = Greater?(x=w4469, y=w4470) -> (0:w4472:bool)
          n1340 = Boolean To (0,1)(Boolean=w4472) -> (0, 1=w4471:i16)
        }
        n1341 = call-poly <vilib>:"Write Waveforms to File.vi"("waveform"=w4392, "file path (dialog if empty)"=w4410) -> ()  [unwired: 8 in, 2 out]
        n1342 = Reverse 1D Array(array=w4392) -> (reversed array=w4409:i16[])
        n1343 = Search 1D Array(1D array=w4392, element=w4368) -> (index of element=w4397:i32)  [unwired: 1 in]
        n1344 = Search 1D Array(1D array=w4409, element=w4368) -> (index of element=w4407:i32)  [unwired: 1 in]
        n1345 = Add(x=w4397, y=w4407) -> (x+y=w4408:i32)
        n1346 = Subtract(x=200, y=w4408) -> (x-y=w4396:i32)
        n1347 = Insert Into Array(array=w4400, index=w4370, new element=w4396) -> (w4401:i16[])
        n1348 = Array Subset(array=w4394, index=w4397, length=w4396) -> (w4398:dbl[])
        n1349 = call-poly <vilib>:"Mean.vi"("X"=w4398) -> ("mean"=w4395:dbl)  [unwired: 1 out]
        n1350 = Insert Into Array(array=w4389, index=w4423, new element=w4395) -> (w4422:dbl[])
        n1351 = case shown="True" w4451 {
          tunnel: [states."auto imaging" w4500] -> w4454
          frame False {
          }
          frame True {
            n1352 = case shown="True" "4000?" {
              tunnel: [states."screening" states."4000"] -> w4500
              frame False {
              }
              frame True {
              }
            }
          }
        }
        n1353 = case shown="True" w4430 {
          tunnel: w4429 -> [w4475 w4478]
          tunnel: [w4475 w4477] -> w4428
          frame False {
          }
          frame True {
            n1354 = local read "Last saved file number 2000"() -> (w4476:i32)
            n1355 = Replace Array Subset(array=w4478, new element=w4476, index=w4476) -> (w4477:dbl[])
          }
        }
        "Last saved file number 2000" <- w4369
      }
      frame "Close" {
        n1356 = call-poly <vilib>:"DAQmx Write.vi"("task/channels in"=w4605, "data"=FALSE) -> ()  [unwired: 11 in, 3 out]
        n1357 = call-poly <vilib>:"DAQmx Write.vi"("task/channels in"=w4607, "data"=FALSE) -> ()  [unwired: 11 in, 3 out]
        n1358 = call <userlib>:"tm_unpreparecapture_40.vi"("error in (no error)"=w4627, "Handle in"=w4628) -> ("error out"=w4630:errorcluster, "Handle out"=w4629:u32)  [unwired: 8 in]
        n1359 = call-poly <vilib>:"DAQmx Write.vi"("task/channels in"=w4606, "data"=FALSE) -> ()  [unwired: 11 in, 3 out]
        n1360 = call <userlib>:"tm_closecamera_40.vi"("error in (no error)"=w4630, "Handle in"=w4629) -> ("error out"=w4631:errorcluster)  [unwired: 9 in]
        n1361 = call <userlib>:"tm_deinitialize_40.vi"("error in (no error)"=w4631) -> ("error out"=→"Camera error out":errorcluster)  [unwired: 10 in]
        n1362 = call <vilib>:"High Resolution Relative Seconds.vi"() -> ("relative seconds"=→"experiment stop time (relative)":dbl)
        n1363 = call-poly <vilib>:"DAQmx Write.vi"("task/channels in"=w4564, "data"=TRUE) -> ()  [unwired: 11 in, 3 out]
        n1364 = invoke class="BenchtopStepperControl" method="CloseDevice"(reference=w4581) -> ()  [unwired: 2 in, 3 out]
        n1365 = flat-sequence {
          tunnel: refnum<visa-resource-name> "USB0::0x1AB1::0x0643::DG9A242400208::INSTR" ("VISA resource name") -> [w4635]
          tunnel: refnum<visa-resource-name> "USB0::0x1AB1::0x0643::DG9A242400205::INSTR" ("VISA resource name") -> [w4634]
          tunnel: [w4634] -> w4598
          tunnel: [w4633] -> w4588
          tunnel: [w4636] -> w4597
          tunnel: w4598 -> [w4638]
          tunnel: [w4638] -> w4596
          tunnel: w4588 -> [w4637]
          tunnel: w4597 -> [w4645]
          tunnel: [w4641] -> w4595
          tunnel: w4596 -> [w4642]
          tunnel: [w4642] -> w4594
          tunnel: w4595 -> [w4647]
          tunnel: [w4647] -> w4593
          tunnel: w4594 -> [w4649]
          tunnel: [w4646] -> w4592
          tunnel: w4593 -> [w4651]
          tunnel: [w4651] -> w4591
          tunnel: w4592 -> [w4653]
          tunnel: [w4650] -> w4590
          tunnel: w4591 -> [w4658]
          tunnel: [w4658] -> w4589
          tunnel: w4590 -> [w4659]
          tunnel: [w4656] -> w4587
          tunnel: w4589 -> [w4662]
          tunnel: w4587 -> [w4660]
          frame #0 {
            # "CONNECT"
            n1366 = VISA Open(VISA resource name=w4635) -> (VISA resource name=w4633:refnum<visa-resource-name>)  [unwired: 4 in, 1 out]
          }
          frame #1 {
            n1367 = VISA Write(VISA resource name=w4637, write buffer=":OUTP2 OFF") -> (VISA resource name out=w4636:refnum<visa-resource-name>)  [unwired: 1 in, 2 out]
            n1368 = Wait (ms)(milliseconds to wait=u32 500) -> ()  [unwired: 1 out]
          }
          frame #2 {
            n1369 = VISA Write(VISA resource name=w4645, write buffer=":OUTP1 OFF") -> (VISA resource name out=w4641:refnum<visa-resource-name>)  [unwired: 1 in, 2 out]
            n1370 = Wait (ms)(milliseconds to wait=u32 500) -> ()  [unwired: 1 out]
          }
          frame #3 {
            n1371 = VISA Open(VISA resource name=w4649) -> (VISA resource name=w4646:refnum<visa-resource-name>)  [unwired: 4 in, 1 out]
            n1372 = Wait (ms)(milliseconds to wait=u32 500) -> ()  [unwired: 1 out]
          }
          frame #4 {
            n1373 = VISA Write(VISA resource name=w4653, write buffer=":OUTP2 OFF") -> (VISA resource name out=w4650:refnum<visa-resource-name>)  [unwired: 1 in, 2 out]
            n1374 = Wait (ms)(milliseconds to wait=u32 500) -> ()  [unwired: 1 out]
          }
          frame #5 {
            n1375 = VISA Write(VISA resource name=w4659, write buffer=":OUTP1 OFF") -> (VISA resource name out=w4656:refnum<visa-resource-name>)  [unwired: 1 in, 2 out]
            n1376 = Wait (ms)(milliseconds to wait=u32 500) -> ()  [unwired: 1 out]
          }
          frame #6 {
            n1377 = VISA Clear(VISA resource name=w4662) -> ()  [unwired: 1 in, 2 out]
            n1378 = VISA Clear(VISA resource name=w4660) -> ()  [unwired: 1 in, 2 out]
            n1379 = Wait (ms)(milliseconds to wait=u32 500) -> ()  [unwired: 1 out]
          }
          frame #7 {
          }
        }
      }
      frame "Stop" {
        w4711 = FALSE
        n1380 = local read "experiment stop time (relative)"() -> (w4681:dbl)
        n1381 = local read "relative seconds start"() -> (w4680:dbl)
        n1382 = invoke class="VI" method="Abort VI"(reference=w4671) -> ()  [unwired: 2 in, 3 out]
        n1383 = Subtract(x=w4681, y=w4680) -> (x-y=w4679:dbl)
        n1384 = Divide(x=w4679, y=60.0) -> (x/y=w4675:dbl)
        "experiment time(mins)" <- w4675
        n1385 = Greater?(x=w4675, y=5.0) -> (0:w4677:bool)
        n1386 = case shown="True" w4677 {
          tunnel: w4674 -> [_ w4760]
          frame False {
          }
          frame True {
            w4741 = "15528131356@163.com" ("username")
            w4754 = "\\" ("string")
            # "email system"
            n1387 = local read "Save directory"() -> (w4758:path)
            n1388 = local read "Last saved #"() -> (w4776:i32)
            n1389 = local read "experiment time(mins)"() -> (w4768:dbl)
            n1390 = Increment(x=w4776) -> (x+1=w4767:i32)
            n1391 = Path To String(path=w4758) -> (string=w4757:string)
            n1392 = Number To Decimal String(number=w4767) -> (decimal integer string=w4775:string)  [unwired: 1 in]
            n1393 = Divide(x=w4767, y=w4768) -> (x/y=w4766:dbl)
            n1394 = Number To Decimal String(number=w4768, width (-)=i16 4) -> (decimal integer string=w4778:string)
            n1395 = Number To Decimal String(number=w4766) -> (decimal integer string=w4765:string)  [unwired: 1 in]
            n1396 = case shown="\"hanqing WANG\", Default" "Operator" {
              tunnel: [string[] ["ktsubasa@g.ecc.u-tokyo.ac.jp"] ("to") string[] ["hu-chenglang@g.ecc.u-tokyo.ac.jp"] ("to") string[] ["gabrielwangld@gmail.com"] ("cc") string[] ["223yuya@g.ecc.u-tokyo.ac.jp"] ("cc")] -> w4734
              frame "kobayashi" {
              }
              frame "chenglang" {
              }
              frame "hanqing WANG", Default {
              }
              frame "Tsutsumi" {
              }
            }
            n1397 = Concatenate Strings("Experiment time:" ("string"), w4778, w4754, "Sample number:" ("string"), w4775, "/Throughput:" ("string"), w4765, "" ("string"), "real laser power:" ("string"), "real laser power", "sample name:" ("string"), w4760, "saving directory:" ("string"), w4757, "clearing date:" ("string"), "clearing date", w4754) -> (w4742:string)
            n1398 = Get Date/Time String() -> (date string=w4773:string, time string=w4770:string)  [unwired: 3 in]
            n1399 = Concatenate Strings("smtp.163.com" ("string"), ":" ("string"), "25" ("string")) -> (w4737:string)
            n1400 = call <vilib>:"Open Handle.vi"("server address"=w4737, "from"=w4741, "username"=w4741, "password"="element1010") -> ("handle out"=w4753:T14, "error out"=w4752:errorcluster)  [unwired: 10 in]
            n1401 = call <vilib>:"Set Recipients.vi"("handle in"=w4753, "to"=w4734, "cc"=string[] ["pteamcalendar@gmail.com"], "error in (no error)"=w4752) -> ("handle out"=w4751:T14, "error out"=w4750:errorcluster)  [unwired: 10 in]
            n1402 = Concatenate Strings("Experiment record_" ("Subject"), w4773, "_" ("string"), w4770) -> (w4743:string)
            n1403 = call-poly <vilib>:"Set Message.vi"("handle in"=w4751, "subject"=w4743, "plain text message"=w4742, "error in (no error)"=w4750) -> ("handle out"=w4749:T14, "error out"=w4748:errorcluster)  [unwired: 10 in]
            n1404 = call <vilib>:"Set Attachments.vi"("handle in"=w4749, "error in (no error)"=w4748) -> ("handle out"=w4747:T14, "error out"=w4746:errorcluster)  [unwired: 12 in]
            n1405 = call <vilib>:"Send.vi"("handle in"=w4747, "error in (no error)"=w4746) -> ("handle out"=w4745:T14, "error out"=w4744:errorcluster)  [unwired: 11 in, 1 out]
            n1406 = call <vilib>:"Close Handle.vi"("handle in"=w4745, "error in (no error)"=w4744) -> ()  [unwired: 12 in, 2 out]
          }
        }
        n1407 = call-poly <vilib>:"DAQmx Write.vi"("task/channels in"=w4712, "data"=w4711, "error in"=w4698) -> ("task out"=w4702:refnum<k21>, "error out"=w4697:errorcluster)  [unwired: 10 in, 1 out]
        n1408 = call-poly <vilib>:"DAQmx Write.vi"("task/channels in"=w4715, "data"=w4711, "error in"=w4714) -> ("task out"=w4704:refnum<k21>, "error out"=w4699:errorcluster)  [unwired: 10 in, 1 out]
        n1409 = call <vilib>:"DAQmx Stop Task.vi"("task/channels in"=w4702, "error in"=w4697) -> ("task out"=w4706:refnum<k21>, "error out"=w4705:errorcluster)  [unwired: 12 in]
        n1410 = call <vilib>:"DAQmx Clear Task.vi"("task in"=w4706, "error in"=w4705) -> ()  [unwired: 13 in, 1 out]
        n1411 = call-poly <vilib>:"DAQmx Write.vi"("task/channels in"=w4713, "data"=w4711, "error in"=w4701) -> ("task out"=w4703:refnum<k21>, "error out"=w4700:errorcluster)  [unwired: 10 in, 1 out]
        n1412 = call <vilib>:"DAQmx Stop Task.vi"("task/channels in"=w4704, "error in"=w4699) -> ("task out"=w4708:refnum<k21>, "error out"=w4707:errorcluster)  [unwired: 12 in]
        n1413 = call <vilib>:"DAQmx Stop Task.vi"("task/channels in"=w4703, "error in"=w4700) -> ("task out"=w4710:refnum<k21>, "error out"=w4709:errorcluster)  [unwired: 12 in]
        n1414 = call <vilib>:"DAQmx Clear Task.vi"("task in"=w4708, "error in"=w4707) -> ()  [unwired: 13 in, 1 out]
        n1415 = call <vilib>:"DAQmx Clear Task.vi"("task in"=w4710, "error in"=w4709) -> ()  [unwired: 13 in, 1 out]
      }
    }
    "Larvae until move" <- w127
    "Auto-imaging time" <- w110
    "tube changing #" <- w101
    n1416 = Format Into String(w73) -> (resulting string=→"Current state":string)  [unwired: 3 in, 1 out]
    "4c label #" <- w97
  }
  n1417 = flat-sequence {
    tunnel: w47 -> [w4791]
    tunnel: w37 -> [w4789]
    tunnel: w29 -> [w4786]
    tunnel: w13 -> [w4785]
    frame #0 {
      n1418 = call <vilib>:"DAQmx Stop Task.vi"("task/channels in"=w4785) -> ("task out"=w4784:refnum<k21>)  [unwired: 13 in, 1 out]
      n1419 = call <vilib>:"DAQmx Stop Task.vi"("task/channels in"=w4789) -> ("task out"=w4788:refnum<k21>, "error out"=w4787:errorcluster)  [unwired: 13 in]
      n1420 = VISA Clear(VISA resource name=w4786) -> ()  [unwired: 1 in, 2 out]
      n1421 = Index Array(array=w4791, index=1500) -> (element=w4792:T12)
      n1422 = call <vilib>:"DAQmx Clear Task.vi"("task in"=w4784) -> ()  [unwired: 14 in, 1 out]
      n1423 = call "IMAQ Dispose"("All Images? (No)"=TRUE, "Image"=w4792) -> ()  [unwired: 4 in, 1 out]
      n1424 = call <vilib>:"DAQmx Clear Task.vi"("task in"=w4788, "error in"=w4787) -> ()  [unwired: 13 in, 1 out]
    }
  }
